vi "AlliGator.vi"() -> ()   [LabVIEW 2021, in "AlliGator GUI.lvlib"]
doc: "AlliGator main window.\nSpawned by AlliGator Launcher.vi.\nSpawns AlliGator Action Loop.vi, which handles UI requests from AlliGator.vi"
uses:
  AlliGator GUI.lvlib
  AlliGator Main Window Tabs.ctl
  Phasor/Phasor (g, s).ctl
  AlliGator Displayed Image.ctl
  AlliGator State Indicator.ctl
  Phasor/Phasor (m, phi).ctl
  Phasor/Phasor Ratio Type.ctl
  Fits/IRF(X)PSED/Decay Fit Parameters & Derived Quantities List.ctl
  Phasor/Phasor Calibration Type.ctl
  Histograms/Linear Histogram Options.ctl
  Histograms/Histogram Bin Option.ctl
  Histograms/Histogram Bin Position.ctl
  AlliGator Q Element.ctl
  AlliGator Q Event.ctl
  AlliGator Dataset Ctrl Refnums.ctl
  AlliGator Other Ctrl Refnums.ctl
  AlliGator Registered Events Ctrl Refnums.ctl
  AlliGator Ctrl Refnums.ctl
  AlliGator Phasor Plot Ctrl Refnums.ctl
  AlliGator Phasor Graph Ctrl Refnums.ctl
  AlliGator Image Histogram Control Refnums.ctl
  AlliGator Decay Fit Map Control Refnums.ctl
  AlliGator Refnums List.ctl
  AlliGator Settings List.ctl
  AlliGator Variables List.ctl
  Palette/Image Palette Information.ctl
  Image/Image Display Palette Type.ctl
  Image/Image Display Event.ctl
  Image/Image Control Refnum.ctl
  <vilib>/Utility/miscctls.llb/LVPoint32TypeDef.ctl
  AlliGator Decay Parameter Map Update Event Data.ctl
  Graphs/XY Graph/XY Graph Event.ctl
  AlliGator Filtered Event Data.ctl
  Utilities/Read-Write.ctl
  Graphs/XY Graph/New Plot Information.ctl
  Graphs/Plot Scales.ctl
  Graphs/LabVIEW Plot Interpolation.ctl
  Graphs/Plot Point Style.ctl
  Graphs/XY Graph/XY Graph Mouse Click Event Data.ctl
  Graphs/XY Graph/XY Graph Refnum.ctl
  AlliGator ROI Manager Actions.ctl
  Image/Image Display User Event Data.ctl
  AlliGator Phasor Plot Mouse Up Event Data.ctl
  Image/Image ROI Descriptor.ctl
  Image/Image Contour Definition.ctl
  Image/Image Contour ID.ctl
  Image/Image ROI Type.ctl
  AlliGator Action Loop.vi
  Variant/Variant to Data/Variant to Boolean.vi
  Phasor/Phasor Abort Parallel Computation.vi
  Fits/Abort Fit Global.vi
  Image/Abort ROI Creation Global.vi
  AlliGator Abort.vi
  Variant/Variant to Data/Variant to [String].vi
  <vilib>/Utility/inputDevices.llb/keyboardAcquire.vi
  <vilib>/Utility/inputDevices.llb/mouseAcquire.vi
  AlliGator Globals.vi
  <vilib>/Utility/inputDevices.llb/closeKeyboard.vi
  <vilib>/Utility/inputDevices.llb/closeMouse.vi
  AlliGator Action Engine.lvlib
  Variant/Variant to Data/Variant to Data.lvlib
  Error/Error.lvlib
  AlliGator Globals, Variables & Constants.lvlib
  Image/Image.lvlib
  Palette/Palette.lvlib
  Notebook/Notebook.lvlib
  Rich Text Box/Rich Text Box.lvlib
  Graphs/XY Graph/XY Graph Add-Ons.lvlib
  AlliGator Settings.lvlib
  Phasor/Phasor.lvlib
  Fits/Fits.lvlib
  AlliGator Phasor Calibration.lvlib
  AlliGator Phasor Plot.lvlib
  AlliGator Source Image.lvlib
  AlliGator Phasor Graph.lvlib
  AlliGator ROIs.lvlib
  GUI/GUI.lvlib
  AlliGator Decay Fit Parameter Map.lvlib
  AlliGator Python Plugins.lvlib
  Utilities/Utilities.lvlib
  AlliGator Graphs.lvlib
  Sound/Sound.lvlib
  Graphs/Graphs.lvlib
  AlliGator Decay Processing.lvlib
  Histograms/Histogram Window.lvlib
panel:
  in  "Current ROI Analysis":bool
  in  "Scale Bar":bool
  in  "Refresh Image":bool
  in  "Clear Image Overlay":bool
  in  "Overlay Mode":u16(ring)
  in  "Use ROI as Search Area":bool
  in  "Highlight Image ROI":bool
  in  "Phasor Overlay Color":u32(colorbox)=16777216
  in  "Gate Image Slide":u16(slide)=9 min=1 max=135 scale=1.0..132.0
  in  "Dataset File/Folder Path":path caption="File/Folder Path"
  out "Source Image":T1(plugin-control)
  in  "Source Image ROI Selection":i32(c297)
  in  "Source Image ROI Color":u32(colorbox)=6618880 caption="ROI Color"
  in  "Time Point Slide":u16(slide)=65535 min=1 step=1 scale=1.0..2.0
  in  "Image Color Scale":dbl(ramp)
  in  "Channel Name":u16(ring) items=["Gate"]
  out "Current Time Stamp":dbl caption="Time Stamp" format="%#_5g"
  out "CPU":dbl[unit] format="%^#_4e"
  in  "Save Source Image":bool caption="Save Image"
  out "Current Data":string="Stained cancer cells" caption="Current Folder"
  in  "Displayed Image":T2=enum."Sum of All Gates"
  in  "Tab Control":T3=enum."Lifetime & Other Parameters"
  in  "Dataset File/Folder Path 2":path caption="File/Folder Path"
  in  "Histogram Lower Percentile":dbl=1.0 caption="Lower Percentile" min=0.0 max=100.0 format="%#.3f"
  in  "Histogram Upper Percentile":dbl=1.0 caption="100 - Upper Percentile" min=0.0 max=100.0 format="%#.3f"
  in  "Image Histogram Options":T4={"Bin Size"=1.0, "Bin Number"=256, "Bin Option"=enum."Bin Number", "Min Value"=-inf, "Max Value"=inf, "Filter NaN & Infinite Values"=TRUE, "Frequency Plot"=FALSE, "Align Bins"=TRUE, "Bin Location"=enum."Left", "Project Outside Values"=FALSE, "Max Histogram Size"=1000000} {"Max Histogram Size" format="%.0e"}
  in  "Auto-Adjust Contrast":bool=TRUE
  out "Lower Percentile":dbl=nan format="%#.3f"
  out "Upper Percentile":dbl=nan caption="100 - Upper Percentile" format="%#.3f"
  in  "Image Histogram Active":bool=TRUE
  in  "Use Image Histogram for Contrast":bool=TRUE
  out "Image Histogram":cluster{"X Array":dbl[], "Y Array":dbl[]}[](graph)
  in  "Dataset File/Folder Path 3":path caption="File/Folder Path"
  out "Decay Integrated Intensity":dbl=46949635.0 caption="Bkgd-subtracted Intensity" format="%#_5g"
  out "Decay Background":dbl caption="Background" format="%#_5g"
  out "Decay Lifetime":dbl[unit] caption="Lifetime" format="%#_5g"
  out "Decay Graph TipStrip":string
  out "Decay Graph":cluster{"X Array":dbl[], "Y Array":dbl[]}[](graph)
  in  "Decay Graph Active":bool=TRUE
  in  "Dataset File/Folder Path 4":path caption="File/Folder Path"
  out "Decay Statistics Graph TipStrip":string
  out "Decay Statistics Graph":cluster{"X Array":dbl[], "Y Array":dbl[]}[](graph)
  in  "Decay Statistics Bin":i32=1 min=1
  in  "Dataset File/Folder Path 5":path caption="File/Folder Path"
  in  "Intensity Correction File":path
  in  "Use Intensity Correction File":bool
  out "Intensity Time Trace TipStrip":string
  in  "Use File Timestamp":bool=TRUE
  out "Intensity Time Trace":cluster{"X Array":dbl[], "Y Array":dbl[]}[](graph)
  in  "Time Step":dbl[unit]=1.0 format="%#_5g"
  in  "Dataset File/Folder Path 6":path caption="File/Folder Path"
  in  "Phasor ROI Decay":bool
  in  "Phasor Plot ROI Color":u32(colorbox)=6618880
  out "Phasor Plot Average Lifetime":dbl[unit]=nan caption="<tau>_a" format="%#_4e"
  out "Phasor Plot Phasor Ratio":dbl=nan caption="Amplitude Ratio (a1)" format="%#_4e"
  out "Phasor Plot Modulus Lifetime":dbl[unit]=nan caption="Modulus Lifetime" format="%#_4e"
  out "Phasor Plot Phase Lifetime":dbl[unit]=-9.431404035075279e-09 caption="Phase Lifetime" format="%#_4e"
  out "Phasor at cursor (m, phi)":T7={"m"=1.5330078000581284, "phi"=1.7786862539971595} caption="Phasor at Cursor (m, phi)" {"phi" format="%#_4e"; "m" format="%#_4e"}
  in  "Clear Phasor Overlay":bool
  in  "Phasor Plot ROI Selection":i32(c297)
  in  "Phasor Plot Active":bool
  in  "Phasor Plot Color Scale":dbl(ramp)
  out "Phasor at cursor (g, s)":T8={"g"=-0.31640625, "s"=1.5} caption="Phasor at Cursor" {"s" format="%#.3e"; "g" format="%#_4e"}
  in  "Phasor Plot Display Range":cluster{u32, u32}(slide)={0, 100} scale=0.0..6117.0
  in  "Highlight Phasor in Source Image":bool caption="Highlight Phasor ROI"
  in  "Image Overlay Color":u32(colorbox)=16777216
  out "Phasor Plot Image":T1(plugin-control)
  in  "Refresh Phasor Plot":bool caption="Refresh Phsor Plot"
  in  "Save Phasor Plot":bool
  out "Reference 2 Button":bool caption="Reference"
  out "Reference 1 Button":bool caption="Reference"
  in  "Phasor Plot Frequency":dbl[unit]=80000000.0 caption="Phasor Frequency"
  in  "Dataset File/Folder Path 7":path caption="File/Folder Path"
  out "Average Lifetime SDV":dbl[unit]=nan caption="+/-" format="%#.3g"
  out "Phasor Ratio SDV":dbl=nan caption="+/-" format="%#.3g"
  out "Modulus Lifetime SDV":dbl[unit]=nan caption="+/-" format="%#.3g"
  out "Phase Lifetime SDV":dbl[unit]=nan caption="+/-" format="%#.3g"
  in  "Calibration Type":T9
  out "Phasor Graph Average Lifetime":dbl[unit]=nan caption="<tau>_a" format="%#.3g"
  in  "Phasor Graph Active":bool
  in  "Refresh SEPL":bool
  out "Phasor Graph Phasor Ratio":dbl=nan caption="Amplitude Ratio (a1)" format="%#.3g"
  out "Phasor Graph Modulus Lifetime":dbl[unit]=nan caption="Modulus Lifetime" format="%#.3g"
  in  "Phasor Reference 2 Control":dbl(c297)
  in  "Save Phasor Graph Image":bool
  in  "Current Phasor (m, phi)":T7={"m"=nan, "phi"=nan} {"phi" format="%#_4g"; "m" format="%#_4g"}
  in  "Phasor Reference 1 Control":dbl(c297)
  out "Phasor Graph TipStrip":string
  in  "Single Step Phasor":bool
  in  "Phasor Frame Slide":i32(slide) caption="Phasor Frame Slider" min=0 step=1 scale=1.0..1.1
  out "Phase Lifetime 2":dbl[unit]=nan format="%#.3g"
  out "Phase Lifetime 1":dbl[unit]=nan format="%#.3g"
  in  "Show Line":bool
  out "Phasor Graph Phase Lifetime":dbl[unit]=nan caption="Phase Lifetime" format="%#.3g"
  in  "Current Phasor (g, s)":T8={"g"=nan, "s"=nan} caption="Current Phasor" {"s" format="%#_4g"; "g" format="%#_4g"}
  out "Phasor Graph":cluster{"X Array":dbl[], "Y Array":dbl[]}[](graph)
  in  "Phasor Graph Frequency":dbl[unit]=80000000.0 caption="Phasor Frequency"
  in  "Calibration Lifetime":dbl[unit] min=0.0
  in  "Dataset File/Folder Path 8":path caption="File/Folder Path"
  in  "Phasor Ratio Type":T10
  out "Phasor Ratio Graph TipStrip":string
  out "Phasor Ratio Graph":cluster{"X Array":dbl[], "Y Array":dbl[]}[](graph)
  in  "Dataset File/Folder Path 9":path caption="File/Folder Path"
  out "Lifetime & Other Parameters Graph TipStrip":string caption="Lifetime Graph TipStrip"
  out "Lifetime & Other Parameters Graph":cluster{"X Array":dbl[], "Y Array":dbl[]}[](graph)
  in  "Dataset File/Folder Path 10":path caption="File/Folder Path"
  in  "Decay Fit Parameter Map ROI Color":u32(colorbox)=6618880
  in  "Overlay Decay Fit Parameter Map":bool caption="Overlay Parameter Map"
  out "Decay Fit Max Parameter":dbl=1.0 caption="Max Parameter"
  out "Decay Fit Min Parameter":dbl caption="Min Parameter"
  in  "Refresh Decay Fit Parameter Map":bool
  in  "Decay Fit Parameter":T11
  out "Decay Fit Parameter Map Image":T1(plugin-control)
  in  "Decay Fit Parameter Map Color Scale":dbl(ramp)
  in  "Decay Fit Parameter Map Display Range":cluster{dbl, dbl}(slide)={0.0, 1.0} scale=0.0..1.0
  in  "Map Set":u16(ring)
  in  "Map Parameter":u16(ring)
  in  "Dataset File/Folder Path 11":path caption="File/Folder Path"
  in  "Parameter Map ROI Color":u32(colorbox)=6618880 caption="Decay Fit Parameter Map ROI Color"
  in  "Overlay Parameter Map":bool
  out "Map Max Parameter":dbl=1.0 caption="Max Parameter"
  out "Map Min Parameter":dbl caption="Min Parameter"
  in  "Refresh Parameter Map":bool
  out "Parameter Map Image":T1(plugin-control)
  in  "Parameter Map Color Scale":dbl(ramp)
  in  "Parameter Map Display Range":cluster{dbl, dbl}(slide)={0.0, 1.0} scale=0.0..1.0
  out "Event LED":bool
  out "Message":string
  out "Progress Bar":dbl(slide) scale=0.0..100.0
  in  "Abort ROI Creation":bool
  in  "Abort Fit":bool
  in  "Abort":bool
  out "Animated Busy Icon":bool=TRUE
  out "State Indicators":T12
  # "Drop the content of this VI on AlliGator's diagram\nIn AlliGator, replace the subVI template by a new version"
  # "Drop the content of this VI on AlliGator's diagram\nIn AlliGator, replace the subVI template by a new version"
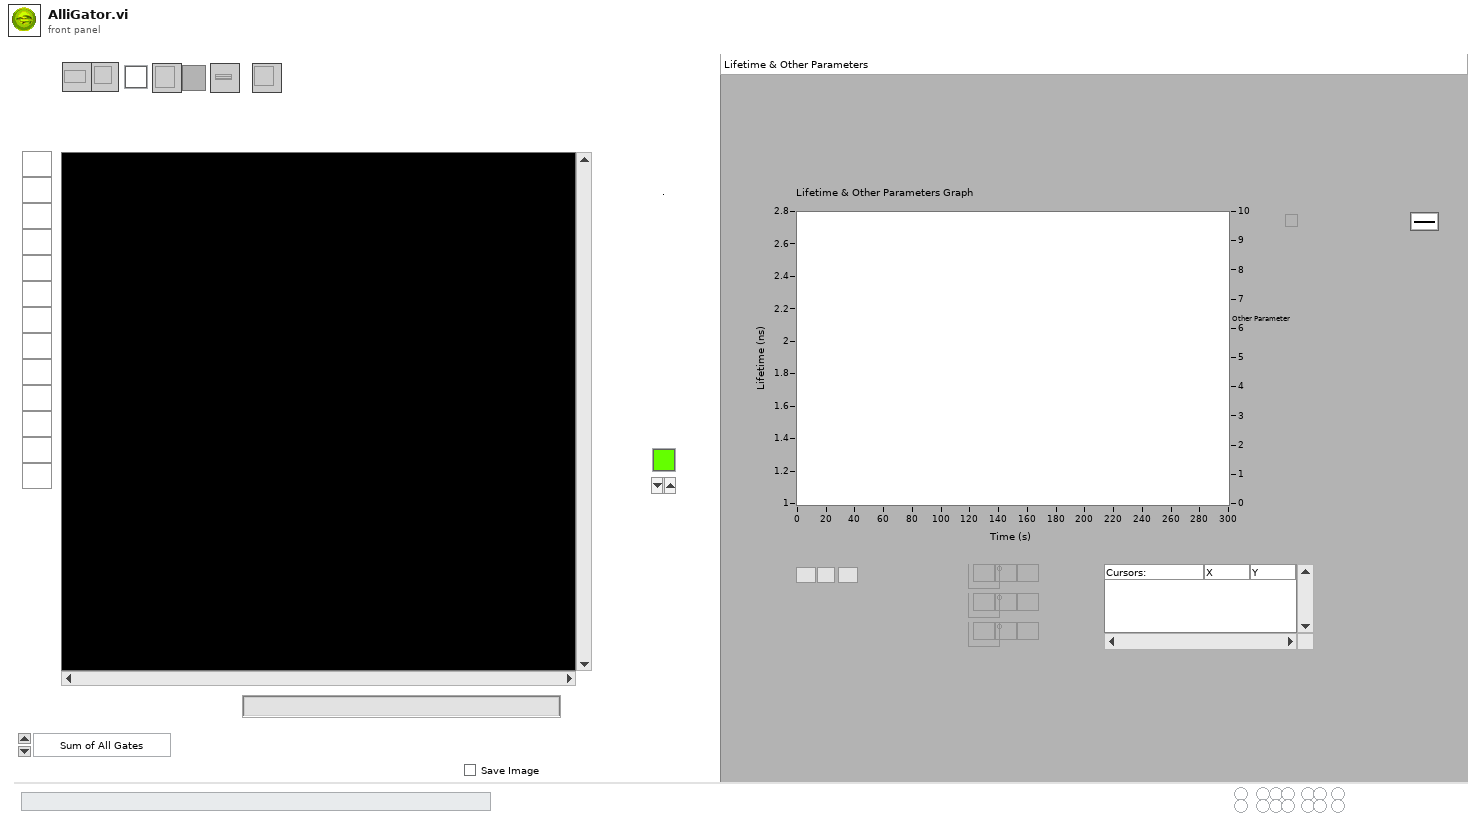
[diagram p1: front panel]
types:
  T1 = typedef "IMAQ Image.ctl" = refnum<image>
  T2 = typedef "AlliGator Source Image.lvlib/AlliGator Displayed Image.ctl" = enum16{"Single Gate", "Sum of All Gates", "Max of All Gates", "Min of All Gates", "-", "White Ligth Image", "Mask Image"}
  T3 = typedef "AlliGator GUI.lvlib/AlliGator Main Window Tabs.ctl" = enum32{"Image Histogram", "Fluorescence Decay", "Fluorescence Decay Statistics", "Intensity Time Trace", "Phasor Plot", "Phasor Graph", "Phasor Ratio", "Lifetime & Other Parameters", "Decay Fit Parameter Map", "Parameter Map"}
  T4 = typedef "Histogram Window.lvlib/Linear Histogram Options.ctl" = cluster{"Bin Size":dbl, "Bin Number":i32, "Bin Option":T5, "Min Value":dbl, "Max Value":dbl, "Filter NaN & Infinite Values":bool, "Frequency Plot":bool, "Align Bins":bool, "Bin Location":T6, "Project Outside Values":bool, "Max Histogram Size":i32}
  T5 = typedef "Histogram Window.lvlib/Histogram Bin Option.ctl" = enum32{"Bin Number", "Bin Size"}
  T6 = typedef "Histogram Window.lvlib/Histogram Bin Position.ctl" = enum16{"Left", "Center", "Right"}
  T7 = typedef "Phasor.lvlib/Phasor (m, phi).ctl" = cluster{"m":dbl, "phi":dbl}
  T8 = typedef "Phasor.lvlib/Phasor (g, s).ctl" = cluster{"g":dbl, "s":dbl}
  T9 = typedef "Phasor.lvlib/Phasor Calibration Type.ctl" = enum16{"None", "Single Phasor", "Phasor Series", "Phasor Map"}
  T10 = typedef "Phasor.lvlib/Phasor Ratio Type.ctl" = enum32{"Intensity-weighted", "Amplitude-weighted"}
  T11 = typedef "Fits.lvlib/Decay Fit Parameters & Derived Quantities List.ctl" = enum16{"Offset", "Baseline", "A_1", "tau_1", "A_2", "tau_2", "<tau>_a", "f1_a", "f2_a", "<tau>_i", "f1_i", "f2_i", "-", "R^2", "Chi^2"}
  T12 = typedef "AlliGator GUI.lvlib/AlliGator State Indicator.ctl" = cluster{"Phasor Calibration Defined":bool, "Phasor Calibration Series Defined":bool, "Phasor Calibration Map Defined":bool, "Phasor Ratio Reference 1 Defined":bool, "Phasor Ratio Reference 2 Defined":bool, "Phasor Ratio Lifetime Reference 1 Defined ":bool, "Phasor Ratio Lifetime Reference 2 Defined":bool, "Phasor Calibration Used":bool, "Phasor Calibration Series Used":bool, "Phasor Calibration Map Used":bool, "Dataset Update Needed":bool, "Phasor Plot Update Needed":bool, "Reference/IRF Defined":bool, "Individual IRFs Defined":bool}
  T13 = enum32{"Invalid", "Standard", "Closed", "Hidden", "Minimized", "Maximized"}
  T14 = enum32{"Image Histogram", "Fluorescence Decay", "Fluorescence Decay Statistics", "Intensity Time Trace", "Phasor Plot", "Phasor Graph", "Phasor Ratio", "Lifetime & Other Parameters", "Decay Fit Parameters Map", "Parameter Map"}
  T15 = typedef "AlliGator Decay Fit Parameter Map.lvlib/AlliGator Decay Fit Map Control Refnums.ctl" = cluster{"Decay Fit Parameter Map Color Scale":refnum<vi>, "Decay Fit Parameter":refnum<vi>, "Max Parameter":refnum<vi>, "Min Parameter":refnum<vi>, "Decay Fit Parameter Map Display":refnum<vi>, "Decay Fit Parameter Map Display Range":refnum<vi>}
  T16 = typedef "AlliGator GUI.lvlib/AlliGator Image Histogram Control Refnums.ctl" = cluster{"Image Histogram":refnum<vi>, "Image Histogram Options":refnum<vi>, "Image Histogram Active":refnum<vi>, "Image Histogram Upper Percentile":refnum<vi>, "Image Histogram Lower Percentile":refnum<vi>, "Auto-Adjust Contrast":refnum<vi>}
  T17 = typedef "AlliGator GUI.lvlib/AlliGator Phasor Graph Ctrl Refnums.ctl" = cluster{"Phasor Ratio":refnum<vi>, "Modulus Lifetime":refnum<vi>, "Phasor at cursor (m, phi)":refnum<vi>, "Phase Lifetime":refnum<vi>, "Phasor at cursor (g, s)":refnum<vi>, "Phasor Graph Average Lifetime":refnum<vi>, "Phasor Graph Active":refnum<vi>, "Save Phasor Graph":refnum<vi>, "Phasor Frame Slide":refnum<vi>, "Single Step Phasor":refnum<vi>, "Calibration Type":refnum<vi>, "Show Line":refnum<vi>, "Phase Lifetime 1":refnum<vi>, "Phase Lifetime 2":refnum<vi>, "Phasor Graph Frequency":refnum<vi>, "Phasor Reference 1 Control":refnum<vi>, "Phasor Reference 2 Control":refnum<vi>, "Calibration Lifetime":refnum<vi>, "Phase Lifetime SDV":refnum<vi>, "Average Lifetime SDV":refnum<vi>, "Phasor Ratio SDV":refnum<vi>, "Modulus Lifetime SDV":refnum<vi>}
  T18 = typedef "AlliGator GUI.lvlib/AlliGator Phasor Plot Ctrl Refnums.ctl" = cluster{"Phasor Ratio":refnum<vi>, "Modulus Lifetime":refnum<vi>, "Phasor at cursor (m, phi)":refnum<vi>, "Phase Lifetime":refnum<vi>, "Phasor at cursor (g, s)":refnum<vi>, "Phasor Plor Average Lifetime":refnum<vi>, "Phasor Plot Active":refnum<vi>, "Save Phasor Plot":refnum<vi>, "Image Overlay Color":refnum<vi>, "Phasor Plot Color Scale":refnum<vi>, "Reference 1 Button":refnum<vi>, "Reference 2 Button":refnum<vi>}
  T19 = typedef "AlliGator Globals, Variables & Constants.lvlib/AlliGator Refnums List.ctl" = enum16{"---------- AlliGator Controls ----------", "AlliGator Tab Control Refnum", "---------- AlliGator Indicators ----------", "Source Image Display Refnum", "Phasor Plot Display Refnum", "Decay Fit Parameter Map Refnum", "---------- AlliGator VIs ----------", "AlliGator Settings Refnum", "AlliGator Launcher Refnum"}
  T20 = typedef "AlliGator GUI.lvlib/AlliGator Ctrl Refnums.ctl" = cluster{"Other AlliGator Ctrl Refnums":T21, "Phasor Plot Ctrl Refnums":T18, "Phasor Graph Ctrl Refnums":T17, "Dataset Control References":T22, "Registered Events Ctrl Refnums":T23, "Image Histogram Ctrl Refnums":T16, "Decay Fit Map Ctrl Refums":T15}
  T21 = typedef "AlliGator GUI.lvlib/AlliGator Other Ctrl Refnums.ctl" = cluster{"State Indicators":refnum<vi>, " Progress Bar":refnum<vi>, "Decay Graph Active":refnum<vi>, "Decay Statistics Bin":refnum<vi>, "Time Step":refnum<vi>, "Use File Timestamp":refnum<vi>, "Tab Control":refnum<vi>, "CPU":refnum<vi>, "Abort Fit":refnum<vi>, "Dataset File/Folder Path":refnum<vi>, "Abort ROI Creation":refnum<vi>, "Event LED":refnum<vi>, "Dataset File/Folder Path 2":refnum<vi>, "Dataset File/Folder Path 3":refnum<vi>, "Dataset File/Folder Path 4":refnum<vi>, "Dataset File/Folder Path 5":refnum<vi>, "Dataset File/Folder Path 6":refnum<vi>, "Dataset File/Folder Path 7":refnum<vi>, "Dataset File/Folder Path 8":refnum<vi>, "Dataset File/Folder Path 9":refnum<vi>, "Dataset File/Folder Path 10":refnum<vi>, "Dataset File/Folder Path 11":refnum<vi>}
  T22 = typedef "AlliGator GUI.lvlib/AlliGator Dataset Ctrl Refnums.ctl" = cluster{"Current Data":refnum<vi>, "Gate Image Slide":refnum<vi>, "Time Point Slide":refnum<vi>, "Current Time Stamp":refnum<vi>, "Save Image":refnum<vi>, "Displayed Image":refnum<vi>, "Overlay Mode":refnum<vi>, "Phasor Overlay Color":refnum<vi>, "Image Color Scale":refnum<vi>, "Use ROI as Search Area":refnum<vi>, "Source Image ROI Color":refnum<vi>}
  T23 = typedef "AlliGator GUI.lvlib/AlliGator Registered Events Ctrl Refnums.ctl" = cluster{"Time Point Slider":refnum<vi>, "Phasor Plot Display Range":refnum<vi>, "Decay Graph":refnum<vi>, "Decay Statistics Graph":refnum<vi>, "Intensity Time Trace":refnum<vi>, "Phasor Graph":refnum<vi>, "Phasor Ratio Graph":refnum<vi>, "Lifetime Graph":refnum<vi>, "Phasor Plot Display":refnum<vi>, "Source Image Display":refnum<vi>, "Decay Fit Parameter Map Display Range":refnum<vi>, "Decay Fit Parameter Map Display":refnum<vi>}
  T24 = typedef "AlliGator Action Engine.lvlib/AlliGator Q Event.ctl" = enum16{"---- Files ----", "Files:Set Batch Export Files To Save", "Files:Set Dataset Loading & Pre-processing Options", "Files:Check #Frames in Dataset", "Files:Increment Frame Index", "Files:Open Mask Image", "Files:Open White Light Image", "Files:Open Single Dataset", "Files:New Folder of Folders Selected", "Files:Load File (all Types)_Scriptable", "Files:Move Flattened Series to Folders Series", "Files:Select Folder", "Files:Load FLI Dataset", "Files:Load Swiss SPAD 1 Dataset", "Files:Load Swiss SPAD 2 Dataset", "Files:Load .sdt FLI Dataset", "Files:Load .ptu FLI Dataset", "Files:Load .bin FLI Dataset", "Files:Load Single Gate Image Folder", "Files:Load I/m/phi Dataset (deprecated)", "Files:Load Single Image", "Files:Subtract Background File", "Files:Export FLI Dataset", "Files:Load HDF5 FLI Dataset", "Files:Set Destination File Path", "Files:Save Mask Image", "Files:Batch Conversion", "Files:New Folder Selected", "Files:Close FLI Dataset", "Files:Close FLI Dataset Series", "Files:Close White Light Image", "Files:Close Mask Image", "---- FLI Dataset ----", "FLI Dataset:Channel Arithmetic", "FLI Dataset:Export Average Lifetime Map as ASCII", "FLI Dataset:Export User-Defined Quantity Map as ASCII", "FLI Dataset:Python Function FLI Dataset Event", "FLI Dataset:ROI Analysis", "FLI Dataset:Tilted Logistic Square Gated IRF Characteristics Map", "FLI Dataset:Logistic Square Gated IRF Characteristics Map", "FLI Dataset:Square Gated IRF Characteristics Map", "FLI Dataset:Multi-ROI Single-Pixel Phasor Analysis", "FLI Dataset:Multi-ROI Single-Pixel NLSF Analysis", "FLI Dataset:All ROIs IRF Extraction", "FLI Dataset:All ROIs Decay Fit Non-Interactive (Fast + Individual IRF)", "FLI Dataset:All ROIs Phasor Analysis", "FLI Dataset:All ROIs Decay Fit", "FLI Dataset:Fluorescence Decay Statistics", "FLI Dataset:Update Decay Statistics Graph", "FLI Dataset:Get Decay from ROI", "FLI Dataset:All ROIs Average Lifetimes", "---- FLI Dataset Series ----", "FLI Dataset Series:Sum All Datasets in Series", "FLI Dataset Series:Add Dataset to Accumulated Dataset", "FLI Dataset Series:Display Accumulated Dataset", "FLI Dataset Series:Clear Dataset Series Sum", "FLI Dataset Series:Time-Series Analysis (NLSF)", "FLI Dataset Series:Time-Series Analysis (Phasor)", "---- Image ----", "Image:Update Image Profile Plots", "Image:Image Histogram Cursor Move", "Image:Image Histogram", "Image:Image Contrast", "Image:Set Image Histogram Cursor Move Flag", "Image:Clear Image Overlay", "Image:Use ROI as Search Area", "Image:Set ROI Diameter", "Image:Save Image Data as TIFF", "Image:Save Displayed Image with Overlay", "Image:Save Image Overlay Only", "Image:Save Image as Hot Pixel Mask", "Image:Change Source Image Color Palette", "Image:Copy Image to Clipboard", "Image:Source Image ROI Selection", "Image:Delete All ROIs", "Image:Delete All Unselected ROIs", "Image:Delete ROI", "Image:Merge All ROIs", "Image:Store ROI", "Image:Source Image ROI Storage", "Image:Export ROI Description to Notebook", "Image:Save ROI", "Image:Load ROI", "Image:Paste ROI Definition", "Image:Clear ROI", "Image:Identify ROIs in Mask Image", "Image:Create Complementary ROI", "Image:Create Contour ROI", "Image:Create ROI(s) from Pixels with Peak above Min_Scriptable", "Image:Create ROI(s) from Pixels with Intensity above Min_Scriptable", "Image:Compute ROI Statistics", "Image:Delete ROI(s) based on ROI Characteristics", "Image:Create ROI Grid", "Image:ROI to Individual Pixel ROIs", "Image:Python Function Source Image Event", "Image:Show Phasor Calibration Map ROI Centers", "Image:Convert ROI to Mask Image", "Image:Mouse Move", "Image:Mouse Up", "Image:Set Source Image Mouse Move Flag", "Image:Add Scale Bar Overlay", "Image:Delete Existing ROIs Option", "Image:Overlay ROI Median", "---- Decay ----", "Decay:Clear IRF/Reference Plot", "Decay:Clear Local IRFs", "Decay:Add Decay to Graph", "Decay:Smoothen Plot", "Decay:Smoothen Plot Tail", "Decay:Average Selected Plots", "Decay:Extract IRF", "Decay:Optimal IRF Extraction", "Decay:Threshold IRF", "Decay:Fit to Model IRF", "Decay:Fit IRF to Square Gate", "Decay:Fit IRF to Logistic Square Gate", "Decay:Fit IRF to Tilted Logistic Square Gate", "Decay:Create Bounding Cursors Set", "Decay:Export Bounding Cursors Definition to Notebook", "Decay:Denoise Plot", "Decay:Compute Cumulative Function", "Decay:Use as Reference Decay", "Decay:Show Reference Decay/IRF", "Decay:Extrapolate Decay", "Decay:Create Head & Tail Bounding Cursors", "Decay:Store Cursor-defined Head & Tail Fractions", "Decay:Rebin Plot", "Decay:1-Normalize Decay", "Decay:[0-1]-Normalize Plot", "Decay:Straighten Decay", "Decay:Shift Decay", "Decay:Fold Decay", "Decay:Fit Decay", "Decay:Global Fit of Selected Decays", "Decay:Post Global Fit Script", "Decay:Add Global Fit Parameters to Graph", "Decay:Add Decay Parameter(s) to Plot (Graph)", "Decay:Export Decay to Phasor Graph", "Decay:Plot Decay Shifts", "Decay:Compute Average Lifetime", "Decay:Plot Convolution", "Decay:Graph Tip Strip Update", "---- Decay Statistics ----", "Decay Statistics:Tip Strip Update", "---- Intensity Time Trace ----", "Intensity Time Trace:Use File Timestamp", "Intensity Time Trace:Load Intensity Corrections File", "Intensity Time Trace:Clear Intensity Corrections File", "Intensity Time Trace:Tip Strip Update", "---- Phasor Plot ----", "Phasor Plot:Build Phasor Plot", "Phasor Plot:Change Phasor Plot Color Palette", "Phasor Plot:Adjust Phasor Plot Display Range", "Phasor Plot:Highlight Image ROI in Phasor Plot", "Phasor Plot:Save Phasor Plot Image with Overlay", "Phasor Plot:Export Complex Phasor Map", "Phasor Plot:Export Phasor Ratio Map", "Phasor Plot:Export Average Lifetime Map", "Phasor Plot:Compute Phase Lifetime Histogram", "Phasor Plot:Compute Phasor Ratio Histogram", "Phasor Plot:Compute Phase Lifetime vs Intensity Scatter Plot", "Phasor Plot:Weber 2-Component Decomposition", "Phasor Plot:Update Phasor Color Map Vertices", "Phasor Plot:Clear Phasor Overlay", "Phasor Plot:Use Segment Extremities as References", "Phasor Plot:Use UC/Segment Intersections as References", "Phasor Plot:Use UC/Principal Axis Intersections as References", "Phasor Plot:Use UC/Linear Fit Intersections as References", "Phasor Plot:Update Phasor Plot Reference", "Phasor Plot:Show Local Phasor Info in Phasor Plot", "Phasor Plot:Update Phasor Plot State", "Phasor Plot:Phasor Plot ROI Storage", "Phasor Plot:Phasor Plot ROI Selection", "Phasor Plot:Python Function Phasor Plot Event", "Phasor Plot:Overlay Phasor ROI, Ratio or Map in Source Image", "Phasor Plot:Compute Decay of Selected Phasors", "Phasor Plot:Phasor at Image Pixel", "Phasor Plot:Mouse Move", "Phasor Plot:Mouse Up", "Phasor Plot:Display Range Mouse Move", "Phasor Plot:Set Mouse Move Flag", "---- Phasor Graph ----", "Phasor Graph:Calibrated Phasor Map Series", "Phasor Graph:Whole Image Phasor Scatter Plot (Todo)", "Phasor Graph:Get Phasor Value", "Phasor Graph:Create New Phasor Plot Dialog", "Phasor Graph:Update Last Phasor Value", "Phasor Graph:Update Phasor (m, phi)", "Phasor Graph:Remove Single Phasor from Plot", "Phasor Graph:Add Single Phasor to Plot", "Phasor Graph:Remove Phasor Plot", "Phasor Graph:Remove Selected Phasor Plots", "Phasor Graph:Clear Phasor Data", "Phasor Graph:Clear Phasor Graph", "Phasor Graph:Cursor Move", "Phasor Graph:Draw Cursor Connecting Line", "Phasor Graph:Clear Cursor Connecting Line", "Phasor Graph:Find UC Intersection", "Phasor Graph:Use UC/Cursor-Defined Line Intersections", "Phasor Graph:Use Selected Plots Fitted Line/UC Intersections", "Phasor Graph:Use Selected Plots Principal Axis/UC Intersections", "Phasor Graph:Show Single Phasor", "Phasor Graph:Save Single Phasor Plot", "Phasor Graph:Save All Phasor Plots", "Phasor Graph:Load Phasor Plot(s)", "Phasor Graph:Phasor Multiplication", "Phasor Graph:Compute Average Phasor", "Phasor Graph:Compute Multiple Average Phasors (Selected Plots)", "Phasor Graph:Export Single Phasor Plot Phase Lifetimes", "Phasor Graph:Phase Lifetime Trajectory", "Phasor Graph:Phase Lifetime vs Intensity Scatter Plot (deprecated)", "Phasor Graph:Parameter 2 vs Parameter 1 Scatter Plot", "Phasor Graph:Use Cursor n Location", "Phasor Graph:Set Reference n to Current Phase Lifetime Value", "Phasor Graph:Set Reference n to Lifetime Value", "Phasor Graph:Set Cursor n Location", "Phasor Graph:Save Phasor Graph Image", "Phasor Graph:Update SEPL Plot", "Phasor Graph:Export Single Phasor Plot Data", "Phasor Graph:Export Selected Phasor Plots Data", "Phasor Graph:Python Function Phasor Graph Event", "Phasor Graph:Tip Strip Update", "---- Calibration ----", "Calibration:Set Calibration Type", "Calibration:Load/Save Phasor Calibration", "Calibration:Load/Save Phasor Calibration Series", "Calibration:Load/Save Phasor Calibration Map", "Calibration:Use as Calibration", "Calibration:Compute Optimal Calibration from Phasor References", "Calibration:Clear Phasor Calibration", "Calibration:Single Phasor Calibration Information", "Calibration:Use as Calibration Series", "Calibration:Use as Calibration Map", "Calibration:Clear Calibration Series", "Calibration:Phasor Calibration Series Information", "Calibration:Clear Calibration Map", "Calibration:Phasor Calibration Map Information", "Calibration:Apply Phasor Calibration", "Calibration:Update Single Plot Calibration", "Calibration:Update Multiple Plots Calibration", "Calibration:Clear Single Plot Calibration", "Calibration:Clear All Plots Calibrations", "Calibration:Clear Plot(s) Calibration(s)?", "Calibration:Phasor Calibration Maps (# Gates Series)", "---- Phasor Ratio ----", "Phasor Ratio:Clear Reference n", "Phasor Ratio:Toggle Selected Plot(s)  Lock to Reference 1", "Phasor Ratio:Use as Reference n", "Phasor Ratio:Send Reference n to Notebook", "Phasor Ratio:Toggle Selected Plot(s)  Lock to Reference 2", "Phasor Ratio:Compute Phasor Ratio at Mouse Location", "Phasor Ratio:Compute Phasor Plot's Average Phasor Ratio", "Phasor Ratio:Compute Time-Series Phasor Ratios", "Phasor Ratio:Fit Line to Phasor Ratio Plot", "Phasor Ratio:Save References", "Phasor Ratio:Load References", "Phasor Ratio:Update Phasor Reference 1", "Phasor Ratio:Update Phasor Reference 2", "Phasor Ratio:Move Cursor n to Reference n", "Phasor Ratio:Use as Phasor Reference 1 Lifetime", "Phasor Ratio:Use as Phasor Reference 2 Lifetime", "Phasor Ratio:Export Phasor Ratio Map as ASCII", "Phasor Ratio:Tip Strip Update", "---- Lifetime & Other Parameters Graph ----", "Lifetime:Tip Strip Update", "---- Decay Fit Parameter Map ----", "Decay Fit Parameter Map:Export ROI NLSF Data as ASCII", "Decay Fit Parameter Map:Set Decay Fit  Parameter Map Selection", "Decay Fit Parameter Map:Build Decay Fit Parameter Map", "Decay Fit Parameter Map:Change Decay Fit Parameter Map Color Palette", "Decay Fit Parameter Map:Export Decay Fit Parameter Map Data as ASCII", "Decay Fit Parameter Map:Export All Decay Fit Parameter Maps Data as ASCII", "Decay Fit Parameter Map:Send Map Data to Lifetime Graph", "Decay Fit Parameter Map:Save Decay Fit Parameter Map Image", "Decay Fit Parameter Map:Save-Load IRFs & Fit Data", "Decay Fit Parameter Map:Update Local Decay Plots", "Decay Fit Parameter Map:Python Function Decay Fit Parameters Map Event", "Decay Fit Parameter Map:Overlay Decay Fit Parameter Map in Source Image", "Decay Fit Parameter Map:Plot Map Data vs Intensity", "Decay Fit Parameter Map:Mouse Up", "Decay Fit Parameter Map:Display Range Mouse Move", "---- Generic Graph ----", "Generic Graph:Generic XY Graph Event", "Generic Graph:Python Function XY Graph Event", "Generic Graph:New Plot", "Generic Graph:Save Plot", "Generic Graph:XY Plot Histogram", "Generic Graph:Set XY Graph Plot Name", "Generic Graph:Set Last Cursor Style", "Generic Graph:Tip Strip Update", "---- GUI ----", "GUI:Start Script", "GUI:Type of Displayed Image Changed", "GUI:Gate Image Slide Changed", "GUI:Show Busy Icon", "GUI:Show Busy Icon & Abort Button", "GUI:Hide Busy Icon", "GUI:Hide Busy Icon & Abort Button", "GUI:Abort", "GUI:End Script", "GUI:Start Timing", "GUI:End Timing", "GUI:Set State Indicator", "GUI:Send Parameters JSON Strings to Clipboard", "GUI:Set Gate Step", "GUI:Idle", "GUI:Initialization", "GUI:Quit", "GUI:Increment Dataset Index", "GUI:Set Dataset Index to -1", "GUI:Time Series Slider Moved", "GUI:Time Series Slider Changed", "GUI:Toggle Playback or Loop", "GUI:Playback Script", "GUI:Set Phasor Frequency", "GUI:Open Window", "GUI:Start Test Script", "GUI:End Test Script", "DEBUG"}
  T25 = typedef "AlliGator Action Engine.lvlib/AlliGator Q Element.ctl" = cluster{"AlliGator Q Event":T24, "Data":variant}
  T26 = typedef "AlliGator GUI.lvlib/AlliGator Event Registration v2.ctl" = cluster{"Phasor Plot Display Event":refnum<event-registration>, "Source Image Display Event":refnum<event-registration>, "Phasor Display Range Event":refnum<event-registration>, "Time Point Slider Event":refnum<event-registration>, "Other Events":refnum<event-registration>, "Decay Graph Tipstrip Event":refnum<event-registration>, "Decay Statistics Graph Tipstrip Event":refnum<event-registration>, "Intensity Time Trace Tipstrip Event":refnum<event-registration>, "Phasor Graph Tipstrip Event":refnum<event-registration>, "Phasor Ratio Graph Tipstrip Event":refnum<event-registration>, "Lifetime Graph Tipstrip Event":refnum<event-registration>, "Decay Fit Parameter Map Display Range Event":refnum<event-registration>, "Decay Fit Parameter Map Display Event":refnum<event-registration>}
  T27 = typedef "AlliGator Progress Bar Q Element.ctl" = cluster{"Action":string, "Value":dbl}
  T28 = typedef "AlliGator Settings.lvlib/AlliGator Settings List.ctl" = enum16{"GUI:Visible Settings Tab", "GUI:Last Run Version", "Source Image:Use Image Histogram for Contrast", "Source Image:Low Count Pixels Rejection Options", "Source Image:High Count Pixels Rejection Options", "Source Image:Use Image Brightness", "Source Image:Blend Overlay with Image Background", "Source Image:Use Fixed ROI Diameter", "Source Image:ROI Diameter", "Source Image:ROI Center Color", "Source Image:Peak Threshold", "Source Image:Intensity Threshold", "Source Image:Image Binning Options", "Source Image:Image Smoothing Options", "Source Image:Image Histogram Active", "Source Image:Invert Binary Mask", "Source Image:Hot Pixel Removal", "Source Image:Overlay Analyzed ROI Center", "Source Image:Auto-Adjust Contrast", "Source Image:Histogram Lower Percentile", "Source Image:Histogram Upper Percentile", "Source Image:Save Source Image", "Source Image:Scale Bar Options", "Source Image:Image Resolution (Pixel Size)", "Source Image:Flatfield Correction", "Source Image:Show Dead Left Columns Correction", "Source Image:Dead Left Columns Correction", "Source Image:Image Pre-Processing Operations Order", "Source Image:Overlay ROI Median", "Source Image:Median Overlay Color", "Data Information:Gate Width", "Data Information:Nanotime Gate Separation", "Data Information:Macrotime Gate Separation", "Data Information:Gate Step", "Data Information:# Gates", "Data Information:Gate Image Exposure", "Data Information:Gate Image Integration", "Data Information:Gates to Skip", "Data Information:Gates to Keep", "Data Information:Define Gates to", "Data Information:Channel Name", "Data Information:Available Channel Names", "Data Information:Channel Arithmetic", "Data Information:Background File Subtraction", "Data Information:Background File", "Data Information:Background Scaling Factor", "Data Information:Background Pile-up Correction", "Data Information:Background Pixel Well Capacity", "Data Information:Laser Period", "Data Information:SYNC Period", "Data Information:Pile-up Correction", "Data Information:Pixel Well Capacity", "Data Information:Dataset Scaling Factor", "Fluorescence Decay_Decay Pre-Processing:Reverse Gates", "Fluorescence Decay_Decay Pre-Processing:Verbose Decay Pre-Processing", "Fluorescence Decay_Decay Pre-Processing:Use Decay Pre-Processing", "Fluorescence Decay_Decay Pre-Processing:Background Subtraction", "Fluorescence Decay_Decay Pre-Processing:Background Definition Range", "Fluorescence Decay_Decay Pre-Processing:Baseline Subtraction Method", "Fluorescence Decay_Decay Pre-Processing:Decay Pre-Processing Operations Order", "Fluorescence Decay_Decay Pre-Processing:Smoothing Parameter", "Fluorescence Decay_Decay Pre-Processing:Shift Decay", "Fluorescence Decay_Decay Pre-Processing:Decay Shift Parameters", "Fluorescence Decay_Decay Pre-Processing:Fold Decay", "Fluorescence Decay_Decay Pre-Processing:# Folds", "Fluorescence Decay_Decay Pre-Processing:1-Normalize Decay", "Fluorescence Decay_Decay Pre-Processing:[0-1]-Normalize Decay", "Fluorescence Decay_Decay Pre-Processing:Smoothen Decay", "Fluorescence Decay_Decay Pre-Processing:Extrapolate Decay", "Fluorescence Decay_Decay Pre-Processing:Use Periodicity", "Fluorescence Decay_Decay Pre-Processing:Use Cursors", "Fluorescence Decay_Decay Pre-Processing:Tail Fraction", "Fluorescence Decay_Decay Pre-Processing:Head Fraction", "Fluorescence Decay_Decay Pre-Processing:Additional Points", "Fluorescence Decay_Decay Pre-Processing:Straighten Decay", "Fluorescence Decay_Decay Pre-Processing:Constant Background", "Fluorescence Decay_Decay Pre-Processing:Pixel-Normalize Decay", "Fluorescence Decay_Advanced Analysis:Extract IRF instead of Decay", "Fluorescence Decay_Advanced Analysis:IRF Extraction Options", "Fluorescence Decay_Advanced Analysis:IRF Optimization Options", "Fluorescence Decay_Advanced Analysis:Square Pulse Options", "Fluorescence Decay_Advanced Analysis:IRF Order", "Fluorescence Decay_Advanced Analysis:IRF Time Constants", "Fluorescence Decay_Advanced Analysis:Wavelet Analysis Options", "Fluorescence Decay_Advanced Analysis:Average Lifetime Options", "Fluorescence Decay_Fit Options:Fit Options", "Fluorescence Decay_Fit Options:Use Legacy Fitting Approach", "Fluorescence Decay_Fit Options:Use Data Information Laser Period", "Fluorescence Decay_Fit Parameters:Displayed Fit Parameters", "Fluorescence Decay_Fit Parameters:Fit Parameter Constraints", "Fluorescence Decay_Fit Parameters:Export Tabulated Results", "Fluorescence Decay_Fit Parameters:MLE Baseline Offset Type", "Fluorescence Decay_Fit Parameters:MLE Baseline Offset", "Fluorescence Decay_Fit Parameters:Guess Parameter Names", "Fluorescence Decay_Fit Parameters:Guess Parameter Values", "Fluorescence Decay_Fit Parameters:Guess Parameters Options", "Fluorescence Decay_Styles:Show Last Decay Only", "Fluorescence Decay_Styles:Decay Graph Color Array", "Fluorescence Decay:Decay Graph Active", "Fluorescence Decay Statistics:Min Peak Value", "Fluorescence Decay Statistics:Reject Low Decay Peak Pixels", "Fluorescence Decay Statistics:Reject High Decay Peak Pixels", "Fluorescence Decay Statistics:Max Peak Value", "Time Traces:Use File Timestamp", "Time Traces:Time Step", "Time Traces:Use Intensity Correction File", "Time Traces:Intensity Correction File", "Phasor Plot:Phasor Plot Smoothing Options", "Phasor Plot:Phasor Plot Size", "Phasor Plot:Phasor Plot Graphics Options", "Phasor Plot:Cumulative Phasor Plot", "Phasor Plot:Use Phasor Brightness", "Phasor Plot:Blend Overlay with Phasor Background", "Phasor Plot:Save Phasor Plot", "Phasor Plot:Show References", "Phasor Plot:Phasor Ratio Decay Range", "Phasor Plot:Exponential Fading", "Phasor Plot:Phasor Ratio Reference Colors", "Phasor Plot:Reference Radius", "Phasor Plot:Show Color Map Vertices", "Phasor Plot:Phasor Plot Active", "Phasor Plot:Phasor Ratio Color Map Type", "Phasor Plot:Phasor Ratio Color Map", "Phasor Plot:Phasor Ratio Display Range", "Phasor Plot:Selected Image ROI(s)", "Phasor Plot:All Image ROIs", "Phasor Plot:Selected Phasor Plot ROI(s)", "Phasor Plot:All Phasor Plot ROIs", "Phasor Plot:Phasor Ratio Color-Coded Quantity", "Phasor Plot:Store Phasor Harmonics", "Phasor Plot:Draw Reference Segment", "Phasor Plot:User-Defined Quantity", "Phasor Graph:Phasor Frequency", "Phasor Graph:Phasor Ratio Type", "Phasor Graph:Pixel-level Phasor Computation", "Phasor Graph:Save Phasor Graph", "Phasor Graph:Phasor Graph Active", "Phasor Graph:Phasor SDV Options", "Phasor Calibration:Use Backup Calibration if needed", "Phasor Graph:Define Shortest Lifetime as", "Phasor Calibration:Backup Calibration Type", "Phasor Calibration:Calibration Type", "Phasor Calibration:Calibration Lifetime", "Phasor Calibration:Calibration Map Algorithm", "Single-Exponential Phasor Locus (SEPL):Gate Parameters", "Single-Exponential Phasor Locus (SEPL):User-defined Gate", "Single-Exponential Phasor Locus (SEPL):User-defined IRF", "Single-Exponential Phasor Locus (SEPL):Phasor Parameters", "Single-Exponential Phasor Locus (SEPL):Decay & IRF Parameters", "Single-Exponential Phasor Locus (SEPL):Display Parameters", "Lifetime Analysis:Decay Analysis Parameters", "Lifetime Analysis:Lifetime Map Active", "Plugins:Python Settings", "Miscellaneous:Verbose Mode", "Miscellaneous:Beep after Script", "Miscellaneous:Saved Image File Format", "Miscellaneous:Exported Gate Image Settings", "Miscellaneous:Include Loading in Timing", "Miscellaneous:Verbose Settings Mode", "Miscellaneous:Histogram Options", "Miscellaneous:Beep on Error", "Miscellaneous:# Logical Processors Used", "Miscellaneous:ROI Description Max Characters", "Miscellaneous:Verbose Error Mode", "Miscellaneous:Transparent Mask Color"}
  T29 = typedef "Palette.lvlib/Image Palette Information.ctl" = cluster{"Palette Name [# Colors,int?,inv?]":string, "Palette Type":T30, "Palette Colors":u32[], "Interpolate?":bool}
  T30 = typedef "Image.lvlib/Image Display Palette Type.ctl" = u32
  T31 = typedef "AlliGator Globals, Variables & Constants.lvlib/AlliGator Variables List.ctl" = enum16{"---- GUI ----", "GUI:Initialization Status", "GUI:State Indicators Refnum", "GUI:Original AlliGator Menu Items", "GUI:Current Action Loop State", "GUI:Script in progress", "GUI:Playback", "GUI:Loop Playback", "GUI:Search ROI Used", "GUI:Search ROI", "Decay Graph Max Legend Size", "Intensity Graph Max Legend Size", "Decay Statistics Graph Max Legend Size", "Phasor Graph Max Legend Size", "Phasor Ratio Graph Max Legend Size", "Lifetime Graph Max Legend Size", "---- Files ----", "Files:Export Dataset Frames as Individual Files", "Files:Show Batch Export Help Balloons", "Files:Frames in Dataset", "Files:ptu File Frame Start Indices", "Files:Current Frame in Dataset", "Files:Current Frame Timestamp", "Files:Dataset Loaded", "Files:Dataset Metadata", "Files:Dataset Channel", "Files:Dataset Data Description", "Files:Background Dataset Metadata", "Files:Background Dataset Channel", "Files:Background Dataset Data Description", "Files:Background File Subtraction", "Files:Background File Path", "Files:Background File Pile-up Correction", "Files:Background File Pixel Well Capacity", "Files:Background File Scaling Factor", "Files:Current Dataset Load Settings", "Files:Dataset Path", "Files:ICCD-specific Information", "Files:Macrotime Gate Separation", "------ Python Plugins ------", "Python Plugins:Information", "Python Plugins:Python Session", "Python Plugins:Valid Python Session?", "---- Source Image ----", "Source Image:ROIs", "Source Image:Current ROI", "Source Image:ROI Event Refnum", "X_Source Image Display Range", "X_Source Image Palette Information", "X_Type of Displayed Image", "X_Time Gate Slider", "Source Image:Palette List", "Source Image:Scale", "Source Image:ROI Overlay Color", "Source Image:Overlay to Erase", "Source Image:Is Displayed Image Accumulated", "Source Image:White Light Image Modified", "Source Image:Mask Image Modified", "---- Image Profile Window ----", "Image Profile:Window Event Refnum", "Image Profile:IntensityType", "Image Profile:Intensity Average Type", "Image Profile:Intensity-weighted SDV", "Image Profile:Box Profile Type", "Image Profile:Window Open", "Image Profile:Plotted Fit Parameter", "------ Phasor Graph -------", "Phasor Graph:Show Line", "---- Phasor Plot ---", "Phasor Plot:Parameters Changed", "Phasor Plot:FLI Dataset Modified since last Calculation", "Phasor Harmonics Data", "Selected Phasor Harmonics", "Phasor Harmonic Manager Event Refnum", "Phasor Plot:ROIs", "Phasor Plot:Current ROI", "Phasor Plot:ROI Event Refnum", "Phasor Plot:Image Reference Points", "Phasor Plot:Computed", "Phasor Plot:Palette Information", "Phasor Plot:Palette List", "Phasor Plot:Phasor Ratio Palette Information", "Phasor Plot:Phasor Ratio Palette List", "Phasor Plot:Image Scale", "Phasor Plot:Image Overlay to Erase", "Phasor Plot:Image Elements to Update", "Phasor Plot:Current Calculation Parameters", "Phasor Plot:Current Calibration Options", "Phasor Plot:Reset Cumulated Phasor Plot", "Phasor Plot:Reference 1", "Phasor Plot:Lifetime Reference 1", "Phasor Plot:Reference 1 Frequency", "Phasor Plot:Reference 2", "Phasor Plot:Lifetime Reference 2", "Phasor Plot:Reference 2 Frequency", "---- Decay Analysis ----", "Number of Selected Decays to Fit", "LS Fit Results", "LAR Fit Results", "BS Fit Results", "Last Decay Max - Min", "Best Fit Parameters", "Best Fit Parameter Names", "Actual Size X", "Actual Size Y", "Binning X", "Binning Y", "Actual # Gates", "Dataset Number", "Gates to...", "Gates Skipped", "Gates to keep", "Gate Step", "Gate Separation", "Reversed Gates", "Pile-up Correction", "Pixel Well Capacity", "Background Subtracted", "Background Subtraction Method", "Background Definition Range", "Background File (deprecated)", "Number of Dataset Accumulated", "Array of Accumulated Dataset Paths", "Do Averaged Datasets", "Destination File Path", "Process Plot Target", "Use 1/D as Phasor Frequency", "---- Decay Fit Parameter Map -----", "Decay Fit Parameter Map:Palette Information", "Decay Fit Parameter Map:Palette List", "------- Local Decay Window ---------", "Local Decay Graph Window:Event Refnum", "Local Decay Graph Window:Use normalized IRF for convolution", "----- Miscellaneous ----", "Misc:Skippable Dialog Windows Status"}
  T32 = enum16{"0", "1", "2", "3", "4", "5", "6", "7", "8", "9", "A", "B", "C", "D", "E", "F", "G", "H", "I", "J", "K", "L", "M", "N", "O", "P", "Q", "R", "S", "T", "U", "V", "W", "X", "Y", "Z", "F1", "F2", "F3", "F4", "F5", "F6", "F7", "F8", "F9", "F10", "F11", "F12", "F13", "F14", "F15", "ADD", "BACK", "BACKSLASH", "CAPITAL", "COMMA", "DECIMAL", "DELETE", "DIVIDE", "DOWN", "END", "EQUALS", "ESCAPE", "GRAVE (`)", "HOME", "INSERT", "LBRACKET", "LCONTROL", "LEFT", "L ALT", "LSHIFT", "LWIN", "MINUS", "MULTIPLY", "NEXT", "NUMLOCK", "NUMPAD_0", "NUMPAD_1", "NUMPAD_2", "NUMPAD_3", "NUMPAD_4", "NUMPAD_5", "NUMPAD_6", "NUMPAD_7", "NUMPAD_8", "NUMPAD_9", "PAUSE", "PERIOD", "PRIOR (PG UP)", "RBRACKET", "RCONTROL", "RETURN", "RIGHT", "R ALT", "RSHIFT", "RWIN", "SCROLL", "SEMICOLON", "SLASH", "SPACE", "SUBTRACT", "TAB", "UP", "ENTER (num pad)", "' (quote)"}
  T33 = typedef "Image.lvlib/Image Display Event.ctl" = cluster{"Item Tag":string, "Image Control Refnum":T34, "Coords":T35, "Item Path":string}
  T34 = typedef "Image.lvlib/Image Control Refnum.ctl" = refnum<vi>
  T35 = typedef "LVPoint32TypeDef.ctl" = cluster{"Horizontal":i32, "Vertical":i32}
  T36 = typedef "AlliGator Decay Fit Parameter Map.lvlib/AlliGator Decay Parameter Map Update Event Data.ctl" = cluster{"Parameter":T11, "Parameter changed":bool}
  T37 = typedef "XY Graph Add-Ons.lvlib/XY Graph Event.ctl" = cluster{"Item Tag":string, "XY Graph Refnum":refnum<vi>, "Coords":T35, "Item Path":string}
  T38 = typedef "Utilities.lvlib/Read-Write.ctl" = enum16{"Read", "Write"}
  T39 = typedef "AlliGator Action Engine.lvlib/AlliGator Filtered Event Data.ctl" = cluster{"AlliGator Q Event":T24, "Time":u32, "Timeout":u32}
  T40 = typedef "XY Graph Add-Ons.lvlib/XY Graph Mouse Click Event Data.ctl" = cluster{"Multiplot XY Graph":T41, "Mouse Coordinates":T35}
  T41 = typedef "XY Graph Add-Ons.lvlib/XY Graph Refnum.ctl" = refnum<vi>
  T42 = typedef "AlliGator ROIs.lvlib/AlliGator ROI Manager Actions.ctl" = enum16{"Undefined", "Delete Current ROI", "Delete All Unselected ROIs", "Delete Multiple ROIs", "Delete All ROIs", "Swap ROIs", "Insert ROI", "Update Current ROI Descriptor", "Rename Current ROI", "Store New ROI", "Store Multiple ROIs", "Select Next ROI", "Select Previous ROI", "Find Selected ROI", "Show All ROIs", "Update ROI Manager Window", "Merge All ROIs", "Unmerge ROI", "Set Selected ROI by ID"}
  T43 = typedef "Image.lvlib/Image Display User Event Data.ctl" = cluster{"Image Control Refnum":T34, "Coords":T35, "button info":cluster{"button 1":bool, "button 2":bool, "button 3":bool, "button 4":bool}, "keys pressed":enum16{"0", "1", "2", "3", "4", "5", "6", "7", "8", "9", "A", "B", "C", "D", "E", "F", "G", "H", "I", "J", "K", "L", "M", "N", "O", "P", "Q", "R", "S", "T", "U", "V", "W", "X", "Y", "Z", "F1", "F2", "F3", "F4", "F5", "F6", "F7", "F8", "F9", "F10", "F11", "F12", "F13", "F14", "F15", "ADD", "BACK", "BACKSLASH", "CAPITAL", "COMMA", "DECIMAL", "DELETE", "DIVIDE", "DOWN", "END", "EQUALS", "ESCAPE", "GRAVE (`)", "HOME", "INSERT", "LBRACKET", "LCONTROL", "LEFT", "L ALT", "LSHIFT", "LWIN", "MINUS", "MULTIPLY", "NEXT", "NUMLOCK", "NUMPAD_0", "NUMPAD_1", "NUMPAD_2", "NUMPAD_3", "NUMPAD_4", "NUMPAD_5", "NUMPAD_6", "NUMPAD_7", "NUMPAD_8", "NUMPAD_9", "PAUSE", "PERIOD", "PRIOR (PG UP)", "RBRACKET", "RCONTROL", "RETURN", "RIGHT", "R ALT", "RSHIFT", "RWIN", "SCROLL", "SEMICOLON", "SLASH", "SPACE", "SUBTRACT", "TAB", "UP", "ENTER (num pad)", "' (quote)"}[]}
  T44 = typedef "AlliGator Phasor Plot.lvlib/AlliGator Phasor Plot Mouse Up Event Data.ctl" = cluster{"Current ROI Tool":u32, "ROI Descriptor":T45, "Shift":bool, "Alt":bool}
  T45 = typedef "Image.lvlib/Image ROI Descriptor.ctl" = cluster{"Global Rectangle":i32[], "Contours":T46[]}
  T46 = typedef "Image.lvlib/Image Contour Definition.ctl" = cluster{"Contour Type":T47, "ROI Type":T48, "Points":i32[]}
  T47 = typedef "Image.lvlib/Image Contour ID.ctl" = enum32{"External", "Internal"}
  T48 = typedef "Image.lvlib/Image ROI Type.ctl" = enum16{"No Selection", "Point", "Line", "Rectangle", "Oval", "Polygon", "Freehand Region", "Annulus", "Unused2", "Unused3", "Broken Line", "Freehand Line", "Rotated Rectangle"}
  T49 = enum16{"0", "1", "2", "3", "4", "5", "6", "7", "8", "9", "A", "B", "C", "D", "E", "F", "G", "H", "I", "J", "K", "L", "M", "N", "O", "P", "Q", "R", "S", "T", "U", "V", "W", "X", "Y", "Z", "F1", "F2", "F3", "F4", "F5", "F6", "F7", "F8", "F9", "F10", "F11", "F12", "F13", "F14", "F15", "ADD", "BACK", "BACKSLASH", "CAPITAL", "COMMA", "DECIMAL", "DELETE", "DIVIDE", "DOWN", "END", "EQUALS", "ESCAPE", "GRAVE (`)", "HOME", "INSERT", "LBRACKET", "LCONTROL", "LEFT", "L ALT", "LSHIFT", "LWIN", "MINUS", "MULTIPLY", "NEXT", "NUMLOCK", "NUMPAD_0", "NUMPAD_1", "NUMPAD_2", "NUMPAD_3", "NUMPAD_4", "NUMPAD_5", "NUMPAD_6", "NUMPAD_7", "NUMPAD_8", "NUMPAD_9", "PAUSE", "PERIOD", "PRIOR (PG UP)", "RBRACKET", "RCONTROL", "RETURN", "RIGHT", "R ALT", "RSHIFT", "RWIN", "SCROLL", "SEMICOLON", "SLASH", "SPACE", "SUBTRACT", "TAB", "UP", "ENTER (num pad)", "' (quote)"}[]
  T50 = typedef "XY Graph Add-Ons.lvlib/New Plot Information.ctl" = cluster{"Multiplot XY Graph":refnum<vi>, "Plot Name":string, "Plot Scales":T51, "Plot Interpolation":T52, "Point Style":T53, "Plot Color":u32, "Plot Metadata":variant}
  T51 = typedef "XY Graph Add-Ons.lvlib/Plot Scales.ctl" = cluster{"X Scale":u32, "Y Scale":u32}
  T52 = typedef "Graphs.lvlib/LabVIEW Plot Interpolation.ctl" = u8
  T53 = typedef "Graphs.lvlib/Plot Point Style.ctl" = enum16{"not defined", "None", "Empty Circle", "Filled Circle", "Thick Circle", "Dotted Circle", "Empty Square", "Filled Square", "Thick Square", "Dotted Square", "Small Filled Square", "Dot", "Cross", "Tiny Cross", "Large X", "Small x", "Diamond", "Small Empty Square"}
  T54 = typedef "AlliGator Settings.lvlib/AlliGator Settings Window Messages.ctl" = enum16{"Idle", "Subscribe", "Unsubscribe", "Refresh Parameter", "Refresh All Parameters", "Quit"}
  T55 = typedef "AlliGator Phasor Plot Color Map.lvlib/AlliGator Phasor Color Map User Event List.ctl" = enum16{"Init", "Vertex Update", "Color Change"}
  T56 = cluster{"button 1":bool, "button 2":bool, "button 3":bool, "button 4":bool}
  T57 = cluster{"Global Rectangle":i32[], "Contours":cluster{"Contour Type":u32, "ROI Type":u32, "Points":i32[]}[]}
  T58 = typedef "Rich Text Box.lvlib/Text Formatting.ctl" = cluster{"Font":string, "Text Color":T59, "Text Background Color":T59, "Text Style":enum16{"Regular", "Bold", "Italic", "Underline", "Strikeout"}, "Font Size (Points)":dbl, "Text Alignment":i32}
  T59 = typedef "Rich Text Box.lvlib/Text Colors.ctl" = enum16{"Unchanged", "Black", "Blue", "Brown", "Gray", "Green", "Orange", "Pink", "Red", "White"}
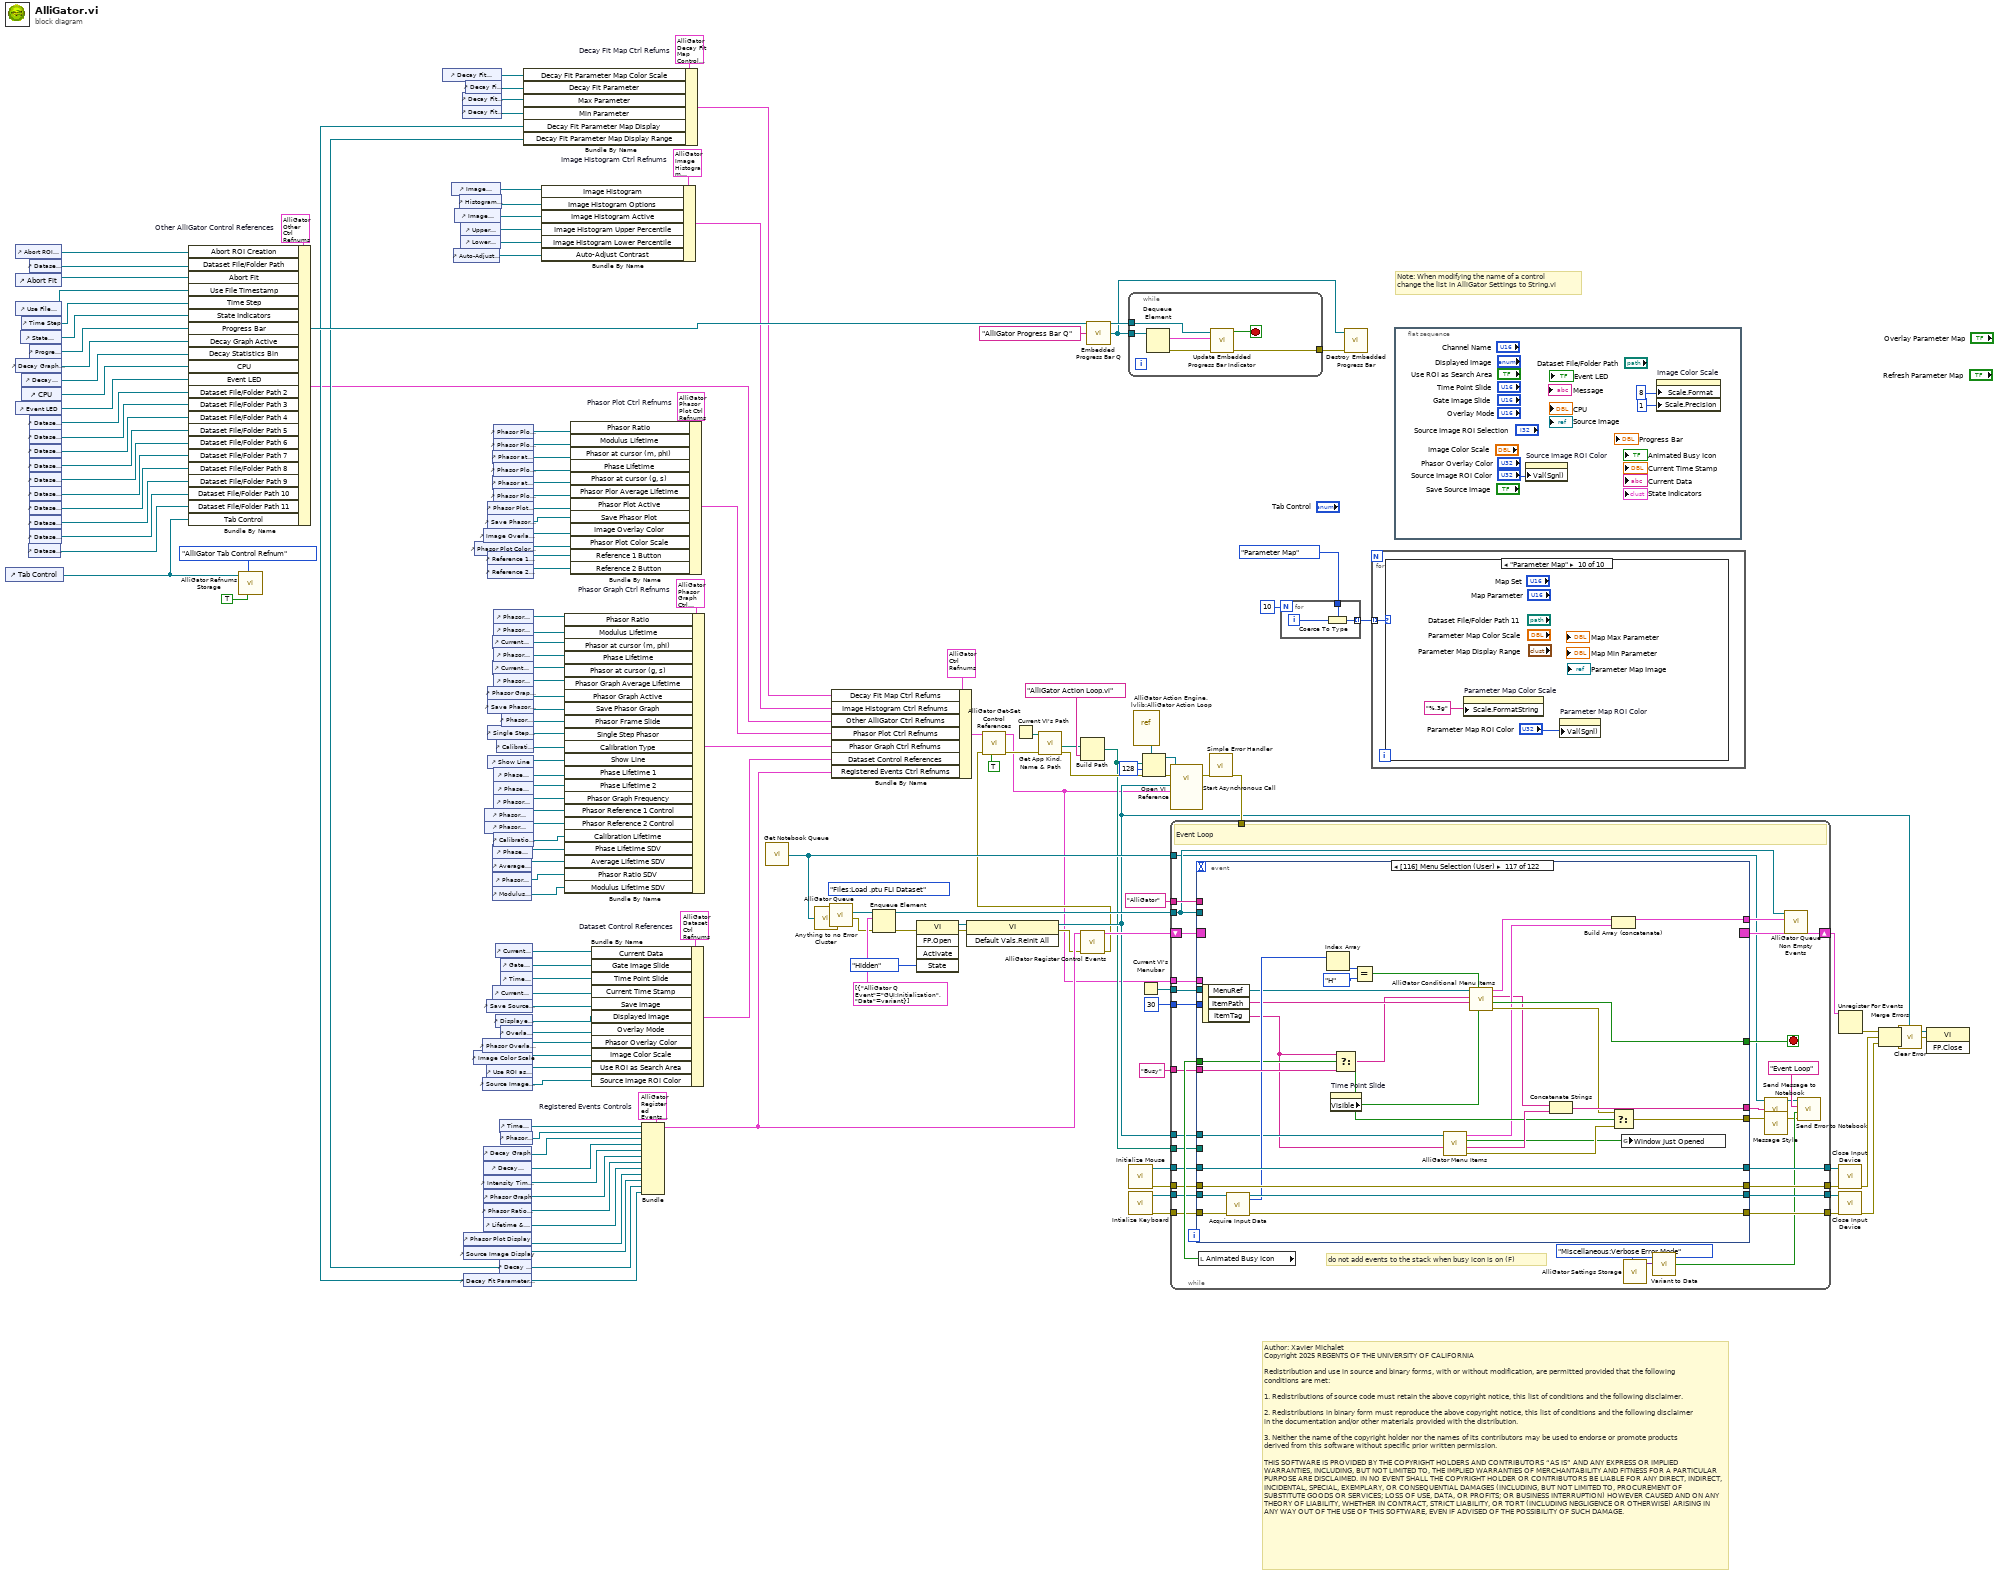
[diagram p0: block diagram]
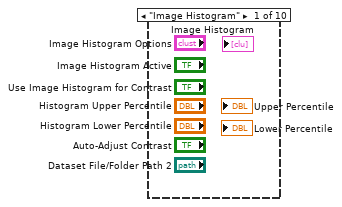
[diagram p2: hidden frame]
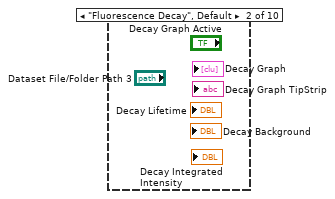
[diagram p3: hidden frame]
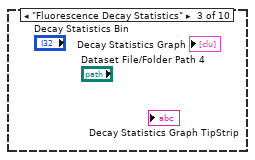
[diagram p4: hidden frame]
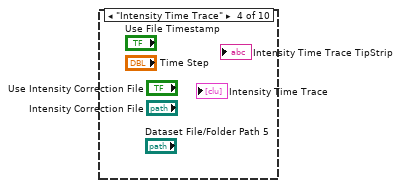
[diagram p5: hidden frame]
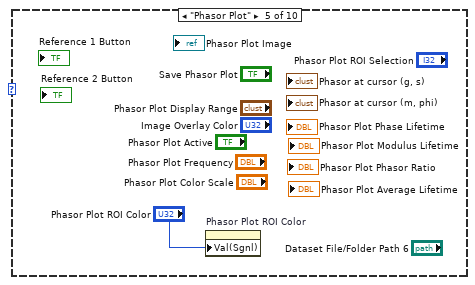
[diagram p6: hidden frame]
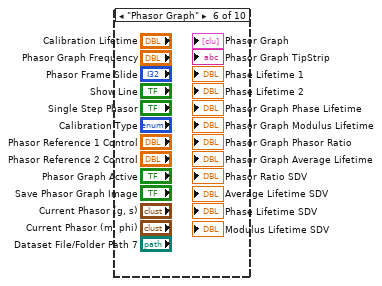
[diagram p7: hidden frame]
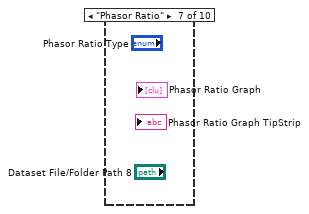
[diagram p8: hidden frame]
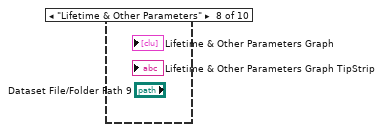
[diagram p9: hidden frame]
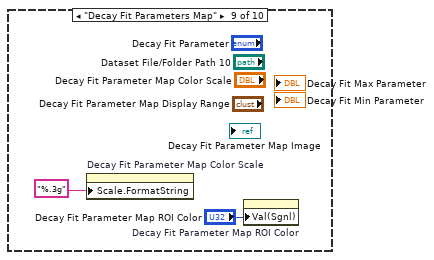
[diagram p10: hidden frame]
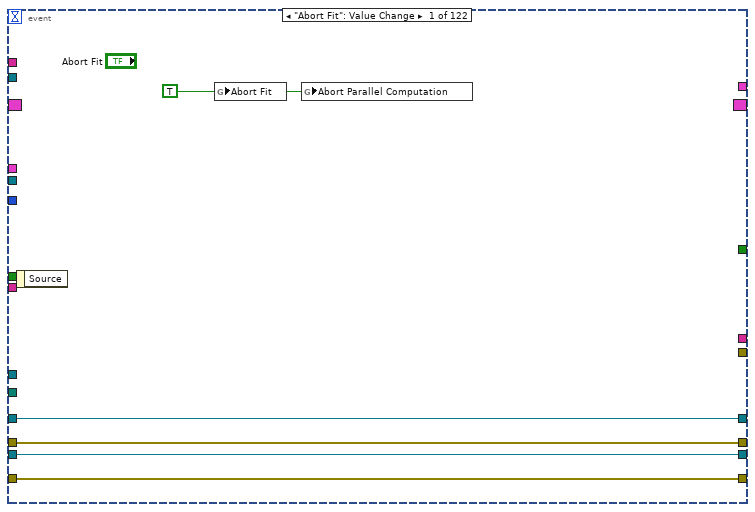
[diagram p11: hidden frame]
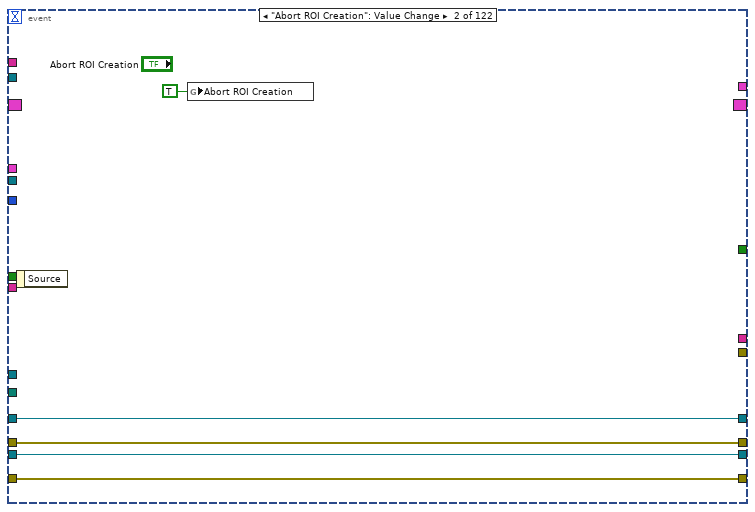
[diagram p12: hidden frame]
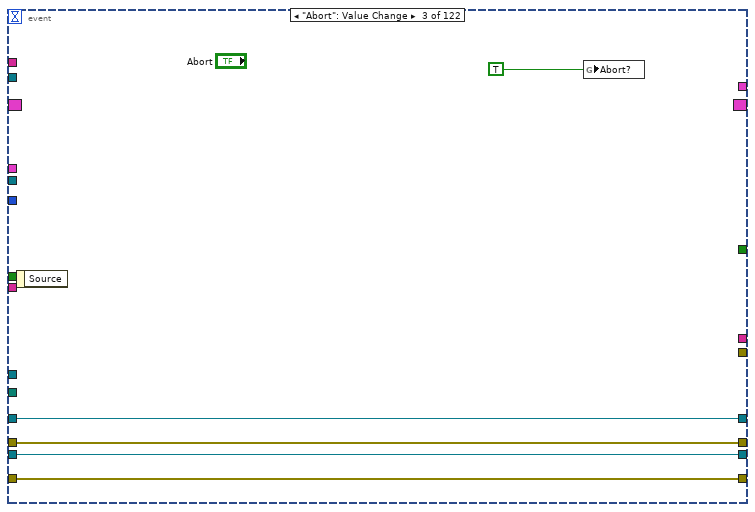
[diagram p13: hidden frame]
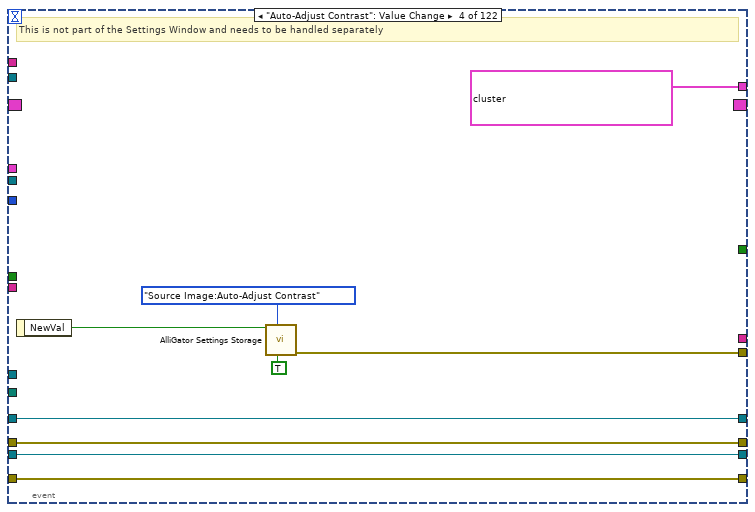
[diagram p14: hidden frame]
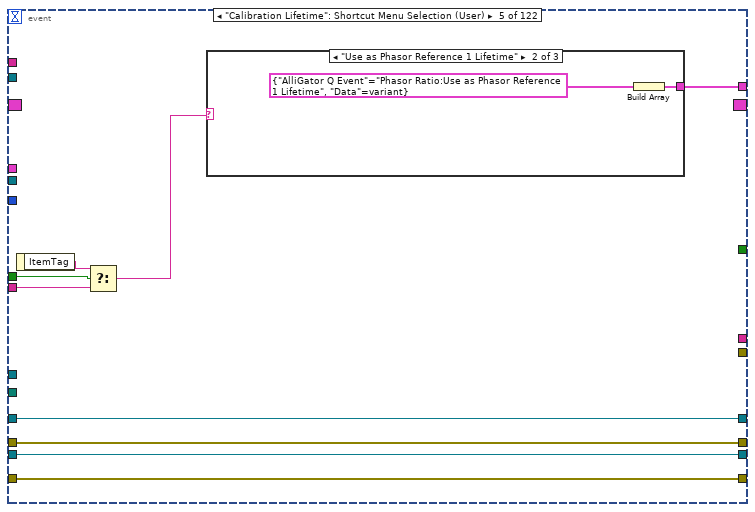
[diagram p15: hidden frame]
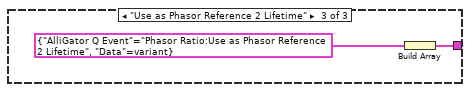
[diagram p17: hidden frame]
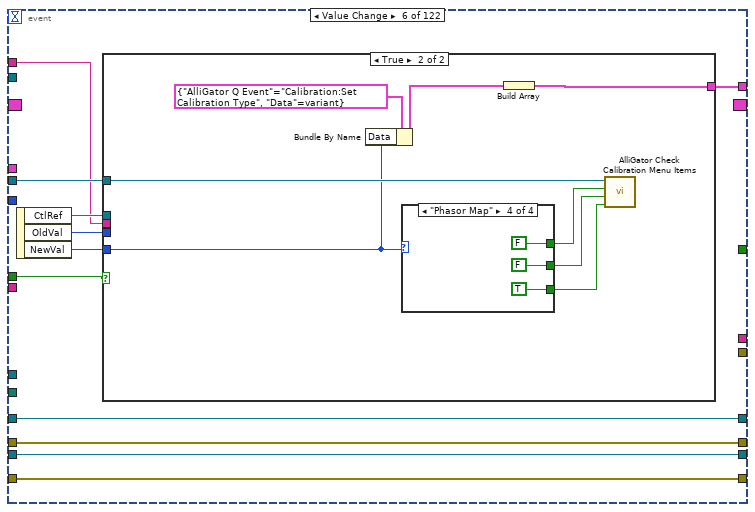
[diagram p18: hidden frame]
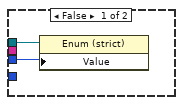
[diagram p19: hidden frame]
diagram:
  w70 = T15 {"Decay Fit Parameter Map Color Scale"=refnum, "Decay Fit Parameter"=refnum, "Max Parameter"=refnum, "Min Parameter"=refnum, "Decay Fit Parameter Map Display"=refnum, "Decay Fit Parameter Map Display Range"=refnum}  # Decay Fit Map Ctrl Refums
  w74 = T16 {"Image Histogram"=refnum, "Image Histogram Options"=refnum, "Image Histogram Active"=refnum, "Image Histogram Upper Percentile"=refnum, "Image Histogram Lower Percentile"=refnum, "Auto-Adjust Contrast"=refnum}  # Image Histogram Ctrl Refnums
  w93 = T17 {"Phasor Ratio"=refnum, "Modulus Lifetime"=refnum, "Phasor at cursor (m, phi)"=refnum, "Phase Lifetime"=refnum, "Phasor at cursor (g, s)"=refnum, "Phasor Graph Average Lifetime"=refnum, "Phasor Graph Active"=refnum, "Save Phasor Graph"=refnum, "Phasor Frame Slide"=refnum, "Single Step Phasor"=refnum, "Calibration Type"=refnum, "Show Line"=refnum, "Phase Lifetime 1"=refnum, "Phase Lifetime 2"=refnum, "Phasor Graph Frequency"=refnum, "Phasor Reference 1 Control"=refnum, "Phasor Reference 2 Control"=refnum, "Calibration Lifetime"=refnum, "Phase Lifetime SDV"=refnum, "Average Lifetime SDV"=refnum, "Phasor Ratio SDV"=refnum, "Modulus Lifetime SDV"=refnum}  # Phasor Graph Ctrl Refnums
  w94 = T18 {"Phasor Ratio"=refnum, "Modulus Lifetime"=refnum, "Phasor at cursor (m, phi)"=refnum, "Phase Lifetime"=refnum, "Phasor at cursor (g, s)"=refnum, "Phasor Plor Average Lifetime"=refnum, "Phasor Plot Active"=refnum, "Save Phasor Plot"=refnum, "Image Overlay Color"=refnum, "Phasor Plot Color Scale"=refnum, "Reference 1 Button"=refnum, "Reference 2 Button"=refnum}  # Phasor Plot Ctrl Refnums
  (unwired) AlliGator_Q_Event."Files:Load .ptu FLI Dataset" ("AlliGator Q Event")
  w139 = T23 {"Time Point Slider"=refnum, "Phasor Plot Display Range"=refnum, "Decay Graph"=refnum, "Decay Statistics Graph"=refnum, "Intensity Time Trace"=refnum, "Phasor Graph"=refnum, "Phasor Ratio Graph"=refnum, "Lifetime Graph"=refnum, "Phasor Plot Display"=refnum, "Source Image Display"=refnum, "Decay Fit Parameter Map Display Range"=refnum, "Decay Fit Parameter Map Display"=refnum}  # Registered Events Controls
  w120 = T21 {"State Indicators"=refnum, " Progress Bar"=refnum, "Decay Graph Active"=refnum, "Decay Statistics Bin"=refnum, "Time Step"=refnum, "Use File Timestamp"=refnum, "Tab Control"=refnum, "CPU"=refnum, "Abort Fit"=refnum, "Dataset File/Folder Path"=refnum, "Abort ROI Creation"=refnum, "Event LED"=refnum, "Dataset File/Folder Path 2"=refnum, "Dataset File/Folder Path 3"=refnum, "Dataset File/Folder Path 4"=refnum, "Dataset File/Folder Path 5"=refnum, "Dataset File/Folder Path 6"=refnum, "Dataset File/Folder Path 7"=refnum, "Dataset File/Folder Path 8"=refnum, "Dataset File/Folder Path 9"=refnum, "Dataset File/Folder Path 10"=refnum, "Dataset File/Folder Path 11"=refnum}  # Other AlliGator Control References
  w147 = T22 {"Current Data"=refnum, "Gate Image Slide"=refnum, "Time Point Slide"=refnum, "Current Time Stamp"=refnum, "Save Image"=refnum, "Displayed Image"=refnum, "Overlay Mode"=refnum, "Phasor Overlay Color"=refnum, "Image Color Scale"=refnum, "Use ROI as Search Area"=refnum, "Source Image ROI Color"=refnum}  # Dataset Control References
  # "Author: Xavier Michalet\nCopyright 2025 REGENTS OF THE UNIVERSITY OF CALIFORNIA\n\nRedistribution and use in source and binary forms, with or without modification, are permitted provided that the following conditions are met:\n\n1. Redistributions of source code must retain the above copyright notice, this list of conditions and the following disclaimer.\n\n2. Redistributions in binary form must reproduce the above copyright notice, this list of conditions and the following disclaimer in the documentation and/or other materials provided with the distribution.\n\n3. Neither the name of the copyright holder nor the names of its contributors may be used to endorse or promote products derived from this software without specific prior written permission.\n\nTHIS SOFTWARE IS PROVIDED BY THE COPYRIGHT HOLDERS AND CONTRIBUTORS “AS IS” AND ANY EXPRESS OR IMPLIED WARRANTIES, INCLUDING, BUT NOT LIMITED TO, THE IMPLIED WARRANTIES OF MERCHANTABILITY AND FITNESS FOR A PARTICULAR PURPOSE ARE DISCLAIMED. IN NO EVENT SHALL THE COPYRIGHT HOLDER OR CONTRIBUTORS BE LIABLE FOR ANY DIRECT, INDIRECT, INCIDENTAL, SPECIAL, EXEMPLARY, OR CONSEQUENTIAL DAMAGES (INCLUDING, BUT NOT LIMITED TO, PROCUREMENT OF SUBSTITUTE GOODS OR SERVICES; LOSS OF USE, DATA, OR PROFITS; OR BUSINESS INTERRUPTION) HOWEVER CAUSED AND ON ANY THEORY OF LIABILITY, WHETHER IN CONTRACT, STRICT LIABILITY, OR TORT (INCLUDING NEGLIGENCE OR OTHERWISE) ARISING IN ANY WAY OUT OF THE USE OF THIS SOFTWARE, EVEN IF ADVISED OF THE POSSIBILITY OF SUCH DAMAGE."
  # "Note: When modifying the name of a control\nchange the list in AlliGator Settings to String.vi"
  n1 = control-ref of="Tab Control"() -> (w1:refnum<vi>)
  n2 = control-ref of="Abort ROI Creation"() -> (w79:refnum<vi>)
  n3 = control-ref of="Abort Fit"() -> (w82:refnum<vi>)
  n4 = control-ref of="Use File Timestamp"() -> (w95:refnum<vi>)
  n5 = control-ref of="Decay Graph Active"() -> (w103:refnum<vi>)
  n6 = control-ref of="Event LED"() -> (w36:refnum<vi>)
  n7 = control-ref of="State Indicators"() -> (w122:refnum<vi>)
  n8 = control-ref of="Time Step"() -> (w96:refnum<vi>)
  n9 = control-ref of="Decay Statistics Bin"() -> (w98:refnum<vi>)
  n10 = control-ref of="CPU"() -> (w83:refnum<vi>)
  n11 = control-ref of="Dataset File/Folder Path 11"() -> (w2:refnum<vi>)
  n12 = control-ref of="Dataset File/Folder Path"() -> (w81:refnum<vi>)
  n13 = control-ref of="Progress Bar"() -> (w119:refnum<vi>)
  n14 = control-ref of="Dataset File/Folder Path 2"() -> (w14:refnum<vi>)
  n15 = control-ref of="Dataset File/Folder Path 3"() -> (w13:refnum<vi>)
  n16 = control-ref of="Dataset File/Folder Path 4"() -> (w12:refnum<vi>)
  n17 = control-ref of="Dataset File/Folder Path 5"() -> (w11:refnum<vi>)
  n18 = control-ref of="Dataset File/Folder Path 6"() -> (w10:refnum<vi>)
  n19 = control-ref of="Dataset File/Folder Path 7"() -> (w9:refnum<vi>)
  n20 = control-ref of="Dataset File/Folder Path 8"() -> (w8:refnum<vi>)
  n21 = control-ref of="Dataset File/Folder Path 9"() -> (w7:refnum<vi>)
  n22 = control-ref of="Dataset File/Folder Path 10"() -> (w6:refnum<vi>)
  n23 = Bundle By Name(cluster=w120, "Abort ROI Creation"=w79, "Dataset File/Folder Path"=w81, "Abort Fit"=w82, "Use File Timestamp"=w95, "Time Step"=w96, "State Indicators"=w122, "Progress Bar"=w119, "Decay Graph Active"=w103, "Decay Statistics Bin"=w98, "CPU"=w83, "Event LED"=w36, "Dataset File/Folder Path 2"=w14, "Dataset File/Folder Path 3"=w13, "Dataset File/Folder Path 4"=w12, "Dataset File/Folder Path 5"=w11, "Dataset File/Folder Path 6"=w10, "Dataset File/Folder Path 7"=w9, "Dataset File/Folder Path 8"=w8, "Dataset File/Folder Path 9"=w7, "Dataset File/Folder Path 10"=w6, "Dataset File/Folder Path 11"=w2, "Tab Control"=w1) -> (w5:T21)
  n24 = call "AlliGator Refnums Storage.vi"("Get(F)/Set"=TRUE, "AlliGator Refnum List"=AlliGator_Refnums_List."AlliGator Tab Control Refnum", "Data in"=w1) -> ()  [unwired: 7 in, 2 out]
  n25 = control-ref of="Decay Fit Parameter Map Color Scale"() -> (w69:refnum<vi>)
  n26 = control-ref of="Image Histogram"() -> (w78:refnum<vi>)
  n27 = control-ref of="Auto-Adjust Contrast"() -> (w31:refnum<vi>)
  n28 = control-ref of="Image Histogram Active"() -> (w77:refnum<vi>)
  n29 = control-ref of="Histogram Options"() -> (w26:refnum<vi>)
  n30 = control-ref of="Upper Percentile"() -> (w76:refnum<vi>)
  n31 = control-ref of="Lower Percentile"() -> (w75:refnum<vi>)
  n32 = control-ref of="Decay Fit Max Parameter"() -> (w64:refnum<vi>)
  n33 = control-ref of="Decay Fit Min Parameter"() -> (w65:refnum<vi>)
  n34 = control-ref of="Phasor Plot Display"() -> (w152:refnum<vi>)
  n35 = control-ref of="Source Image Display"() -> (w151:refnum<vi>)
  n36 = control-ref of="Decay Fit Parameter Map Display"() -> (w67:refnum<vi>)
  n37 = control-ref of="Decay Fit Parameter"() -> (w68:refnum<vi>)
  n38 = control-ref of="Image Color Scale"() -> (w85:refnum<vi>)
  n39 = control-ref of="Phasor Plot Color Scale"() -> (w86:refnum<vi>)
  n40 = control-ref of="Phasor Overlay Color"() -> (w99:refnum<vi>)
  n41 = control-ref of="Source Image ROI Color"() -> (w32:refnum<vi>)
  n42 = control-ref of="Image Overlay Color"() -> (w97:refnum<vi>)
  n43 = control-ref of="Decay Graph"() -> (w144:refnum<vi>)
  n44 = control-ref of="Decay Statistics Graph"() -> (w143:refnum<vi>)
  n45 = control-ref of="Intensity Time Trace"() -> (w142:refnum<vi>)
  n46 = control-ref of="Phasor Graph"() -> (w52:refnum<vi>)
  n47 = control-ref of="Phasor Ratio Graph"() -> (w141:refnum<vi>)
  n48 = control-ref of="Lifetime & Other Parameters Graph"() -> (w140:refnum<vi>)
  n49 = control-ref of="Phasor Reference 1 Control"() -> (w84:refnum<vi>)
  n50 = control-ref of="Phasor Reference 2 Control"() -> (w72:refnum<vi>)
  n51 = control-ref of="Save Source Image"() -> (w108:refnum<vi>)
  n52 = control-ref of="Use ROI as Search Area"() -> (w80:refnum<vi>)
  n53 = control-ref of="Phasor Plot Active"() -> (w111:refnum<vi>)
  n54 = control-ref of="Save Phasor Plot"() -> (w56:refnum<vi>)
  n55 = control-ref of="Reference 1 Button"() -> (w21:refnum<vi>)
  n56 = control-ref of="Reference 2 Button"() -> (w20:refnum<vi>)
  n57 = control-ref of="Phasor Graph Active"() -> (w110:refnum<vi>)
  n58 = control-ref of="Save Phasor Graph Image"() -> (w109:refnum<vi>)
  n59 = control-ref of="Single Step Phasor"() -> (w91:refnum<vi>)
  n60 = control-ref of="Show Line"() -> (w90:refnum<vi>)
  n61 = control-ref of="Phasor at cursor (m, phi)"() -> (w130:refnum<vi>)
  n62 = control-ref of="Phasor at cursor (g, s)"() -> (w128:refnum<vi>)
  n63 = control-ref of="Current Phasor (m, phi)"() -> (w125:refnum<vi>)
  n64 = control-ref of="Current Phasor (g, s)"() -> (w123:refnum<vi>)
  n65 = control-ref of="Average Lifetime SDV"() -> (w24:refnum<vi>)
  n66 = control-ref of="Phasor Ratio SDV"() -> (w23:refnum<vi>)
  n67 = control-ref of="Modulus Lifetime SDV"() -> (w22:refnum<vi>)
  n68 = control-ref of="Phase Lifetime SDV"() -> (w25:refnum<vi>)
  n69 = control-ref of="Current Time Stamp"() -> (w133:refnum<vi>)
  n70 = control-ref of="Phasor Plot Phasor Ratio"() -> (w132:refnum<vi>)
  n71 = control-ref of="Phasor Plot Modulus Lifetime"() -> (w131:refnum<vi>)
  n72 = control-ref of="Phasor Plot Phase Lifetime"() -> (w129:refnum<vi>)
  n73 = control-ref of="Phasor Plot Average Lifetime"() -> (w112:refnum<vi>)
  n74 = control-ref of="Phasor Graph Phasor Ratio"() -> (w127:refnum<vi>)
  n75 = control-ref of="Phasor Graph Modulus Lifetime"() -> (w126:refnum<vi>)
  n76 = control-ref of="Phasor Graph Phase Lifetime"() -> (w124:refnum<vi>)
  n77 = control-ref of="Phasor Graph Average Lifetime"() -> (w113:refnum<vi>)
  n78 = control-ref of="Phase Lifetime 1"() -> (w89:refnum<vi>)
  n79 = control-ref of="Phase Lifetime 2"() -> (w88:refnum<vi>)
  n80 = control-ref of="Phasor Graph Frequency"() -> (w87:refnum<vi>)
  n81 = control-ref of="Calibration Lifetime"() -> (w71:refnum<vi>)
  n82 = control-ref of="Current Data"() -> (w149:refnum<vi>)
  n83 = control-ref of="Displayed Image"() -> (w107:refnum<vi>)
  n84 = control-ref of="Calibration Type"() -> (w38:refnum<vi>)
  n85 = control-ref of="Time Point Slide"() -> (w146:refnum<vi>)
  n86 = control-ref of="Decay Fit Parameter Map Display Range"() -> (w63:refnum<vi>)
  n87 = control-ref of="Gate Image Slide"() -> (w148:refnum<vi>)
  n88 = control-ref of="Time Point Slide"() -> (w134:refnum<vi>)
  n89 = control-ref of="Overlay Mode"() -> (w100:refnum<vi>)
  n90 = control-ref of="Phasor Plot Display Range"() -> (w145:refnum<vi>)
  n91 = control-ref of="Phasor Frame Slide"() -> (w92:refnum<vi>)
  n92 = Bundle By Name(cluster=w70, "Decay Fit Parameter Map Color Scale"=w69, "Decay Fit Parameter"=w68, "Max Parameter"=w64, "Min Parameter"=w65, "Decay Fit Parameter Map Display"=w67, "Decay Fit Parameter Map Display Range"=w63) -> (w66:T15)
  n93 = Bundle By Name(cluster=w74, "Image Histogram"=w78, "Image Histogram Options"=w26, "Image Histogram Active"=w77, "Image Histogram Upper Percentile"=w76, "Image Histogram Lower Percentile"=w75, "Auto-Adjust Contrast"=w31) -> (w73:T16)
  n94 = Bundle By Name(cluster=w93, "Phasor Ratio"=w127, "Modulus Lifetime"=w126, "Phasor at cursor (m, phi)"=w125, "Phase Lifetime"=w124, "Phasor at cursor (g, s)"=w123, "Phasor Graph Average Lifetime"=w113, "Phasor Graph Active"=w110, "Save Phasor Graph"=w109, "Phasor Frame Slide"=w92, "Single Step Phasor"=w91, "Calibration Type"=w38, "Show Line"=w90, "Phase Lifetime 1"=w89, "Phase Lifetime 2"=w88, "Phasor Graph Frequency"=w87, "Phasor Reference 1 Control"=w84, "Phasor Reference 2 Control"=w72, "Calibration Lifetime"=w71, "Phase Lifetime SDV"=w25, "Average Lifetime SDV"=w24, "Phasor Ratio SDV"=w23, "Modulus Lifetime SDV"=w22) -> (w39:T17)
  n95 = Bundle By Name(cluster=w94, "Phasor Ratio"=w132, "Modulus Lifetime"=w131, "Phasor at cursor (m, phi)"=w130, "Phase Lifetime"=w129, "Phasor at cursor (g, s)"=w128, "Phasor Plor Average Lifetime"=w112, "Phasor Plot Active"=w111, "Save Phasor Plot"=w56, "Image Overlay Color"=w97, "Phasor Plot Color Scale"=w86, "Reference 1 Button"=w21, "Reference 2 Button"=w20) -> (w106:T18)
  n96 = Bundle By Name(cluster=w147, "Current Data"=w149, "Gate Image Slide"=w148, "Time Point Slide"=w134, "Current Time Stamp"=w133, "Save Image"=w108, "Displayed Image"=w107, "Overlay Mode"=w100, "Phasor Overlay Color"=w99, "Image Color Scale"=w85, "Use ROI as Search Area"=w80, "Source Image ROI Color"=w32) -> (w105:T22)
  n97 = Bundle(cluster=w139, "Time Point Slider"=w146, "Phasor Plot Display Range"=w145, "Decay Graph"=w144, "Decay Statistics Graph"=w143, "Intensity Time Trace"=w142, "Phasor Graph"=w52, "Phasor Ratio Graph"=w141, "Lifetime Graph"=w140, "Phasor Plot Display"=w152, "Source Image Display"=w151, "Decay Fit Parameter Map Display Range"=w63, "Decay Fit Parameter Map Display"=w67) -> (w35:T23)
  n98 = call "Get Notebook Queue.vi"() -> ("Notebook Queue"=w59:refnum<queue>)  [unwired: 9 in]
  n99 = call "Anything to no Error Cluster.vi"("Variant"=w59) -> ("Error Out"=w58:errorcluster)  [unwired: 8 in]
  n100 = call "AlliGator Queue.vi"("Error In"=w58) -> ("Error Out"=w150:errorcluster, "AlliGator Q"=w158:refnum<queue>)  [unwired: 7 in]
  n101 = Bundle By Name(cluster=T20 {"Other AlliGator Ctrl Refnums"={"State Indicators"=refnum, " Progress Bar"=refnum, "Decay Graph Active"=refnum, "Decay Statistics Bin"=refnum, "Time Step"=refnum, "Use File Timestamp"=refnum, "Tab Control"=refnum, "CPU"=refnum, "Abort Fit"=refnum, "Dataset File/Folder Path"=refnum, "Abort ROI Creation"=refnum, "Event LED"=refnum, "Dataset File/Folder Path 2"=refnum, "Dataset File/Folder Path 3"=refnum, "Dataset File/Folder Path 4"=refnum, "Dataset File/Folder Path 5"=refnum, "Dataset File/Folder Path 6"=refnum, "Dataset File/Folder Path 7"=refnum, "Dataset File/Folder Path 8"=refnum, "Dataset File/Folder Path 9"=refnum, "Dataset File/Folder Path 10"=refnum, "Dataset File/Folder Path 11"=refnum}, "Phasor Plot Ctrl Refnums"={"Phasor Ratio"=refnum, "Modulus Lifetime"=refnum, "Phasor at cursor (m, phi)"=refnum, "Phase Lifetime"=refnum, "Phasor at cursor (g, s)"=refnum, "Phasor Plor Average Lifetime"=refnum, "Phasor Plot Active"=refnum, "Save Phasor Plot"=refnum, "Image Overlay Color"=refnum, "Phasor Plot Color Scale"=refnum, "Reference 1 Button"=refnum, "Reference 2 Button"=refnum}, "Phasor Graph Ctrl Refnums"={"Phasor Ratio"=refnum, "Modulus Lifetime"=refnum, "Phasor at cursor (m, phi)"=refnum, "Phase Lifetime"=refnum, "Phasor at cursor (g, s)"=refnum, "Phasor Graph Average Lifetime"=refnum, "Phasor Graph Active"=refnum, "Save Phasor Graph"=refnum, "Phasor Frame Slide"=refnum, "Single Step Phasor"=refnum, "Calibration Type"=refnum, "Show Line"=refnum, "Phase Lifetime 1"=refnum, "Phase Lifetime 2"=refnum, "Phasor Graph Frequency"=refnum, "Phasor Reference 1 Control"=refnum, "Phasor Reference 2 Control"=refnum, "Calibration Lifetime"=refnum, "Phase Lifetime SDV"=refnum, "Average Lifetime SDV"=refnum, "Phasor Ratio SDV"=refnum, "Modulus Lifetime SDV"=refnum}, "Dataset Control References"={"Current Data"=refnum, "Gate Image Slide"=refnum, "Time Point Slide"=refnum, "Current Time Stamp"=refnum, "Save Image"=refnum, "Displayed Image"=refnum, "Overlay Mode"=refnum, "Phasor Overlay Color"=refnum, "Image Color Scale"=refnum, "Use ROI as Search Area"=refnum, "Source Image ROI Color"=refnum}, "Registered Events Ctrl Refnums"={"Time Point Slider"=refnum, "Phasor Plot Display Range"=refnum, "Decay Graph"=refnum, "Decay Statistics Graph"=refnum, "Intensity Time Trace"=refnum, "Phasor Graph"=refnum, "Phasor Ratio Graph"=refnum, "Lifetime Graph"=refnum, "Phasor Plot Display"=refnum, "Source Image Display"=refnum, "Decay Fit Parameter Map Display Range"=refnum, "Decay Fit Parameter Map Display"=refnum}, "Image Histogram Ctrl Refnums"={"Image Histogram"=refnum, "Image Histogram Options"=refnum, "Image Histogram Active"=refnum, "Image Histogram Upper Percentile"=refnum, "Image Histogram Lower Percentile"=refnum, "Auto-Adjust Contrast"=refnum}, "Decay Fit Map Ctrl Refums"={"Decay Fit Parameter Map Color Scale"=refnum, "Decay Fit Parameter"=refnum, "Max Parameter"=refnum, "Min Parameter"=refnum, "Decay Fit Parameter Map Display"=refnum, "Decay Fit Parameter Map Display Range"=refnum}} ("AlliGator Ctrl Refnums"), "Decay Fit Map Ctrl Refums"=w66, "Image Histogram Ctrl Refnums"=w73, "Other AlliGator Ctrl Refnums"=w5, "Phasor Plot Ctrl Refnums"=w106, "Phasor Graph Ctrl Refnums"=w39, "Dataset Control References"=w105, "Registered Events Ctrl Refnums"=w35) -> (w61:T20)
  n102 = Enqueue Element(queue=w158, element=T25[] [{"AlliGator Q Event"=enum."GUI:Initialization", "Data"=variant}] ("Named Q Element"), error in (no error)=w150) -> (queue out=w157:refnum<queue>, error out=w50:errorcluster)  [unwired: 1 in, 1 out]
  n103 = invoke class="VI" method="FP.Open"(error in=w50, "State"=T13."Hidden" ("Front Panel Window:State")) -> (reference out=w40:refnum<vi>, error out=w29:errorcluster)  [unwired: 3 in, 3 out]
  n104 = invoke class="VI" method="Default Vals.Reinit All"(reference=w40, error in=w29) -> (reference out=w30:refnum<vi>, error out=w28:errorcluster)  [unwired: 1 in, 1 out]
  n105 = Current VI's Path() -> (path=w47:path)
  n106 = call "AlliGator Register Control Events.vi"("Error In"=w28, "AlliGator Control References"=w35) -> ("Error Out"=w16:errorcluster, "AlliGator Event Registration"=w121:T26)  [unwired: 8 in]
  n107 = call "AlliGator Get-Set Control References.vi"("Get(F)/Set"=TRUE, "Error In"=w16, "AlliGator Ctrl Refnums in"=w61) -> ("Error Out"=w19:errorcluster, "AlliGator Ctrl Refnums out"=w4:T20)  [unwired: 7 in]
  n108 = call "Get App Kind, Name & Path.vi"("Error In"=w19, "Callling VI Path"=w47) -> ("Error Out"=w43:errorcluster, "Application Path"=w45:path)  [unwired: 6 in, 2 out]
  n109 = Build Path(base path=w45, name or relative path="AlliGator Action Loop.vi") -> (appended path=w15:path)
  n110 = call "Embedded Progress Bar Q.vi"("Progress Bar Queue Name"="AlliGator Progress Bar Q") -> ("Progress Bar Queue"=w33:refnum<queue>)  [unwired: 6 in]
  n111 = while {
    tunnel: w33 -> [w164]
    tunnel: w119 -> [w162]
    tunnel: [w159] -> w34
    stop <- w160 stop-if-true
    n112 = Dequeue Element(queue=w164) -> (element=w163:T27, error out=w161:errorcluster)  [unwired: 2 in, 2 out]
    n113 = call "Update Embedded Progress Bar Indicator.vi"("Error In"=w161, "Progress Bar Event"=w163, "Progress Bar Refnum"=w162) -> ("Error Out"=w159:errorcluster, "Quit?"=w160:bool)  [unwired: 7 in]
  }
  n114 = call <vilib>:"Initialize Mouse.vi"() -> ("error out"=w137:errorcluster, "device ID"=w138:refnum<k1>)  [unwired: 10 in]
  n115 = call <vilib>:"Intialize Keyboard.vi"() -> ("error out"=w116:errorcluster, "device ID"=w117:refnum<k1>)  [unwired: 10 in]
  n116 = vi-ref "AlliGator Action Engine.lvlib:AlliGator Action Loop.vi"() -> (w44:refnum<vi>)
  n117 = Current VI's Menubar() -> (w155:refnum<k9>)
  n118 = Open VI Reference(type specifier VI Refnum (for type only)=w44, vi path=w15, options=128, error in (no error)=w43) -> (vi reference=w3:refnum<vi>, error out=w62:errorcluster)  [unwired: 2 in]
  n119 = call-by-ref "Start Asynchronous Call"(reference=w3, error in=w62, "AlliGator Ctrl Refnums"=w4, "AlliGator Refnum"=w30) -> (error out=w37:errorcluster)  [unwired: 9 in, 2 out]
  n120 = while {
    tunnel: w157 -> [w169]
    tunnel: w155 -> [w195]
    shift-right: [w194] -> w154
    shift-left: w121 -> [w193]
    tunnel: "AlliGator" ("Sender") -> [w192]
    tunnel: w59 -> [w168]
    tunnel: w138 -> [w190]
    tunnel: w137 -> [w189]
    tunnel: [w188] -> w136
    tunnel: [w187] -> w135
    tunnel: w117 -> [w186]
    tunnel: w116 -> [w185]
    tunnel: [w184] -> w115
    tunnel: [w183] -> w114
    tunnel: w37 -> [_]
    tunnel: w30 -> [w178]
    tunnel: "Busy" ("t") -> [w170]
    tunnel: u32 30 ("Mouse Move Timeout") -> [w167]
    tunnel: w15 -> [w166]
    tunnel: w4 -> [w165]
    stop <- w171 stop-if-true
    # "do not add events to the stack when busy icon is on (F)"
    # "Event Loop"
    n121 = local read "Animated Busy Icon"() -> (w191:bool)
    n122 = event shown="[116] Menu Selection (User)" {
      selector: w193 -> [_ _ _ _ _ _ _ _ _ _ _ _ _ _ _ _ _ _ _ _ _ _ _ _ _ _ _ _ _ _ _ _ _ _ _ _ _ _ _ _ _ _ _ _ _ _ _ _ _ _ _ _ _ _ _ _ _ _ _ _ _ _ _ _ _ _ _ _ _ _ _ _ _ w1324 w1341 _ w1371 w1382 w1389 w1412 w1425 _ w1451 w1464 _ w1490 w1503 _ w1529 w1542 _ _ _ w1624 w1631 w1654 w1663 w1676 _ w1704 w1732 w1749 _ w1831 w1868 w1881 _ w1907 w1935 w1952 _ w2020 w2047 _ w2088 _ _ _ _ _ _ _]
      dyn-events: [_ _ _ _ _ _ _ _ _ _ _ _ _ _ _ _ _ _ _ _ _ _ _ _ _ _ _ _ _ _ _ _ _ _ _ _ _ _ _ _ _ _ _ _ _ _ _ _ _ _ _ _ _ _ _ _ _ _ _ _ _ _ _ _ _ _ _ _ _ _ _ _ _ w1325 w1342 _ w1372 w1383 w1389 w1410 w1424 _ w1449 w1463 _ w1488 w1502 _ w1527 w1541 _ _ _ w1625 w1631 w1655 w1661 w1675 _ w1703 w1733 w1750 _ w1830 w1866 w1880 _ w1908 w1936 w1953 _ w2019 w2048 _ w2089 _ _ _ _ _ _ _] -> w194
      timeout: _ -> [_ _ _ _ _ _ _ _ _ _ _ _ _ _ _ _ _ _ _ _ _ _ _ _ _ _ _ _ _ _ _ _ _ _ _ _ _ _ _ _ _ _ _ _ _ _ _ _ _ _ _ _ _ _ _ _ _ _ _ _ _ _ _ _ _ _ _ _ _ _ _ _ _ _ _ _ _ _ _ _ _ _ _ _ _ _ _ _ _ _ _ _ _ _ _ _ _ _ _ _ _ _ _ _ _ _ _ _ _ _ _ _ _ _ _ _ _ _ _ _ _ _]
      tunnel: [_ _ _ _ _ _ _ _ _ _ _ _ _ _ _ _ _ _ _ _ _ _ _ _ _ _ _ _ _ _ _ _ _ _ _ _ _ _ _ _ _ _ _ _ _ _ _ _ _ _ _ _ _ _ _ _ _ _ _ _ _ _ _ _ _ _ _ _ _ _ _ _ _ _ _ _ _ _ _ _ _ _ _ _ _ _ _ _ _ _ _ _ _ _ _ _ _ _ _ _ _ _ _ _ _ _ _ _ _ _ _ _ _ _ _ _ w2137 _ _ _ _ w2177] -> w171
      tunnel: w169 -> [_ _ _ _ _ _ _ _ _ _ _ _ _ _ _ _ _ _ _ _ _ _ _ _ _ _ _ _ _ _ _ _ _ _ _ _ _ _ _ _ _ _ _ _ _ _ _ _ _ _ _ _ w985 w1002 w1016 w1025 _ _ _ _ _ _ _ _ _ _ _ _ _ _ _ _ w1310 _ _ _ _ _ _ _ _ _ _ _ _ _ _ _ _ _ _ _ _ _ _ _ _ _ _ _ _ _ _ _ _ _ _ _ _ _ _ _ _ _ _ _ _ _ _ _ _ _]
      tunnel: w195 -> [_ _ _ _ _ w243 _ _ _ _ _ _ _ _ _ _ _ _ _ _ _ _ _ _ _ _ _ _ _ _ _ _ _ _ _ _ _ _ _ _ _ _ _ _ _ _ _ _ _ _ _ _ _ _ _ _ _ _ _ _ _ _ _ _ _ _ _ _ _ _ _ _ _ _ _ _ _ _ _ _ _ _ _ _ _ _ _ _ _ _ _ _ _ _ _ _ _ _ _ _ _ _ _ _ _ _ _ _ _ _ _ _ _ _ _ _ _ _ _ _ _ _]
      tunnel: w192 -> [_ _ _ _ _ w240 _ _ _ _ _ _ _ _ _ _ _ _ _ _ _ _ _ _ _ _ _ _ _ _ _ _ _ w600 _ _ _ _ w681 _ _ _ _ _ _ _ _ _ _ _ _ _ _ _ _ _ _ _ _ _ _ w1079 _ _ _ _ _ _ _ w1246 _ w1279 _ _ _ _ _ _ _ _ _ _ _ _ _ _ _ _ _ _ _ w1567 _ _ _ _ _ _ _ _ _ _ _ _ _ _ _ _ _ _ _ _ _ _ _ _ _ _ _ _ _ w2183]
      tunnel: w191 -> [_ _ _ _ w228 w239 _ _ w280 _ _ w299 w309 w316 w332 w339 _ _ w382 _ w435 _ w455 w479 w490 w505 w520 w527 w534 _ w550 _ _ w598 _ w647 w656 _ _ _ w761 w782 w796 _ _ _ w841 _ w882 _ _ w944 w983 w1000 w1015 w1024 _ _ w1051 w1059 w1067 w1077 w1099 _ w1128 _ _ w1188 w1226 _ w1259 w1276 w1308 w1323 w1340 w1356 _ _ w1392 _ _ _ _ _ _ _ _ _ _ _ _ _ w1610 _ w1634 _ _ _ _ w1695 w1725 w1748 w1763 w1833 _ _ _ w1901 w1928 w1951 w1970 w2013 w2046 w2065 w2087 w2109 w2134 w2148 w2155 _ _ w2184]
      tunnel: w170 -> [_ _ _ _ w225 _ _ _ _ _ _ _ w306 _ w330 _ _ _ _ _ _ _ _ _ _ _ _ _ _ _ _ _ _ _ _ _ _ _ _ _ _ _ _ _ _ _ _ _ _ _ _ w942 _ _ _ _ _ _ _ _ _ _ _ _ _ _ _ _ _ _ _ _ _ _ _ _ _ _ _ _ _ _ _ _ _ _ _ _ _ _ _ _ _ _ _ _ _ _ _ _ _ _ _ _ _ _ _ _ _ _ _ _ _ _ _ _ w2147 _ _ _ _ _]
      tunnel: w190 -> [w200 w204 w209 w216 w224 w237 w267 w273 w279 w286 w292 w298 w305 w315 w329 w338 w352 w365 w392 w428 w434 w448 w471 w476 w487 w502 w519 w526 w533 w541 w549 w561 w583 w597 w632 w646 w653 w668 w683 w744 w766 w781 w798 w816 w825 w832 w840 w855 w885 w923 w930 w941 w980 w997 w1014 w1023 w1037 w1044 w1050 w1058 w1066 w1075 w1096 w1120 w1125 w1150 w1163 w1191 w1224 w1243 w1256 w1274 w1305 w1321 w1338 w1352 w1368 w1379 w1391 w1409 w1419 w1437 w1448 w1458 w1476 w1487 w1497 w1515 w1526 w1536 w1554 w1566 w1609 w1619 w1633 w1651 w1660 w1670 w1688 w1700 w1730 w1746 w1770 w1828 w1865 w1875 w1893 w1905 w1933 w1949 w1973 w2018 w2044 w2064 w2085 w2108 w2146 w2153 w2160 w2167 w2176 w2182]
      tunnel: w189 -> [w199 w203 w208 w215 w223 w236 w266 w272 w278 w285 w291 w297 w304 w314 w328 w337 w351 w364 w391 w427 w433 w447 w470 w475 w486 w501 w518 w525 w532 w540 w548 w560 w582 w596 w631 w645 w652 w667 w682 w743 w765 w780 w797 w815 w824 w831 w839 w854 w884 w922 w929 w940 w979 w996 w1013 w1022 w1036 w1043 w1049 w1057 w1065 w1074 w1095 w1119 w1124 w1149 w1162 w1190 w1223 w1242 w1255 w1273 w1304 w1320 w1337 w1351 w1367 w1378 w1390 w1408 w1418 w1436 w1447 w1457 w1475 w1486 w1496 w1514 w1525 w1535 w1553 w1565 w1608 w1618 w1632 w1650 w1659 w1669 w1687 w1699 w1729 w1745 w1771 w1827 w1864 w1874 w1892 w1904 w1932 w1948 w1972 w2017 w2043 w2063 w2084 w2107 w2145 w2152 w2159 w2166 w2175 w2181]
      tunnel: [w200 w204 w209 w216 w224 w237 w267 w273 w279 w286 w292 w298 w305 w315 w329 w338 w352 w365 w392 w428 w434 w448 w471 w476 w487 w502 w519 w526 w533 w541 w549 w561 w583 w597 w632 w646 w653 w668 w683 w744 w766 w781 w798 w816 w825 w832 w840 w855 w885 w923 w930 w941 w980 w997 w1014 w1023 w1037 w1044 w1050 w1058 w1066 w1075 w1096 w1120 w1125 w1150 w1163 w1191 w1224 w1243 w1256 w1274 w1305 w1321 w1338 w1352 w1368 w1379 w1391 w1409 w1419 w1437 w1448 w1458 w1476 w1487 w1497 w1515 w1526 w1536 w1554 w1566 w1609 w1619 w1633 w1651 w1660 w1670 w1688 w1700 w1730 w1746 w1769 w1828 w1865 w1875 w1893 w1905 w1933 w1949 w1973 w2018 w2044 w2064 w2085 w2108 w2146 w2153 w2160 w2167 w2176 w2182] -> w188
      tunnel: [w199 w203 w208 w215 w223 w236 w266 w272 w278 w285 w291 w297 w304 w314 w328 w337 w351 w364 w391 w427 w433 w447 w470 w475 w486 w501 w518 w525 w532 w540 w548 w560 w582 w596 w631 w645 w652 w667 w682 w743 w765 w780 w797 w815 w824 w831 w839 w854 w884 w922 w929 w940 w979 w996 w1013 w1022 w1036 w1043 w1049 w1057 w1065 w1074 w1095 w1119 w1124 w1149 w1162 w1190 w1223 w1242 w1255 w1273 w1304 w1320 w1337 w1351 w1367 w1378 w1390 w1408 w1418 w1436 w1447 w1457 w1475 w1486 w1496 w1514 w1525 w1535 w1553 w1565 w1608 w1618 w1632 w1650 w1659 w1669 w1687 w1699 w1729 w1745 w1768 w1827 w1864 w1874 w1892 w1904 w1932 w1948 w1972 w2017 w2043 w2063 w2084 w2107 w2145 w2152 w2159 w2166 w2175 w2181] -> w187
      tunnel: [_ _ _ w212 _ _ w263 w269 _ w282 w288 _ _ _ _ _ _ w354 w380 _ _ w444 w453 _ _ _ _ _ _ w537 _ w557 _ w593 w626 _ _ w664 w675 w740 _ _ w785 w812 w820 _ _ w848 w874 _ _ _ _ _ _ _ w1033 w1040 _ _ _ w1071 _ _ _ _ w1153 w1179 w1220 w1249 w1252 w1270 _ w1317 w1334 _ w1362 w1373 _ w1407 w1417 w1435 w1444 w1456 w1474 w1485 w1495 w1513 w1524 w1534 w1552 w1564 _ w1615 _ w1645 w1658 w1668 w1686 w1698 w1726 w1742 _ w1825 w1863 w1873 w1891 w1900 w1929 w1945 _ w2010 w2040 _ w2081 w2104 w2131 _ _ _ _ _] -> w175
      tunnel: w186 -> [w197 w202 w207 w214 w222 w235 w265 w271 w277 w284 w290 w296 w303 w313 w327 w336 w349 w363 w386 w425 w431 w446 w465 w474 w485 w500 w517 w524 w531 w539 w546 w559 w585 w595 w630 w644 w651 w666 w679 w742 w764 w779 w790 w814 w823 w830 w838 w853 w879 w920 w927 w939 w978 w995 w1012 w1021 w1035 w1042 w1048 w1056 w1064 w1073 w1094 w1117 w1123 w1148 w1161 w1185 w1222 w1241 w1254 w1272 w1303 w1319 w1336 w1355 w1364 w1375 w1388 w1406 w1416 w1434 w1446 w1455 w1473 w1484 w1494 w1512 w1523 w1533 w1551 w1563 w1607 w1617 w1630 w1647 w1657 w1667 w1685 w1697 w1728 w1744 w1764 w1824 w1862 w1872 w1890 w1903 w1931 w1947 w1966 w2016 w2042 w2061 w2083 w2106 w2143 w2150 w2157 w2164 w2173 w2180]
      tunnel: w185 -> [w196 w201 w206 w213 w221 w234 w264 w270 w276 w283 w289 w295 w302 w312 w326 w335 w350 w362 w387 w426 w430 w445 w463 w473 w484 w499 w516 w523 w530 w538 w547 w558 w584 w594 w629 w643 w650 w665 w678 w741 w763 w778 w791 w813 w822 w829 w837 w852 w880 w921 w928 w938 w977 w994 w1011 w1020 w1034 w1041 w1047 w1055 w1063 w1072 w1093 w1118 w1122 w1147 w1160 w1183 w1221 w1240 w1253 w1271 w1302 w1318 w1335 w1354 w1363 w1374 w1387 w1405 w1415 w1433 w1445 w1454 w1472 w1483 w1493 w1511 w1522 w1532 w1550 w1562 w1606 w1616 w1629 w1646 w1656 w1666 w1684 w1696 w1727 w1743 w1766 w1823 w1861 w1871 w1889 w1902 w1930 w1946 w1969 w2015 w2041 w2060 w2082 w2105 w2142 w2151 w2158 w2165 w2174 w2179]
      tunnel: [w196 w201 w206 w213 w221 w234 w264 w270 w276 w283 w289 w295 w302 w312 w326 w335 w350 w362 w385 w426 w430 w445 w464 w473 w484 w499 w516 w523 w530 w538 w547 w558 w584 w594 w629 w643 w650 w665 w678 w741 w763 w778 w788 w813 w822 w829 w837 w852 w876 w921 w928 w938 w977 w994 w1011 w1020 w1034 w1041 w1047 w1055 w1063 w1072 w1093 w1118 w1122 w1147 w1160 w1184 w1221 w1240 w1253 w1271 w1302 w1318 w1335 w1354 w1363 w1374 w1387 w1405 w1415 w1433 w1445 w1454 w1472 w1483 w1493 w1511 w1522 w1532 w1550 w1562 w1606 w1616 w1629 w1646 w1656 w1666 w1684 w1696 w1727 w1743 w1767 w1823 w1861 w1871 w1889 w1902 w1930 w1946 w1968 w2015 w2041 w2060 w2082 w2105 w2141 w2151 w2158 w2165 w2174 w2179] -> w184
      tunnel: [w197 w202 w207 w214 w222 w235 w265 w271 w277 w284 w290 w296 w303 w313 w327 w336 w349 w363 w384 w425 w431 w446 w466 w474 w485 w500 w517 w524 w531 w539 w546 w559 w585 w595 w630 w644 w651 w666 w679 w742 w764 w779 w789 w814 w823 w830 w838 w853 w878 w920 w927 w939 w978 w995 w1012 w1021 w1035 w1042 w1048 w1056 w1064 w1073 w1094 w1117 w1123 w1148 w1161 w1186 w1222 w1241 w1254 w1272 w1303 w1319 w1336 w1355 w1364 w1375 w1388 w1406 w1416 w1434 w1446 w1455 w1473 w1484 w1494 w1512 w1523 w1533 w1551 w1563 w1607 w1617 w1630 w1647 w1657 w1667 w1685 w1697 w1728 w1744 w1765 w1824 w1862 w1872 w1890 w1903 w1931 w1947 w1967 w2016 w2042 w2061 w2083 w2106 w2140 w2150 w2157 w2164 w2173 w2180] -> w183
      tunnel: w178 -> [_ _ _ _ _ _ _ _ _ _ _ _ _ _ _ _ _ _ _ _ _ _ _ _ _ _ _ _ _ _ _ _ _ _ _ _ _ _ _ _ _ _ _ _ _ _ _ _ _ _ _ _ _ _ _ _ _ _ _ _ _ _ _ _ _ _ _ _ _ _ _ _ _ _ _ _ _ _ _ _ _ _ _ _ _ _ _ _ _ _ _ w1561 _ _ _ _ _ _ _ _ _ _ _ _ _ _ _ _ _ _ _ _ _ _ _ w2103 w2127 _ _ _ _ _]
      tunnel: [_ _ _ T25[] [{"AlliGator Q Event"=enum."Image:Image Histogram", "Data"=variant}, {"AlliGator Q Event"=enum."Image:Image Contrast", "Data"=variant}] ("AlliGator Actions") w220 w233 _ _ w275 _ _ w294 w301 w311 w323 w334 w346 _ w389 _ w429 _ w462 w472 w483 w498 w515 w522 w529 T25[] [{"AlliGator Q Event"=enum."Image:Image Histogram", "Data"=variant}] ("AlliGator Actions") w545 T25[] [{"AlliGator Q Event"=enum."Image:Image Histogram", "Data"=variant}, {"AlliGator Q Event"=enum."Image:Image Contrast", "Data"=variant}] ("AlliGator Actions") w577 w592 _ w642 w649 _ w676 _ w762 w777 w784 _ _ _ w836 _ w881 _ w924 w935 w976 w993 w1010 w1019 _ _ w1046 w1054 w1062 w1070 w1092 _ w1121 _ _ w1181 w1219 _ w1251 w1269 w1301 _ _ w1353 _ _ w1386 _ _ _ _ _ _ _ _ _ _ _ _ _ w1605 _ w1627 _ _ _ _ _ _ _ w1762 w1822 _ _ _ _ _ _ w1971 w2014 _ w2059 w2080 _ w2126 w2149 w2156 _ _ w2178] -> w177
      tunnel: [_ _ _ _ _ _ _ _ _ _ _ _ _ _ _ _ _ _ w381 _ _ _ w452 _ _ _ _ _ _ _ _ _ _ w591 _ _ _ _ w674 _ _ _ w786 _ _ _ _ _ w875 _ _ _ _ _ _ _ _ _ _ _ _ _ _ _ _ _ _ w1180 _ w1236 _ w1268 _ _ _ _ _ _ _ _ _ _ _ _ _ _ _ _ _ _ _ _ _ _ _ _ _ _ _ _ _ _ _ _ _ _ _ _ _ _ _ _ _ _ _ _ w2135 _ _ _ _ _] -> w172
      tunnel: w167 -> [_ _ _ _ _ _ _ _ _ _ _ _ _ _ _ _ _ _ _ _ _ _ _ _ _ _ _ _ _ _ _ _ w576 _ _ _ _ _ _ _ w759 _ _ _ _ _ _ _ _ _ _ _ _ _ _ _ _ _ _ _ _ _ _ _ _ _ _ _ _ _ _ _ _ _ _ _ _ _ w1384 _ _ w1427 _ _ w1465 _ _ w1504 _ _ w1543 _ _ _ w1626 _ _ _ w1677 _ _ _ w1760 _ _ _ w1882 _ _ _ w1963 _ _ w2057 _ _ _ _ _ _ _ _]
      tunnel: w166 -> [_ _ _ _ _ _ _ _ _ _ _ _ _ _ _ _ _ _ _ _ _ _ _ _ _ _ _ _ _ _ _ _ _ _ _ _ _ _ _ _ _ _ _ _ _ _ _ _ _ _ _ _ _ _ _ _ _ _ _ _ _ _ _ _ _ _ _ _ _ _ _ _ _ _ _ _ _ _ _ _ _ _ _ _ _ _ _ _ _ _ _ _ _ _ _ _ _ _ _ _ _ _ _ _ _ _ _ _ _ _ _ _ _ _ _ w2102 _ _ _ _ _ _]
      tunnel: w165 -> [_ _ _ _ _ _ _ _ _ _ _ _ _ _ _ _ _ _ _ _ _ _ _ _ _ _ _ _ _ _ _ _ _ _ _ _ _ _ _ _ _ _ _ _ _ _ _ _ _ _ _ _ _ _ _ _ _ _ _ _ _ _ _ _ _ _ _ _ _ _ _ _ _ _ _ _ _ _ _ _ _ _ _ _ _ _ _ _ _ _ _ _ _ _ _ _ _ _ _ _ _ _ _ _ _ _ _ _ _ _ _ _ _ _ _ _ _ _ _ w2163 w2168 _]
      event "Abort Fit": Value Change {
        w198 = TRUE ("Abort?")
        n123 = event-data() -> ()  [unwired: 1 in, 1 out]
        n124 = global write "Abort Fit Global.vi" "Abort Fit"(w198) -> ()
        n125 = global write "Phasor Abort Parallel Computation.vi" "Abort Parallel Computation"(w198) -> ()
      }
      event "Abort ROI Creation": Value Change {
        n126 = event-data() -> ()  [unwired: 1 in, 1 out]
        n127 = global write "Abort ROI Creation Global.vi" "Abort ROI Creation"(TRUE ("Abort?")) -> ()
      }
      event "Abort": Value Change {
        n128 = event-data() -> ()  [unwired: 1 in, 1 out]
        n129 = global write "AlliGator Abort.vi" "Abort?"(TRUE ("Abort?")) -> ()
      }
      event "Auto-Adjust Contrast": Value Change {
        # "This is not part of the Settings Window and needs to be handled separately"
        n130 = event-data() -> ("NewVal"=w219:bool)  [unwired: 1 in]
        n131 = call "AlliGator Settings Storage.vi"("Get(F)/Set"=TRUE, "AlliGator Settings List"=AlliGator_Settings_List."Source Image:Auto-Adjust Contrast", "Variant Data in"=w219) -> ("Error Out"=w212:errorcluster)  [unwired: 7 in, 1 out]
      }
      event "Calibration Lifetime": Shortcut Menu Selection (User) {
        n132 = event-data() -> ("ItemTag"=w226:string)  [unwired: 1 in]
        n133 = Select(t=w226, s=w228, f=w225) -> (s? t:f=w227:string)
        n134 = case shown="\"Use as Phasor Reference 1 Lifetime\"" w227 {
          tunnel: [_ w229 w231] -> w220
          frame Default {
          }
          frame "Use as Phasor Reference 1 Lifetime" {
            n135 = Build Array(T25 {"AlliGator Q Event"=enum."Phasor Ratio:Use as Phasor Reference 1 Lifetime", "Data"=variant} ("element")) -> (w229:T25[])
          }
          frame "Use as Phasor Reference 2 Lifetime" {
            n136 = Build Array(T25 {"AlliGator Q Event"=enum."Phasor Ratio:Use as Phasor Reference 2 Lifetime", "Data"=variant} ("element")) -> (w231:T25[])
          }
        }
      }
      event Value Change {
        n137 = event-data() -> ("CtlRef"=w242:refnum<vi>, "OldVal"=w241:T9, "NewVal"=w238:T9)  [unwired: 1 in]
        n138 = case shown="True" w239 {
          tunnel: w243 -> [_ w253]
          tunnel: w242 -> [w245 _]
          tunnel: w241 -> [w244 _]
          tunnel: w240 -> [_ _]
          tunnel: w238 -> [_ w250]
          tunnel: [_ w246] -> w233
          frame False {
            n139 = property class="Enum (strict)"(reference=w245, "Value"=w244) -> ()  [unwired: 1 in, 2 out]
          }
          frame True {
            n140 = Bundle By Name(cluster=T25 {"AlliGator Q Event"=enum."Calibration:Set Calibration Type", "Data"=variant} ("element"), "Data"=w250) -> (w251:T25)
            n141 = case shown="\"Phasor Map\"" w250 {
              tunnel: [_ TRUE ("Use Calibration Phasor") FALSE ("Use Calibration Phasor") FALSE ("Use Calibration Phasor")] -> w249
              tunnel: [_ FALSE ("Use Calibration Phasor Curve") TRUE ("Use Calibration Phasor Curve") FALSE ("Use Calibration Phasor Curve")] -> w248
              tunnel: [_ FALSE ("Use Calibration Phasor Map") FALSE ("Use Calibration Phasor Map") TRUE ("Use Calibration Phasor Map")] -> w247
              frame "None", Default {
              }
              frame "Single Phasor" {
              }
              frame "Phasor Series" {
              }
              frame "Phasor Map" {
              }
            }
            n142 = Build Array(w251) -> (w246:T25[])
            n143 = call "AlliGator Check Calibration Menu Items.vi"("Use Calibration Phasor Map"=w247, "Use Calibration Phasor Curve"=w248, "Use Calibration Phasor"=w249, "Menu in"=w253) -> ()  [unwired: 7 in, 1 out]
          }
        }
      }
      event "Clear Image Overlay": Shortcut Menu Activation? {
        n144 = event-data() -> ("MenuRef"=w268:refnum<k9>)  [unwired: 1 in]
        n145 = call "AlliGator Set Check Marks in Source Image Overlay to Erase Button Menu.vi"("Menu in"=w268) -> ("Error Out"=w263:errorcluster)  [unwired: 10 in]
        n146 = event-data() -> ()  [unwired: 2 in, 1 out]
      }
      event "Clear Image Overlay": Shortcut Menu Selection (User) {
        n147 = event-data() -> ("ItemTag"=w274:string)  [unwired: 1 in]
        n148 = call "AlliGator Update Checkmarks in Source Image Overlay to Erase Button Menu.vi"("Source Image Overlay to Erase"=w274) -> ("Error Out"=w269:errorcluster)  [unwired: 10 in]
      }
      event "Clear Image Overlay": Value Change {
        n149 = event-data() -> ()  [unwired: 1 in, 1 out]
        n150 = case shown="True" w280 {
          tunnel: [_ T25[] [{"AlliGator Q Event"=enum."Image:Clear Image Overlay", "Data"=variant}, {"AlliGator Q Event"=enum."Image:Image Contrast", "Data"=variant}] ("element")] -> w275
          frame False {
          }
          frame True {
          }
        }
      }
      event "Clear Phasor Overlay": Shortcut Menu Activation? {
        n151 = event-data() -> ("MenuRef"=w287:refnum<k9>)  [unwired: 1 in]
        n152 = call "AlliGator Set Checkmarks in Phasor Overlay to Erase Button Menu.vi"("Menu in"=w287) -> ("Error Out"=w282:errorcluster)  [unwired: 10 in]
        n153 = event-data() -> ()  [unwired: 2 in, 1 out]
      }
      event "Clear Phasor Overlay": Shortcut Menu Selection (User) {
        n154 = event-data() -> ("ItemTag"=w293:string)  [unwired: 1 in]
        n155 = call "AlliGator Update Checkmarks in Phasor Overlay to Erase Button Menu.vi"("Phasor Plot Overlay to Erase"=w293) -> ("Error Out"=w288:errorcluster)  [unwired: 10 in]
      }
      event "Clear Phasor Overlay": Value Change {
        n156 = event-data() -> ()  [unwired: 1 in, 1 out]
        n157 = case shown="True" w299 {
          tunnel: [_ T25[] [{"AlliGator Q Event"=enum."Phasor Plot:Clear Phasor Overlay", "Data"=variant}] ("element")] -> w294
          frame False {
          }
          frame True {
          }
        }
      }
      event Shortcut Menu Selection (User) {
        n158 = event-data() -> ("ItemTag"=w307:string)  [unwired: 1 in]
        n159 = local read "Current Phasor (g, s)"() -> (w310:T8)
        n160 = Select(t=w307, s=w309, f=w306) -> (s? t:f=w308:string)
        n161 = call "AlliGator Current Phasor (g, s) Custom Menu Actions.vi"("Menu Item Tag"=w308, "Current Phasor"=w310) -> ("AlliGator Actions"=w301:T25[])  [unwired: 9 in]
      }
      event Value Change {
        n162 = event-data() -> ("NewVal"=w317:T8)  [unwired: 1 in]
        n163 = case shown="True" w316 {
          tunnel: w317 -> [_ w320]
          tunnel: [_ w319] -> w311
          frame False {
          }
          frame True {
            n164 = Build Array(w320) -> (w318:T8[])
            n165 = Bundle By Name(cluster=T25 {"AlliGator Q Event"=enum."Phasor Graph:Update Last Phasor Value", "Data"=variant} ("element"), "Data"=w318) -> (w321:T25)
            n166 = Build Array(w321) -> (w319:T25[])
          }
        }
      }
      event Shortcut Menu Selection (User) {
        n167 = event-data() -> ("ItemTag"=w331:string)  [unwired: 1 in]
        n168 = local read "Current Phasor (m, phi)"() -> (w333:T7)
        n169 = Select(t=w331, s=w332, f=w330) -> (s? t:f=w324:string)
        n170 = call "Phasor Convert (m, phi) to (g,s).vi"("Phasor (m, phi)"=w333) -> ("Phasor (g, s)"=w325:T8)  [unwired: 8 in]
        n171 = call "AlliGator Current Phasor (g, s) Custom Menu Actions.vi"("Menu Item Tag"=w324, "Current Phasor"=w325) -> ("AlliGator Actions"=w323:T25[])  [unwired: 9 in]
      }
      event Value Change {
        n172 = event-data() -> ("NewVal"=w340:T7)  [unwired: 1 in]
        n173 = case shown="True" w339 {
          tunnel: w340 -> [_ w342]
          tunnel: [_ w341] -> w334
          frame False {
          }
          frame True {
            n174 = Bundle By Name(cluster=T25 {"AlliGator Q Event"=enum."Phasor Graph:Update Phasor (m, phi)", "Data"=variant} ("element"), "Data"=w342) -> (w343:T25)
            n175 = Build Array(w343) -> (w341:T25[])
          }
        }
      }
      event "Dataset File/Folder Path", "Dataset File/Folder Path 2", "Dataset File/Folder Path 3", "Dataset File/Folder Path 4", "Dataset File/Folder Path 5", "Dataset File/Folder Path 6", "Dataset File/Folder Path 7", "Dataset File/Folder Path 8", "Dataset File/Folder Path 9", "Dataset File/Folder Path 10", "Dataset File/Folder Path 11": Value Change {
        n176 = event-data() -> ("NewVal"=w347:path)  [unwired: 1 in]
        n177 = Bundle By Name(cluster=T25 {"AlliGator Q Event"=enum."Files:Load File (all Types)_Scriptable", "Data"=variant} ("element"), "Data"=w347) -> (w345:T25)
        n178 = Build Array(w345) -> (w346:T25[])
        n179 = flat-sequence {
          tunnel: w345 -> [_]
          frame #0 {
            w353 = path "" ("File/Folder Path")
            n180 = local write "Dataset File/Folder Path 2"(w353) -> ()
            n181 = local write "Dataset File/Folder Path 3"(w353) -> ()
            n182 = local write "Dataset File/Folder Path 4"(w353) -> ()
            n183 = local write "Dataset File/Folder Path 5"(w353) -> ()
            n184 = local write "Dataset File/Folder Path 6"(w353) -> ()
            n185 = local write "Dataset File/Folder Path 7"(w353) -> ()
            n186 = local write "Dataset File/Folder Path 8"(w353) -> ()
            n187 = local write "Dataset File/Folder Path 9"(w353) -> ()
            n188 = local write "Dataset File/Folder Path 10"(w353) -> ()
            n189 = local write "Dataset File/Folder Path 11"(w353) -> ()
            n190 = local write "Dataset File/Folder Path"(w353) -> ()
          }
        }
      }
      event "Decay Fit Parameter Map Image": Shortcut Menu Activation? {
        w366 = AlliGator_Variables_List."Decay Fit Parameter Map:Palette List" ("Alligator Variable")
        n191 = event-data() -> ("CtlRef"=w357:refnum<vi>, "MenuRef"=w379:refnum<k9>)  [unwired: 1 in]
        n192 = call "Alligator Variables Storage.vi"("Get(F)/Set"=FALSE, "AlliGator Variable"=AlliGator_Variables_List."Decay Fit Parameter Map:Palette Information" ("Alligator Variable")) -> ("Error Out"=w375:errorcluster, "Data out"=w376:variant)  [unwired: 7 in, 1 out]
        n193 = call "Alligator Variables Storage.vi"("Get(F)/Set"=FALSE, "AlliGator Variable"=w366) -> ("Error Out"=w359:errorcluster, "Data out"=w370:variant)  [unwired: 7 in, 1 out]
        n194 = Variant To Data(error in=w375, type=T29 {"Palette Name [# Colors,int?,inv?]"="", "Palette Type"=0, "Palette Colors"=[], "Interpolate?"=FALSE} ("Image Display Palette Information"), Variant=w376) -> (data=w374:T29, error out=w361:errorcluster)
        n195 = call-poly "Variant to Data.vi"("Variant"=w370) -> ("String Array"=w369:string[])  [unwired: 8 in]
        n196 = Unbundle By Name(w374) -> ("Palette Name [# Colors,int?,inv?]"=w372:string)
        n197 = Merge Errors(w361, w359) -> (w360:errorcluster)
        n198 = call "Check Selected Palette in Menu.vi"("Error In"=w360, "Palette List"=w369, "Checked Palette"=w372, "Menu in"=w379) -> ("Error Out"=w358:errorcluster, "Stored Palette List"=w367:string[], "menu reference out"=w356:refnum<k9>)  [unwired: 5 in]
        n199 = call "Alligator Variables Storage.vi"("Get(F)/Set"=TRUE, "AlliGator Variable"=w366, "Error In"=w358, "Data in"=w367) -> ("Error Out"=w355:errorcluster)  [unwired: 5 in, 2 out]
        n200 = call "AlliGator Add Python Functions to Object Menu.vi"("error in (no error)"=w355, "Menu in"=w356, "Object Refnum"=w357) -> ("error out"=w354:errorcluster)  [unwired: 6 in, 2 out]
        n201 = event-data() -> ()  [unwired: 2 in, 1 out]
      }
      event "Decay Fit Parameter Map Image": Shortcut Menu Selection (User) {
        n202 = event-data() -> ("CtlRef"=w394:refnum<vi>, "ItemTag"=w390:string, "ItemPath"=w393:string, "Coords"=w388:T35)  [unwired: 1 in]
        n203 = call-poly <vilib>:"Acquire Input Data.vi"("device ID"=w386, "error in (no error)"=w387) -> ("device ID"=w384:refnum<k1>, "keys pressed"=w383:T49, "error out"=w385:errorcluster)  [unwired: 15 in]
        n204 = case shown="True" w382 {
          tunnel: w394 -> [_ w405]
          tunnel: w393 -> [_ w404]
          tunnel: w390 -> [_ w403]
          tunnel: [_ w402] -> w389
          tunnel: w388 -> [_ w401]
          tunnel: w383 -> [_ w397]
          tunnel: [_ w396] -> w381
          tunnel: [_ w395] -> w380
          frame False {
          }
          frame True {
            n205 = Index Array(array=w397) -> (element=w400:T32)  [unwired: 1 in]
            n206 = Equal?(x=w400, y=T32."H" ("element")) -> (x = y?=w398:bool)
            n207 = case shown="False" w398 {
              tunnel: w405 -> [w411 w417]
              tunnel: w404 -> [w409 _]
              tunnel: w403 -> [w410 w416]
              tunnel: [w413 _] -> w402
              tunnel: w401 -> [w408 _]
              tunnel: [_ w415] -> w396
              tunnel: [w406 w414] -> w395
              frame False {
                n208 = Bundle By Name(cluster=T33 {"Item Tag"="", "Image Control Refnum"=refnum, "Coords"={"Horizontal"=0, "Vertical"=0}, "Item Path"=""} ("Image Event Data"), "Image Control Refnum"=w411, "Item Tag"=w410, "Item Path"=w409, "Coords"=w408) -> (w407:T33)
                n209 = call "AlliGator Decay Fit Parameter Map Context Menu Handler.vi"("Image Event Data"=w407) -> ("Error Out"=w406:errorcluster, "AlliGator Actions"=w413:T25[])  [unwired: 9 in]
              }
              frame True {
                n210 = property class="ImageControl"(reference=w417) -> ("Label.Text"=w418:string)  [unwired: 1 in, 2 out]
                n211 = call "AlliGator Send Python Function Doc String to Notebook.vi"("Item Tag"=w416, "Target"=w418) -> ("Error Out"=w414:errorcluster, "Message"=w415:string)  [unwired: 8 in]
              }
            }
          }
        }
      }
      event "Decay Fit Parameter Map ROI Color": Value Change {
        n212 = event-data() -> ("NewVal"=w419:u32)  [unwired: 1 in]
        n213 = call <vilib>:"Color to RGB.vi"("Color"=w419) -> ("R"=w422:u8, "G"=w423:u8, "B"=w424:u8)  [unwired: 1 out]
        n214 = Bundle By Name(cluster=cluster{"Red":u8, "Green":u8, "Blue":u8} {"Red"=0, "Green"=0, "Blue"=0} ("ROI Color"), "Red"=w422, "Green"=w423, "Blue"=w424) -> (w421:cluster{"Red":u8, "Green":u8, "Blue":u8})
        n215 = property on="Decay Fit Parameter Map Image" class="ImageControl"("ROI Color"=w421) -> ()  [unwired: 2 in, 2 out]
      }
      event Value Change {
        n216 = event-data() -> ("NewVal"=w432:T11)  [unwired: 1 in]
        n217 = case shown="True" w435 {
          tunnel: w432 -> [_ w441]
          tunnel: [_ w436] -> w429
          frame False {
          }
          frame True {
            w438 = TRUE  # Parameter changed
            n218 = Bundle(cluster=T36 {"Parameter"=enum."Offset", "Parameter changed"=FALSE} ("output cluster"), "Parameter"=w441, "Parameter changed"=w438) -> (w439:T36)
            n219 = Bundle By Name(cluster=T25 {"AlliGator Q Event"=enum."Decay Fit Parameter Map:Build Decay Fit Parameter Map", "Data"=variant} ("Time-Gated Phasor Q Element"), "Data"=w439) -> (w442:T25)
            n220 = Build Array(w442, T25 {"AlliGator Q Event"=enum."Image:Update Image Profile Plots", "Data"=variant} ("Time-Gated Phasor Q Element")) -> (w436:T25[])
          }
        }
      }
      event "Decay Graph Active": Value Change {
        n221 = event-data() -> ("NewVal"=w451:bool)  [unwired: 1 in]
        n222 = call "AlliGator Settings Storage.vi"("Get(F)/Set"=TRUE, "AlliGator Settings List"=AlliGator_Settings_List."Fluorescence Decay:Decay Graph Active", "Variant Data in"=w451) -> ("Error Out"=w444:errorcluster)  [unwired: 7 in, 1 out]
      }
      event "Decay Graph", "Decay Statistics Graph", "Intensity Time Trace", "Image Histogram": Shortcut Menu Selection (User) {
        # "Shortcut Menu (User)"
        n223 = event-data() -> ("CtlRef"=w457:refnum<vi>, "Coords"=w460:T35, "ItemTag"=w459:string, "ItemPath"=w458:string)  [unwired: 1 in]
        n224 = call-poly <vilib>:"Acquire Input Data.vi"("device ID"=w465, "error in (no error)"=w463) -> ("device ID"=w466:refnum<k1>, "keys pressed"=w467:T49, "error out"=w464:errorcluster)  [unwired: 15 in]
        n225 = Index Array(array=w467) -> (element=w469:T32)  [unwired: 1 in]
        n226 = Equal?(x=w469, y=T32."H" ("element")) -> (x = y?=w454:bool)
        n227 = Bundle By Name(cluster=T37 {"Item Tag"="", "XY Graph Refnum"=refnum, "Coords"={"Horizontal"=0, "Vertical"=0}, "Item Path"=""} ("XY Graph Event"), "XY Graph Refnum"=w457, "Coords"=w460, "Item Tag"=w459, "Item Path"=w458) -> (w456:T37)
        n228 = call "AlliGator Special Graph Menu Actions.vi"("Help?"=w454, "Animated Busy Icon"=w455, "XY Graph Event"=w456) -> ("Error Out"=w453:errorcluster, "Message"=w452:string, "AlliGator Actions"=w462:T25[])  [unwired: 6 in]
      }
      event "Decay Statistics Bin": Value Change {
        n229 = event-data() -> ("CtlRef"=w478:refnum<vi>, "OldVal"=w477:i32)  [unwired: 1 in]
        n230 = case shown="True" w479 {
          tunnel: w478 -> [w481 _]
          tunnel: w477 -> [w480 _]
          tunnel: [_ T25[] [{"AlliGator Q Event"=enum."FLI Dataset:Update Decay Statistics Graph", "Data"=variant}] ("element")] -> w472
          frame False {
            n231 = property class="DigNum (strict)"(reference=w481, "Value"=w480) -> ()  [unwired: 1 in, 2 out]
          }
          frame True {
          }
        }
      }
      event Value Change {
        n232 = event-data() -> ("CtlRef"=w488:refnum<vi>, "NewVal"=w489:T2)  [unwired: 1 in]
        n233 = case shown="True" w490 {
          tunnel: w489 -> [w492 w494]
          tunnel: w488 -> [w491 _]
          tunnel: [_ w493] -> w483
          frame False {
            n234 = property class="Enum (strict)"(reference=w491, "Value"=w492) -> ()  [unwired: 1 in, 2 out]
          }
          frame True {
            n235 = Bundle By Name(cluster=T25 {"AlliGator Q Event"=enum."GUI:Type of Displayed Image Changed", "Data"=variant} ("array"), "Data"=w494) -> (w495:T25)
            n236 = Build Array (concatenate)(w495, T25[] [{"AlliGator Q Event"=enum."Image:Image Histogram", "Data"=variant}, {"AlliGator Q Event"=enum."Image:Image Contrast", "Data"=variant}] ("element")) -> (w493:T25[])
          }
        }
      }
      event "Gate Image Slide": Value Change {
        n237 = event-data() -> ("CtlRef"=w504:refnum<vi>, "OldVal"=w503:u16, "NewVal"=w506:u16)  [unwired: 1 in]
        n238 = case shown="False" w505 {
          tunnel: w506 -> [_ w510]
          tunnel: w504 -> [w508 _]
          tunnel: w503 -> [w507 _]
          tunnel: [_ w509] -> w498
          frame False {
            n239 = property class="Slide (strict)"(reference=w508, "Value"=w507) -> ()  [unwired: 1 in, 2 out]
          }
          frame True {
            n240 = Bundle By Name(cluster=T25 {"AlliGator Q Event"=enum."GUI:Gate Image Slide Changed", "Data"=variant} ("element"), "Data"=w510) -> (w511:T25)
            n241 = Build Array(w511, T25 {"AlliGator Q Event"=enum."Image:Image Histogram", "Data"=variant} ("element"), T25 {"AlliGator Q Event"=enum."Image:Image Contrast", "Data"=variant} ("element")) -> (w509:T25[])
          }
        }
      }
      event "Highlight Image ROI": Value Change {
        n242 = event-data() -> ()  [unwired: 1 in, 1 out]
        n243 = case shown="True" w520 {
          tunnel: [_ T25[] [{"AlliGator Q Event"=enum."Phasor Plot:Highlight Image ROI in Phasor Plot", "Data"=variant}] ("element")] -> w515
          frame False {
          }
          frame True {
          }
        }
      }
      event "Highlight Phasor in Source Image": Value Change {
        n244 = event-data() -> ()  [unwired: 1 in, 1 out]
        n245 = case shown="True" w527 {
          tunnel: [_ T25[] [{"AlliGator Q Event"=enum."Phasor Plot:Overlay Phasor ROI, Ratio or Map in Source Image", "Data"=variant}] ("element")] -> w522
          frame False {
          }
          frame True {
          }
        }
      }
      event "Image Color Scale": Mouse Up {
        n246 = event-data() -> ()  [unwired: 1 in, 1 out]
        n247 = case shown="True" w534 {
          tunnel: [_ T25[] [{"AlliGator Q Event"=enum."Image:Image Contrast", "Data"=variant}] ("element")] -> w529
          frame False {
          }
          frame True {
          }
        }
      }
      event "Image Histogram Active": Value Change {
        n248 = event-data() -> ("NewVal"=w544:bool)  [unwired: 1 in]
        n249 = call "AlliGator Settings Storage.vi"("Get(F)/Set"=TRUE, "AlliGator Settings List"=AlliGator_Settings_List."Source Image:Image Histogram Active", "Variant Data in"=w544) -> ("Error Out"=w537:errorcluster)  [unwired: 7 in, 1 out]
      }
      event Value Change {
        n250 = event-data() -> ()  [unwired: 1 in, 1 out]
        n251 = case shown="True" w550 {
          tunnel: [_ w551] -> w545
          frame False {
          }
          frame True {
            n252 = Build Array(T25 {"AlliGator Q Event"=enum."Image:Image Histogram", "Data"=variant} ("element")) -> (w551:T25[])
          }
        }
      }
      event "Histogram Upper Percentile", "Histogram Lower Percentile": Value Change {
        # "This is not part of the Settings Window and needs to be handled separately"
        n253 = event-data() -> ("CtlRef"=w556:refnum<vi>, "NewVal"=w554:dbl)  [unwired: 1 in]
        n254 = property class="DigNum (strict)"(reference=w556) -> ("Label.Text"=w555:string)  [unwired: 1 in, 2 out]
        n255 = case shown="\"Histogram Upper Percentile\"" w555 {
          tunnel: [_ w563 w567] -> w557
          tunnel: w554 -> [_ w562 w566]
          frame "", Default {
          }
          frame "Histogram Lower Percentile" {
            n256 = local write "Lower Percentile"(w562) -> ()
            n257 = call "AlliGator Settings Storage.vi"("Get(F)/Set"=TRUE, "AlliGator Settings List"=AlliGator_Settings_List."Source Image:Histogram Lower Percentile", "Variant Data in"=w562) -> ("Error Out"=w563:errorcluster)  [unwired: 7 in, 1 out]
          }
          frame "Histogram Upper Percentile" {
            n258 = local write "Upper Percentile"(w566) -> ()
            n259 = call "AlliGator Settings Storage.vi"("Get(F)/Set"=TRUE, "AlliGator Settings List"=AlliGator_Settings_List."Source Image:Histogram Upper Percentile", "Variant Data in"=w566) -> ("Error Out"=w567:errorcluster)  [unwired: 7 in, 1 out]
          }
        }
      }
      event "Image Histogram": Cursor Move {
        w578 = T25 {"AlliGator Q Event"=enum."Image:Image Histogram Cursor Move", "Data"=variant} ("Time-Gated Phasor Q Element")
        n260 = event-data() -> ("Time"=w575:u32)  [unwired: 1 in]
        n261 = Unbundle By Name(w578) -> ("AlliGator Q Event"=w581:T24)
        n262 = property on="Auto-Adjust Contrast" class="Bool (strict)"() -> ("Value"=w570:bool)  [unwired: 2 in, 2 out]
        n263 = Bundle By Name(cluster=T39 {"AlliGator Q Event"=enum."---- Files ----", "Time"=0, "Timeout"=0} ("output cluster"), "AlliGator Q Event"=w581, "Time"=w575, "Timeout"=w576) -> (w579:T39)
        n264 = case shown="True" w570 {
          frame False {
          }
          frame True {
            n265 = property on="Auto-Adjust Contrast" class="Bool (strict)"("Val(Sgnl)"=FALSE ("Auto-Adjust Contrast")) -> ()  [unwired: 2 in, 2 out]
          }
        }
        n266 = call "AlliGator Filter Event.vi"("Filtered Event Data"=w579) -> ("Filter Event?"=w572:bool)  [unwired: 9 in, 1 out]
        n267 = call "AlliGator Image Contrast Status.vi"("Read/Write"=Read-Write."Read") -> ("Flag (out)"=w571:bool)  [unwired: 8 in]
        n268 = Or(x=w572, y=w571) -> (x .or. y?=w573:bool)
        n269 = case shown="False" w573 {
          tunnel: w578 -> [w590 _]
          tunnel: [w589 _] -> w577
          frame False {
            # "event not filtered out"
            n270 = call "AlliGator Image Contrast Status.vi"("Flag (in)"=TRUE, "Read/Write"=Read-Write."Write") -> ()  [unwired: 7 in, 1 out]
            n271 = Build Array(w590) -> (w589:T25[])
          }
          frame True {
          }
        }
      }
      event "Intensity Correction File": Value Change {
        n272 = event-data() -> ("NewVal"=w601:path, "CtlRef"=w599:refnum<vi>)  [unwired: 1 in]
        n273 = case shown="True" w598 {
          tunnel: w601 -> [_ w604]
          tunnel: w600 -> [_ w609]
          tunnel: w599 -> [_ w607]
          tunnel: [_ w605] -> w593
          tunnel: [_ w603] -> w592
          tunnel: [_ w602] -> w591
          frame False {
          }
          frame True {
            n274 = property class="Path"(reference=w607) -> (reference out=w610:refnum<vi>, error out=w608:errorcluster, "Label.Text"=w611:string)  [unwired: 1 in]
            n275 = Empty String/Path?(string/path=w604) -> (empty?=w612:bool)
            n276 = case shown="False" w612 {
              selector: w612 -> [_ w618]
              tunnel: w604 -> [w614 _]
              tunnel: [w613 _] -> w603
              frame False {
                n277 = Bundle By Name(cluster=T25 {"AlliGator Q Event"=enum."Intensity Time Trace:Load Intensity Corrections File", "Data"=variant} ("Time-Gated Phasor Q Element"), "Data"=w614) -> (w615:T25)
                n278 = Build Array(w615) -> (w613:T25[])
              }
              frame True {
                n279 = Not(x=w618) -> (.not. x?=w617:bool)
                n280 = property on="Use Intensity Correction File" class="Bool (strict)"("Val(Sgnl)"=w617) -> ()  [unwired: 2 in, 2 out]
              }
            }
            n281 = call "AlliGator Get Control Notebook String.vi"("error in (no error)"=w608, "Value"=w604, "Control Label"=w611) -> ("error out"=w606:errorcluster, "Notebook String"=w602:string)  [unwired: 7 in]
            n282 = call "AlliGator Update Settings & Control.vi"("Error In"=w606, "Value"=w604, "Sender"=w609, "CtlRef"=w610) -> ("Error Out"=w605:errorcluster)  [unwired: 7 in]
          }
        }
      }
      event "Lifetime & Other Parameters Graph", "Phasor Ratio Graph", "Decay Graph", "Phasor Graph", "Decay Statistics Graph", "Intensity Time Trace", "Image Histogram": Shortcut Menu Activation? {
        # "Shortcut Menu Activation"
        n283 = event-data() -> ("CtlRef"=w634:refnum<vi>, "MenuRef"=w633:refnum<k9>)  [unwired: 1 in]
        n284 = call "XY Graph Check-Uncheck Menu Items.vi"("Menu in"=w633, "XY Graph Refnum"=w634) -> ("Error Out (dup)"=w628:errorcluster, "Menu out"=w622:refnum<k9>, "XY Graph Refnum dup"=w620:T41)  [unwired: 6 in, 1 out]
        n285 = call "XY Graph Get Label.vi"("XYGraph"=w620) -> ("Graph Label"=w619:string)  [unwired: 8 in]
        n286 = case shown="\"Decay Graph\"" w619 {
          tunnel: w628 -> [w635 w641]
          tunnel: [w635 w640] -> w623
          tunnel: w622 -> [w636 w639]
          tunnel: [w636 w638] -> w621
          frame "", Default {
          }
          frame "Decay Graph" {
            n287 = call "AlliGator Decay Graph Get-Set Process Plot Target.vi"("Get (F)/Set"=FALSE, "Error In"=w641, "Menu"=w639) -> ("Error Out (dup)"=w640:errorcluster, "Menu"=w638:refnum<k9>)  [unwired: 6 in, 1 out]
          }
        }
        n288 = call "AlliGator Add Python Functions to Object Menu.vi"("error in (no error)"=w623, "Menu in"=w621, "Object Refnum"=w620) -> ("error out"=w627:errorcluster, "Menu out"=w625:refnum<k9>, "Object Refnum dup"=w624:refnum<vi>)  [unwired: 6 in]
        n289 = call "AlliGator Grayed out Menu Items.vi"("error in (no error)"=w627, "Menu in"=w625, "Object Refnum"=w624) -> ("error out"=w626:errorcluster)  [unwired: 7 in, 1 out]
        n290 = event-data() -> ()  [unwired: 2 in, 1 out]
      }
      event "Overlay Decay Fit Parameter Map": Value Change {
        n291 = event-data() -> ()  [unwired: 1 in, 1 out]
        n292 = case shown="True" w647 {
          tunnel: [_ T25[] [{"AlliGator Q Event"=enum."Decay Fit Parameter Map:Overlay Decay Fit Parameter Map in Source Image", "Data"=variant}] ("element")] -> w642
          frame False {
          }
          frame True {
          }
        }
      }
      event "Phasor Frame Slide": Value Change {
        n293 = event-data() -> ("CtlRef"=w655:refnum<vi>, "OldVal"=w654:i32, "NewVal"=w657:i32)  [unwired: 1 in]
        n294 = case shown="True" w656 {
          tunnel: w657 -> [_ w661]
          tunnel: w655 -> [w659 _]
          tunnel: w654 -> [w658 _]
          tunnel: [_ w660] -> w649
          frame False {
            n295 = property class="Slide (strict)"(reference=w659, "Value"=w658) -> ()  [unwired: 1 in, 2 out]
          }
          frame True {
            n296 = Bundle By Name(cluster=T25 {"AlliGator Q Event"=enum."Phasor Graph:Show Single Phasor", "Data"=variant} ("element"), "Data"=w661) -> (w662:T25)
            n297 = Build Array(w662) -> (w660:T25[])
          }
        }
      }
      event "Phasor Graph Active": Value Change {
        n298 = event-data() -> ("NewVal"=w671:bool)  [unwired: 1 in]
        n299 = call "AlliGator Settings Storage.vi"("Get(F)/Set"=TRUE, "AlliGator Settings List"=AlliGator_Settings_List."Phasor Graph:Phasor Graph Active", "Variant Data in"=w671) -> ("Error Out"=w664:errorcluster)  [unwired: 7 in, 1 out]
      }
      event "Phasor Graph Frequency", "Calibration Lifetime", "Save Phasor Plot", "Save Phasor Graph Image", "Phasor Plot Frequency", "Save Source Image", "Use Image Histogram for Contrast": Value Change {
        # "Each new control duplicated in the Settings Window needs to be added to this case\nunless it has its own event case\nThe labels of the controls need to be identical (in the Main AlliGator window and in the Settings window)"
        n300 = event-data() -> ("CtlRef"=w686:refnum<vi>)  [unwired: 1 in]
        n301 = property class="Ctl"(reference=w686) -> (reference out=w673:refnum<vi>, error out=w685:errorcluster, "Label.Text"=w672:string, "Value"=w680:variant)  [unwired: 1 in]
        n302 = case shown="\"Phasor Graph Frequency\"" w672 {
          tunnel: w685 -> [w687 w688 w690 w704 w725]
          tunnel: [w687 w688 w691 w708 w728] -> w684
          tunnel: [_ T25[] [{"AlliGator Q Event"=enum."Image:Image Histogram", "Data"=variant}, {"AlliGator Q Event"=enum."Image:Image Contrast", "Data"=variant}] ("AlliGator Actions") _ T25[] [{"AlliGator Q Event"=enum."Phasor Graph:Update SEPL Plot", "Data"=variant}] ("element") T25[] [{"AlliGator Q Event"=enum."Phasor Graph:Update SEPL Plot", "Data"=variant}] ("element")] -> w676
          tunnel: w681 -> [_ _ _ w711 w730]
          tunnel: w680 -> [_ _ _ w706 w726]
          frame "", Default {
            # "only updates the corresponding Settings window control"
          }
          frame "Use Image Histogram for Contrast" {
          }
          frame "Calibration Lifetime" {
            n303 = disable-structure shown="Disabled" {
              disable-tunnel: [w694 _] -> w691
              disable-tunnel: w690 -> [w693 _]
              frame Disabled {
                n304 = call "Alligator Variables Storage.vi"("AlliGator Variable"=AlliGator_Variables_List."Phasor Plot:Computed" ("Alligator Variable"), "Error In"=w693) -> ("Error Out"=w692:errorcluster, "Data out"=w696:variant)  [unwired: 7 in, 1 out]
                n305 = call-poly "Variant to Data.vi"("Variant"=w696) -> ("Value"=w695:bool)  [unwired: 8 in]
                n306 = case shown="True" w695 {
                  tunnel: w692 -> [w698 w701]
                  tunnel: [w698 w699] -> w694
                  frame False {
                  }
                  frame True {
                    n307 = call "AlliGator Set Phasor Plot Update LED.vi"("error in (no error)"=w701, "Off/On"=TRUE) -> ("error out"=w699:errorcluster)  [unwired: 9 in]
                  }
                }
              }
              frame Enabled {
              }
            }
          }
          frame "Phasor Plot Frequency" {
            # "Need to update TWO controls"
            n308 = Variant To Data(error in=w704, type=dbl[unit] 0.0 ("Calibration Phasor Frequency"), Variant=w706) -> (data=w702:dbl[unit], error out=w703:errorcluster)
            n309 = control-ref of="Phasor Graph Frequency"() -> (w710:refnum<vi>)
            n310 = call "Alligator Variables Storage.vi"("AlliGator Variable"=AlliGator_Variables_List."Phasor Plot:Computed" ("Alligator Variable"), "Error In"=w704) -> ("Error Out"=w709:errorcluster, "Data out"=w714:variant)  [unwired: 7 in, 1 out]
            n311 = local write "Phasor Graph Frequency"(w702) -> ()
            n312 = call "AlliGator Update Settings & Control.vi"("Error In"=w703, "Value"=w702, "Sender"=w711, "CtlRef"=w710) -> ("Error Out"=w707:errorcluster)  [unwired: 7 in]
            n313 = call-poly "Variant to Data.vi"("Variant"=w714) -> ("Value"=w713:bool)  [unwired: 8 in]
            n314 = case shown="True" w713 {
              tunnel: w709 -> [w717 w720]
              tunnel: [w717 w718] -> w716
              frame False {
              }
              frame True {
                n315 = call "AlliGator Set Phasor Plot Update LED.vi"("error in (no error)"=w720, "Off/On"=TRUE) -> ("error out"=w718:errorcluster)  [unwired: 9 in]
              }
            }
            n316 = Merge Errors(w716, w707) -> (w708:errorcluster)
          }
          frame "Phasor Graph Frequency" {
            # "Need to update TWO controls"
            n317 = control-ref of="Phasor Plot Frequency"() -> (w729:refnum<vi>)
            n318 = Variant To Data(error in=w725, type=dbl[unit] 0.0 ("Phasor Plot Frequency"), Variant=w726) -> (data=w721:dbl[unit], error out=w724:errorcluster)
            n319 = call "Alligator Variables Storage.vi"("AlliGator Variable"=AlliGator_Variables_List."Phasor Plot:Computed" ("Alligator Variable"), "Error In"=w725) -> ("Error Out"=w723:errorcluster, "Data out"=w733:variant)  [unwired: 7 in, 1 out]
            n320 = call-poly "Variant to Data.vi"("Variant"=w733) -> ("Value"=w732:bool)  [unwired: 8 in]
            n321 = local write "Phasor Plot Frequency"(w721) -> ()
            n322 = call "AlliGator Update Settings & Control.vi"("Error In"=w724, "Value"=w721, "Sender"=w730, "CtlRef"=w729) -> ("Error Out"=w727:errorcluster)  [unwired: 7 in]
            n323 = case shown="True" w732 {
              tunnel: w723 -> [w736 w739]
              tunnel: [w736 w737] -> w735
              frame False {
              }
              frame True {
                n324 = call "AlliGator Set Phasor Plot Update LED.vi"("error in (no error)"=w739, "Off/On"=TRUE) -> ("error out"=w737:errorcluster)  [unwired: 9 in]
              }
            }
            n325 = Merge Errors(w735, w727) -> (w728:errorcluster)
          }
        }
        n326 = call "AlliGator Update Settings & Control.vi"("Error In"=w684, "Value"=w680, "Sender"=w681, "CtlRef"=w673) -> ("Error Out"=w677:errorcluster)  [unwired: 7 in]
        n327 = call "AlliGator Get Control Notebook String.vi"("error in (no error)"=w677, "Value"=w680, "Control Label"=w672) -> ("error out"=w675:errorcluster, "Notebook String"=w674:string)  [unwired: 7 in]
      }
      event "Phasor Graph Frequency", "Phasor Plot Frequency": Shortcut Menu Selection (User) {
        n328 = event-data() -> ("CtlRef"=w746:refnum<vi>, "ItemTag"=w745:string)  [unwired: 1 in]
        n329 = case shown="\"f = 1/D\"" w745 {
          tunnel: w746 -> [_ w748 w751 w754 w758]
          tunnel: [_ w747 w749 w752 w755] -> w740
          frame "", Default {
          }
          frame "f = 1/T" {
            n330 = call "AlliGator Set Phasor Harmonic.vi"("Phasor Frequency Refnum"=w748) -> ("Error Out"=w747:errorcluster)  [unwired: 10 in]
          }
          frame "f = 1/D" {
            n331 = call "AlliGator Set Phasor Harmonic.vi"("Use n/D"=TRUE, "Phasor Frequency Refnum"=w751) -> ("Error Out"=w749:errorcluster)  [unwired: 9 in]
          }
          frame "f = n/T (n > 1)" {
            n332 = call "AlliGator Set Phasor Harmonic.vi"("Harmonic (1)"=0, "Phasor Frequency Refnum"=w754) -> ("Error Out"=w752:errorcluster)  [unwired: 9 in]
          }
          frame "f = n/D (n > 1)" {
            n333 = call "AlliGator Set Phasor Harmonic.vi"("Use n/D"=TRUE, "Harmonic (1)"=0, "Phasor Frequency Refnum"=w758) -> ("Error Out"=w755:errorcluster)  [unwired: 8 in]
          }
        }
      }
      event "Phasor Graph": Cursor Move {
        n334 = event-data() -> ("Time"=w760:u32)  [unwired: 1 in]
        n335 = case shown="True" w761 {
          tunnel: [_ w768] -> w762
          tunnel: w760 -> [_ w771]
          tunnel: w759 -> [_ w767]
          frame False {
          }
          frame True {
            w769 = T25 {"AlliGator Q Event"=enum."Phasor Graph:Cursor Move", "Data"=variant} ("Time-Gated Phasor Q Element")
            n336 = Unbundle By Name(w769) -> ("AlliGator Q Event"=w774:T24)
            n337 = Bundle By Name(cluster=T39 {"AlliGator Q Event"=enum."---- Files ----", "Time"=0, "Timeout"=0} ("output cluster"), "AlliGator Q Event"=w774, "Time"=w771, "Timeout"=w767) -> (w772:T39)
            n338 = call "AlliGator Filter Event.vi"("Filtered Event Data"=w772) -> ("Filter Event?"=w770:bool)  [unwired: 9 in, 1 out]
            n339 = case shown="False" w770 {
              tunnel: w769 -> [w776 _]
              tunnel: [w775 _] -> w768
              frame False {
                n340 = Build Array(w776) -> (w775:T25[])
              }
              frame True {
              }
            }
          }
        }
      }
      event "Phasor Graph": Scale Range Change; "Phasor Graph": Autoscale Range Change; "Phasor Graph": Cursor Release {
        n341 = event-data() -> ()  [unwired: 1 in, 1 out]
        n342 = case shown="True" w782 {
          tunnel: [_ T25[] [{"AlliGator Q Event"=enum."Phasor Graph:Draw Cursor Connecting Line", "Data"=variant}] ("element")] -> w777
          frame False {
          }
          frame True {
          }
        }
      }
      event "Phasor Graph": Shortcut Menu Selection (User) {
        n343 = event-data() -> ("CtlRef"=w795:refnum<vi>, "Coords"=w794:T35, "ItemTag"=w793:string, "ItemPath"=w792:string)  [unwired: 1 in]
        n344 = call-poly <vilib>:"Acquire Input Data.vi"("device ID"=w790, "error in (no error)"=w791) -> ("device ID"=w789:refnum<k1>, "keys pressed"=w787:T49, "error out"=w788:errorcluster)  [unwired: 15 in]
        n345 = case shown="True" w796 {
          tunnel: w795 -> [_ w811]
          tunnel: w794 -> [_ w810]
          tunnel: w793 -> [_ w809]
          tunnel: w792 -> [_ w808]
          tunnel: w787 -> [_ w804]
          tunnel: [_ w801] -> w786
          tunnel: [_ w800] -> w785
          tunnel: [_ w799] -> w784
          frame False {
          }
          frame True {
            n346 = Index Array(array=w804) -> (element=w803:T32)  [unwired: 1 in]
            n347 = Equal?(x=w803, y=T32."H" ("element")) -> (x = y?=w802:bool)
            n348 = Bundle By Name(cluster=T37 {"Item Tag"="", "XY Graph Refnum"=refnum, "Coords"={"Horizontal"=0, "Vertical"=0}, "Item Path"=""} ("XY Graph Event"), "XY Graph Refnum"=w811, "Coords"=w810, "Item Tag"=w809, "Item Path"=w808) -> (w807:T37)
            n349 = call "AlliGator Phasor Graph Context Menu Handler.vi"("Help?"=w802, "XY Graph Event"=w807) -> ("Error Out"=w800:errorcluster, "Message"=w801:string, "AlliGator Actions"=w799:T25[])  [unwired: 7 in]
          }
        }
      }
      event "Phasor Plot Active": Value Change {
        n350 = event-data() -> ("NewVal"=w819:bool)  [unwired: 1 in]
        n351 = call "AlliGator Settings Storage.vi"("Get(F)/Set"=TRUE, "AlliGator Settings List"=AlliGator_Settings_List."Phasor Plot:Phasor Plot Active", "Variant Data in"=w819) -> ("Error Out"=w812:errorcluster)  [unwired: 7 in, 1 out]
      }
      event "Phasor Plot Color Scale", "Decay Fit Parameter Map Color Scale", "Image Color Scale": Shortcut Menu Activation? {
        w826 = string[] ["Copy Color Scale to Clipboard"] ("item names")
        n352 = event-data() -> ("MenuRef"=w828:refnum<k9>)  [unwired: 1 in]
        n353 = Delete Menu Items(9:w828) -> (0:w821:errorcluster, 3:w827:refnum<k9>)  [unwired: 3 in]
        n354 = Insert Menu Items(6:w821, 7:w826, 8:w826, 9:w827) -> (0:w820:errorcluster)  [unwired: 2 in, 2 out]
        n355 = event-data() -> ()  [unwired: 2 in, 1 out]
      }
      event "Phasor Plot Color Scale", "Image Color Scale", "Decay Fit Parameter Map Color Scale": Shortcut Menu Selection (User) {
        n356 = event-data() -> ("CtlRef"=w833:refnum<vi>, "ItemTag"=w834:string)  [unwired: 1 in]
        n357 = case shown="\"Copy Color Scale to Clipboard\"" w834 {
          tunnel: w833 -> [_ w835]
          frame "", Default {
          }
          frame "Copy Color Scale to Clipboard" {
            n358 = call "Export Color Ramp to Clipboard.vi"("ColorRamp in"=w835) -> ()  [unwired: 11 in]
          }
        }
      }
      event "Phasor Plot Color Scale": Mouse Up {
        n359 = event-data() -> ()  [unwired: 1 in, 1 out]
        n360 = case shown="True" w841 {
          tunnel: [_ w842] -> w836
          frame False {
          }
          frame True {
            n361 = Bundle By Name(cluster=T25 {"AlliGator Q Event"=enum."Phasor Plot:Change Phasor Plot Color Palette", "Data"=variant} ("element"), "Data"="Refresh Image" ("String")) -> (w844:T25)
            n362 = Build Array(w844) -> (w842:T25[])
          }
        }
      }
      event "Phasor Plot Image": Shortcut Menu Activation? {
        w859 = AlliGator_Variables_List."Phasor Plot:Phasor Ratio Palette List" ("Alligator Variable")
        n363 = event-data() -> ("CtlRef"=w847:refnum<vi>, "MenuRef"=w873:refnum<k9>)  [unwired: 1 in]
        n364 = call "Alligator Variables Storage.vi"("Get(F)/Set"=FALSE, "AlliGator Variable"=AlliGator_Variables_List."Phasor Plot:Palette Information" ("Alligator Variable")) -> ("Error Out"=w869:errorcluster, "Data out"=w870:variant)  [unwired: 7 in, 1 out]
        n365 = call "Alligator Variables Storage.vi"("Get(F)/Set"=FALSE, "AlliGator Variable"=w859) -> ("Error Out"=w850:errorcluster, "Data out"=w863:variant)  [unwired: 7 in, 1 out]
        n366 = Variant To Data(error in=w869, type=T29 {"Palette Name [# Colors,int?,inv?]"="", "Palette Type"=0, "Palette Colors"=[], "Interpolate?"=FALSE} ("Image Display Palette Information"), Variant=w870) -> (data=w868:T29, error out=w867:errorcluster)
        n367 = call-poly "Variant to Data.vi"("Variant"=w863) -> ("String Array"=w862:string[])  [unwired: 8 in]
        n368 = Unbundle By Name(w868) -> ("Palette Name [# Colors,int?,inv?]"=w865:string)
        n369 = Merge Errors(w867, w850) -> (w851:errorcluster)
        n370 = call "Check Selected Palette in Menu.vi"("Error In"=w851, "Palette List"=w862, "Checked Palette"=w865, "Menu in"=w873) -> ("Error Out"=w858:errorcluster, "Stored Palette List"=w860:string[], "menu reference out"=w857:refnum<k9>)  [unwired: 5 in]
        n371 = call "Alligator Variables Storage.vi"("Get(F)/Set"=TRUE, "AlliGator Variable"=w859, "Error In"=w858, "Data in"=w860) -> ("Error Out"=w856:errorcluster)  [unwired: 5 in, 2 out]
        n372 = call "AlliGator Show-Hide Phasor Plot Menu Items.vi"("error in (no error)"=w856, "Menu in"=w857) -> ("error out"=w849:errorcluster, "Menu out"=w846:refnum<k9>)  [unwired: 8 in]
        n373 = call "AlliGator Add Python Functions to Object Menu.vi"("error in (no error)"=w849, "Menu in"=w846, "Object Refnum"=w847) -> ("error out"=w848:errorcluster)  [unwired: 6 in, 2 out]
        n374 = event-data() -> ()  [unwired: 2 in, 1 out]
      }
      event "Phasor Plot Image": Shortcut Menu Selection (User) {
        n375 = event-data() -> ("CtlRef"=w886:refnum<vi>, "ItemTag"=w883:string, "ItemPath"=w887:string, "Coords"=w888:T35)  [unwired: 1 in]
        n376 = call-poly <vilib>:"Acquire Input Data.vi"("device ID"=w879, "error in (no error)"=w880) -> ("device ID"=w878:refnum<k1>, "keys pressed"=w877:T49, "error out"=w876:errorcluster)  [unwired: 15 in]
        n377 = case shown="True" w882 {
          tunnel: w888 -> [_ w899]
          tunnel: w887 -> [_ w898]
          tunnel: w886 -> [_ w897]
          tunnel: w883 -> [_ w896]
          tunnel: [_ w895] -> w881
          tunnel: w877 -> [_ w891]
          tunnel: [_ w890] -> w875
          tunnel: [_ w889] -> w874
          frame False {
          }
          frame True {
            n378 = Index Array(array=w891) -> (element=w894:T32)  [unwired: 1 in]
            n379 = Equal?(x=w894, y=T32."H" ("element")) -> (x = y?=w892:bool)
            n380 = case shown="False" w892 {
              tunnel: w899 -> [w908 _]
              tunnel: w898 -> [w907 _]
              tunnel: w897 -> [w906 w912]
              tunnel: w896 -> [w905 w911]
              tunnel: [w904 _] -> w895
              tunnel: [w901 w910] -> w890
              tunnel: [w900 w909] -> w889
              frame False {
                n381 = Bundle By Name(cluster=T33 {"Item Tag"="", "Image Control Refnum"=refnum, "Coords"={"Horizontal"=0, "Vertical"=0}, "Item Path"=""} ("Image Event Data"), "Image Control Refnum"=w906, "Item Tag"=w905, "Item Path"=w907, "Coords"=w908) -> (w902:T33)
                n382 = call "AlliGator Phasor Plot Context Menu Handler.vi"("Image Event"=w902) -> ("Error Out"=w900:errorcluster, "Message"=w901:string, "AlliGator Actions"=w904:T25[])  [unwired: 8 in]
              }
              frame True {
                n383 = property class="ImageControl"(reference=w912) -> ("Label.Text"=w913:string)  [unwired: 1 in, 2 out]
                n384 = call "AlliGator Send Python Function Doc String to Notebook.vi"("Item Tag"=w911, "Target"=w913) -> ("Error Out"=w909:errorcluster, "Message"=w910:string)  [unwired: 8 in]
              }
            }
          }
        }
      }
      event "Phasor Plot ROI Color": Value Change {
        n385 = event-data() -> ("NewVal"=w914:u32)  [unwired: 1 in]
        n386 = call <vilib>:"Color to RGB.vi"("Color"=w914) -> ("R"=w917:u8, "G"=w918:u8, "B"=w919:u8)  [unwired: 1 out]
        n387 = Bundle By Name(cluster=cluster{"Red":u8, "Green":u8, "Blue":u8} {"Red"=0, "Green"=0, "Blue"=0} ("ROI Color"), "Red"=w917, "Green"=w918, "Blue"=w919) -> (w916:cluster{"Red":u8, "Green":u8, "Blue":u8})
        n388 = property on="Phasor Plot Image" class="ImageControl"("ROI Color"=w916) -> ()  [unwired: 2 in, 2 out]
      }
      event "Phasor Ratio Graph", "Decay Graph", "Phasor Graph", "Lifetime & Other Parameters Graph", "Decay Statistics Graph": event #0x4e {
        # "Change style of new cursor to a more visible one"
        n389 = event-data() -> ("ItemTag"=w926:string, "CtlRef"=w925:refnum<vi>)  [unwired: 1 in]
        n390 = case shown="\"CURS_FREE\", \"CURS_MULTI\", \"CURS_SINGLE\"" w926 {
          tunnel: w925 -> [_ w931]
          tunnel: [_ w933] -> w924
          frame "", Default {
          }
          frame "CURS_FREE", "CURS_MULTI", "CURS_SINGLE" {
            n391 = Bundle By Name(cluster=T25 {"AlliGator Q Event"=enum."Generic Graph:Set Last Cursor Style", "Data"=variant} ("AlliGator Actions"), "Data"=w931) -> (w932:T25)
            n392 = Build Array(w932) -> (w933:T25[])
          }
        }
      }
      event "Phasor Ratio Graph", "Lifetime & Other Parameters Graph": Shortcut Menu Selection (User) {
        n393 = event-data() -> ("ItemPath"=w936:string, "CtlRef"=w946:refnum<vi>, "Coords"=w945:T35, "ItemTag"=w937:string)  [unwired: 1 in]
        n394 = Select(t=w937, s=w944, f=w942) -> (s? t:f=w943:string)
        n395 = case shown="\"Linear Fit\"" w943 {
          selector: w943 -> [_ w949 _ _ _ _]
          tunnel: w946 -> [_ w951 _ _ w970 _]
          tunnel: w945 -> [_ w950 _ _ w969 _]
          tunnel: w936 -> [_ w948 _ _ _ _]
          tunnel: [_ w947 _ w957 w968 w974] -> w935
          frame "", "Busy" {
          }
          frame Default {
            n396 = Bundle By Name(cluster=T37 {"Item Tag"="", "XY Graph Refnum"=refnum, "Coords"={"Horizontal"=0, "Vertical"=0}, "Item Path"=""} ("XY Graph Event"), "Item Path"=w948, "XY Graph Refnum"=w951, "Coords"=w950, "Item Tag"=w949) -> (w954:T37)
            n397 = Bundle By Name(cluster=T25 {"AlliGator Q Event"=enum."Generic Graph:Generic XY Graph Event", "Data"=variant} ("element"), "Data"=w954) -> (w952:T25)
            n398 = Build Array(w952) -> (w947:T25[])
          }
          frame "-----------------" {
          }
          frame "New Plot" {
            w956 = T50 {"Multiplot XY Graph"=refnum, "Plot Name"="", "Plot Scales"={"X Scale"=0, "Y Scale"=0}, "Plot Interpolation"=7, "Point Style"=enum."not defined", "Plot Color"=15781887, "Plot Metadata"=variant} ("New Plot Information")
            w961 = T25 {"AlliGator Q Event"=enum."Generic Graph:New Plot", "Data"=variant} ("Time-Gated Phasor Q Element")
            n399 = control-ref of="Lifetime & Other Parameters Graph"() -> (w958:refnum<vi>)
            n400 = control-ref of="Phasor Ratio Graph"() -> (w959:refnum<vi>)
            n401 = Bundle By Name(cluster=w956, "Multiplot XY Graph"=w959, "Plot Name"="Phasor Ratio") -> (w965:T50)
            n402 = Bundle By Name(cluster=w956, "Multiplot XY Graph"=w958, "Plot Name"="Lifetime") -> (w962:T50)
            n403 = Bundle By Name(cluster=w961, "Data"=w965) -> (w966:T25)
            n404 = Bundle By Name(cluster=w961, "Data"=w962) -> (w960:T25)
            n405 = Build Array(w966, w960) -> (w957:T25[])
          }
          frame "Linear Fit" {
            n406 = Bundle(cluster=T40 {"Multiplot XY Graph"=refnum, "Mouse Coordinates"={"Horizontal"=0, "Vertical"=0}} ("Mouse Click Event Data"), "Multiplot XY Graph"=w970, "Mouse Coordinates"=w969) -> (w972:T40)
            n407 = Bundle By Name(cluster=T25 {"AlliGator Q Event"=enum."Phasor Ratio:Fit Line to Phasor Ratio Plot", "Data"=variant} ("Time-Gated Phasor Q Element"), "Data"=w972) -> (w973:T25)
            n408 = Build Array(w973) -> (w968:T25[])
          }
          frame "Plot Decay Shifts" {
            n409 = Build Array(T25 {"AlliGator Q Event"=enum."Decay:Plot Decay Shifts", "Data"=variant} ("element")) -> (w974:T25[])
          }
        }
      }
      event "Phasor Reference 1 Control": Value Change {
        n410 = event-data() -> ("CtlRef"=w982:refnum<vi>, "OldVal"=w981:dbl, "NewVal"=w984:dbl)  [unwired: 1 in]
        n411 = case shown="True" w983 {
          tunnel: w985 -> [_ _]
          tunnel: w984 -> [_ w990]
          tunnel: w982 -> [w987 _]
          tunnel: w981 -> [w986 _]
          tunnel: [_ w988] -> w976
          frame False {
            n412 = property class="Scroll (strict)"(reference=w987, "Value"=w986) -> ()  [unwired: 1 in, 2 out]
          }
          frame True {
            n413 = Bundle By Name(cluster=T25 {"AlliGator Q Event"=enum."Phasor Ratio:Update Phasor Reference 1", "Data"=variant} ("Time-Gated Phasor Q Element"), "Data"=w990) -> (w991:T25)
            n414 = Build Array(w991, T25 {"AlliGator Q Event"=enum."Phasor Graph:Draw Cursor Connecting Line", "Data"=variant} ("Time-Gated Phasor Q Element")) -> (w988:T25[])
          }
        }
      }
      event "Phasor Reference 2 Control": Value Change {
        n415 = event-data() -> ("CtlRef"=w999:refnum<vi>, "OldVal"=w998:dbl, "NewVal"=w1001:dbl)  [unwired: 1 in]
        n416 = case shown="True" w1000 {
          tunnel: w1002 -> [_ _]
          tunnel: w1001 -> [_ w1007]
          tunnel: w999 -> [w1004 _]
          tunnel: w998 -> [w1003 _]
          tunnel: [_ w1005] -> w993
          frame False {
            n417 = property class="Scroll (strict)"(reference=w1004, "Value"=w1003) -> ()  [unwired: 1 in, 2 out]
          }
          frame True {
            n418 = Bundle By Name(cluster=T25 {"AlliGator Q Event"=enum."Phasor Ratio:Update Phasor Reference 2", "Data"=variant} ("Time-Gated Phasor Q Element"), "Data"=w1007) -> (w1008:T25)
            n419 = Build Array(w1008, T25 {"AlliGator Q Event"=enum."Phasor Graph:Draw Cursor Connecting Line", "Data"=variant} ("Time-Gated Phasor Q Element")) -> (w1005:T25[])
          }
        }
      }
      event "Refresh Image": Value Change {
        n420 = event-data() -> ()  [unwired: 1 in, 1 out]
        n421 = case shown="True" w1015 {
          tunnel: w1016 -> [_ _]
          tunnel: [_ w1017] -> w1010
          frame False {
          }
          frame True {
            n422 = Build Array(T25 {"AlliGator Q Event"=enum."Files:New Folder Selected", "Data"=variant} ("Time-Gated Phasor Q Element")) -> (w1017:T25[])
          }
        }
      }
      event "Refresh Decay Fit Parameter Map": Value Change {
        n423 = event-data() -> ()  [unwired: 1 in, 1 out]
        n424 = case shown="True" w1024 {
          tunnel: w1025 -> [_ _]
          tunnel: [_ w1026] -> w1019
          frame False {
          }
          frame True {
            w1029 = TRUE  # Parameter changed
            n425 = local read "Decay Fit Parameter"() -> (w1028:T11)
            n426 = Bundle(cluster=T36 {"Parameter"=enum."Offset", "Parameter changed"=FALSE} ("output cluster"), "Parameter"=w1028, "Parameter changed"=w1029) -> (w1027:T36)
            n427 = Bundle By Name(cluster=T25 {"AlliGator Q Event"=enum."Decay Fit Parameter Map:Build Decay Fit Parameter Map", "Data"=variant} ("Time-Gated Phasor Q Element"), "Data"=w1027) -> (w1031:T25)
            n428 = Build Array(w1031) -> (w1026:T25[])
          }
        }
      }
      event "Refresh Phasor Plot": Shortcut Menu Activation? {
        n429 = event-data() -> ("MenuRef"=w1038:refnum<k9>)  [unwired: 1 in]
        n430 = call "AlliGator Set Checks in Phasor Update Button.vi"("Menu in"=w1038) -> ("Error Out"=w1033:errorcluster)  [unwired: 10 in]
        n431 = event-data() -> ()  [unwired: 2 in, 1 out]
      }
      event "Refresh Phasor Plot": Shortcut Menu Selection (User) {
        n432 = event-data() -> ("ItemTag"=w1045:string, "CtlRef"=w1039:refnum<vi>)  [unwired: 1 in]
        n433 = call "AlliGator Update Phasor Image Elements to Update.vi"("CtlRef"=w1039, "Phasor Plot Element to Update"=w1045) -> ("Error Out"=w1040:errorcluster)  [unwired: 8 in, 1 out]
      }
      event "Refresh Phasor Plot": Value Change {
        n434 = event-data() -> ()  [unwired: 1 in, 1 out]
        n435 = case shown="True" w1051 {
          tunnel: [_ w1052] -> w1046
          frame False {
          }
          frame True {
            n436 = Build Array(T25 {"AlliGator Q Event"=enum."Phasor Plot:Build Phasor Plot", "Data"=variant} ("Time-Gated Phasor Q Element")) -> (w1052:T25[])
          }
        }
      }
      event "Refresh SEPL": Value Change {
        n437 = event-data() -> ()  [unwired: 1 in, 1 out]
        n438 = case shown="True" w1059 {
          tunnel: [_ w1060] -> w1054
          frame False {
          }
          frame True {
            n439 = Build Array(T25 {"AlliGator Q Event"=enum."Phasor Graph:Update SEPL Plot", "Data"=variant} ("element")) -> (w1060:T25[])
          }
        }
      }
      event "Scale Bar": Value Change {
        n440 = event-data() -> ()  [unwired: 1 in, 1 out]
        n441 = case shown="True" w1067 {
          tunnel: [_ w1068] -> w1062
          frame False {
          }
          frame True {
            n442 = Build Array(T25 {"AlliGator Q Event"=enum."Image:Add Scale Bar Overlay", "Data"=variant} ("element")) -> (w1068:T25[])
          }
        }
      }
      event "Show Line": Value Change {
        n443 = event-data() -> ("CtlRef"=w1080:refnum<vi>, "NewVal"=w1078:bool, "OldVal"=w1076:bool)  [unwired: 1 in]
        n444 = case shown="True" w1077 {
          tunnel: w1080 -> [w1083 _]
          tunnel: w1079 -> [_ _]
          tunnel: w1078 -> [_ w1086]
          tunnel: w1076 -> [w1082 _]
          tunnel: [w1081 w1085] -> w1071
          tunnel: [_ w1087] -> w1070
          frame False {
            n445 = property class="Bool (strict)"(reference=w1083, "Value"=w1082) -> (error out=w1081:errorcluster)  [unwired: 1 in, 1 out]
          }
          frame True {
            n446 = call "Alligator Variables Storage.vi"("AlliGator Variable"=AlliGator_Variables_List."Phasor Graph:Show Line", "Data in"=w1086) -> ("Error Out"=w1085:errorcluster)  [unwired: 7 in, 2 out]
            n447 = Build Array(T25 {"AlliGator Q Event"=enum."Phasor Graph:Draw Cursor Connecting Line", "Data"=variant} ("Time-Gated Phasor Q Element"), T25 {"AlliGator Q Event"=enum."Phasor Graph:Find UC Intersection", "Data"=variant} ("Time-Gated Phasor Q Element")) -> (w1089:T25[])
            n448 = Select(t=w1089, s=w1086, f=T25[] [{"AlliGator Q Event"=enum."Phasor Graph:Clear Cursor Connecting Line", "Data"=variant}] ("element")) -> (s? t:f=w1087:T25[])
          }
        }
      }
      event "Single Step Phasor": Value Change {
        n449 = event-data() -> ("CtlRef"=w1098:refnum<vi>, "NewVal"=w1100:bool, "OldVal"=w1097:bool)  [unwired: 1 in]
        n450 = case shown="True" w1099 {
          tunnel: w1100 -> [_ w1108]
          tunnel: w1098 -> [w1102 _]
          tunnel: w1097 -> [w1101 _]
          tunnel: [_ w1103] -> w1092
          frame False {
            n451 = property class="Bool (strict)"(reference=w1102, "Value"=w1101) -> ()  [unwired: 1 in, 2 out]
          }
          frame True {
            n452 = property on="Phasor Frame Slide" class="Slide (strict)"("Visible"=w1108) -> ("Value"=w1107:i32)  [unwired: 2 in, 2 out]
            n453 = Select(t=w1107, s=w1108, f=0) -> (s? t:f=w1105:i32)
            n454 = Decrement(x=w1105) -> (x-1=w1104:i32)
            n455 = Bundle By Name(cluster=T25 {"AlliGator Q Event"=enum."Phasor Graph:Show Single Phasor", "Data"=variant} ("element"), "Data"=w1104) -> (w1109:T25)
            n456 = Build Array(w1109) -> (w1103:T25[])
          }
        }
      }
      event "Source Image ROI Color": Value Change {
        n457 = event-data() -> ("NewVal"=w1111:u32)  [unwired: 1 in]
        n458 = call <vilib>:"Color to RGB.vi"("Color"=w1111) -> ("R"=w1114:u8, "G"=w1115:u8, "B"=w1116:u8)  [unwired: 1 out]
        n459 = Bundle By Name(cluster=cluster{"Red":u8, "Green":u8, "Blue":u8} {"Red"=0, "Green"=0, "Blue"=0} ("ROI Color"), "Red"=w1114, "Green"=w1115, "Blue"=w1116) -> (w1113:cluster{"Red":u8, "Green":u8, "Blue":u8})
        n460 = property on="Source Image" class="ImageControl"("ROI Color"=w1113) -> ()  [unwired: 2 in, 2 out]
      }
      event "Source Image ROI Selection": Value Change {
        n461 = event-data() -> ("CtlRef"=w1127:refnum<vi>, "OldVal"=w1126:i32, "NewVal"=w1130:i32)  [unwired: 1 in]
        n462 = Subtract(x=w1126, y=w1130) -> (x-y=w1129:i32)
        n463 = case shown="True" w1128 {
          tunnel: w1129 -> [_ w1134]
          tunnel: w1127 -> [w1132 _]
          tunnel: w1126 -> [w1131 _]
          tunnel: [_ w1133] -> w1121
          frame False {
            n464 = property class="Scroll (strict)"(reference=w1132, "Value"=w1131) -> ()  [unwired: 1 in, 2 out]
          }
          frame True {
            n465 = case shown="..-1" w1134 {
              tunnel: [_ w1135 w1141] -> w1133
              frame 0, Default {
              }
              frame 1.. {
                n466 = Bundle("Action"=AlliGator_ROI_Manager_Actions."Select Previous ROI", -1) -> (w1137:cluster{"Action":T42, i32})  [unwired: 1 in]
                n467 = Bundle By Name(cluster=T25 {"AlliGator Q Event"=enum."Image:Source Image ROI Selection", "Data"=variant} ("Time-Gated Phasor Q Element"), "Data"=w1137) -> (w1139:T25)
                n468 = Build Array(w1139) -> (w1135:T25[])
              }
              frame ..-1 {
                n469 = Bundle("Action"=AlliGator_ROI_Manager_Actions."Select Next ROI", -1) -> (w1143:cluster{"Action":T42, i32})  [unwired: 1 in]
                n470 = Bundle By Name(cluster=T25 {"AlliGator Q Event"=enum."Image:Source Image ROI Selection", "Data"=variant} ("Time-Gated Phasor Q Element"), "Data"=w1143) -> (w1145:T25)
                n471 = Build Array(w1145) -> (w1141:T25[])
              }
            }
          }
        }
      }
      event "Source Image", "Phasor Plot Image", "Decay Fit Parameter Map Image": Mouse Wheel {
        n472 = event-data() -> ("CtlRef"=w1152:refnum<vi>, "Delta"=w1151:i32)  [unwired: 1 in]
        n473 = call "Image Display Mouse Wheel Zoom.vi"("Mouse Wheel Delta"=w1151, "Image Control Refnum"=w1152) -> ()  [unwired: 9 in, 1 out]
      }
      event "Source Image": Shortcut Menu Activation? {
        w1164 = AlliGator_Variables_List."Source Image:Palette List" ("Alligator Variable")
        n474 = event-data() -> ("CtlRef"=w1155:refnum<vi>, "MenuRef"=w1178:refnum<k9>)  [unwired: 1 in]
        n475 = call "Alligator Variables Storage.vi"("Get(F)/Set"=FALSE, "AlliGator Variable"=AlliGator_Variables_List."X_Source Image Palette Information" ("Alligator Variable")) -> ("Error Out"=w1174:errorcluster, "Data out"=w1175:variant)  [unwired: 7 in, 1 out]
        n476 = call "Alligator Variables Storage.vi"("Get(F)/Set"=FALSE, "AlliGator Variable"=w1164) -> ("Error Out"=w1157:errorcluster, "Data out"=w1168:variant)  [unwired: 7 in, 1 out]
        n477 = Variant To Data(error in=w1174, type=T29 {"Palette Name [# Colors,int?,inv?]"="", "Palette Type"=0, "Palette Colors"=[], "Interpolate?"=FALSE} ("Image Display Palette Information"), Variant=w1175) -> (data=w1173:T29, error out=w1172:errorcluster)
        n478 = call-poly "Variant to Data.vi"("Variant"=w1168) -> ("String Array"=w1167:string[])  [unwired: 8 in]
        n479 = Unbundle By Name(w1173) -> ("Palette Name [# Colors,int?,inv?]"=w1170:string)
        n480 = Merge Errors(w1172, w1157) -> (w1158:errorcluster)
        n481 = call "Check Selected Palette in Menu.vi"("Error In"=w1158, "Palette List"=w1167, "Checked Palette"=w1170, "Menu in"=w1178) -> ("Error Out"=w1159:errorcluster, "Stored Palette List"=w1165:string[], "menu reference out"=w1154:refnum<k9>)  [unwired: 5 in]
        n482 = call "Alligator Variables Storage.vi"("Get(F)/Set"=TRUE, "AlliGator Variable"=w1164, "Error In"=w1159, "Data in"=w1165) -> ("Error Out"=w1156:errorcluster)  [unwired: 5 in, 2 out]
        n483 = call "AlliGator Add Python Functions to Object Menu.vi"("error in (no error)"=w1156, "Menu in"=w1154, "Object Refnum"=w1155) -> ("error out"=w1153:errorcluster)  [unwired: 6 in, 2 out]
        n484 = event-data() -> ()  [unwired: 2 in, 1 out]
      }
      event "Source Image": Shortcut Menu Selection (User) {
        n485 = event-data() -> ("CtlRef"=w1193:refnum<vi>, "ItemTag"=w1189:string, "ItemPath"=w1192:string, "Coords"=w1187:T35)  [unwired: 1 in]
        n486 = call-poly <vilib>:"Acquire Input Data.vi"("device ID"=w1185, "error in (no error)"=w1183) -> ("device ID"=w1186:refnum<k1>, "keys pressed"=w1182:T49, "error out"=w1184:errorcluster)  [unwired: 15 in]
        n487 = case shown="True" w1188 {
          tunnel: w1193 -> [_ w1198]
          tunnel: w1192 -> [_ w1204]
          tunnel: w1189 -> [_ w1202]
          tunnel: w1187 -> [_ w1203]
          tunnel: w1182 -> [_ w1201]
          tunnel: [_ w1196] -> w1181
          tunnel: [_ w1195] -> w1180
          tunnel: [_ w1194] -> w1179
          frame False {
          }
          frame True {
            n488 = Index Array(array=w1201) -> (element=w1200:T32)  [unwired: 1 in]
            n489 = Equal?(x=w1200, y=T32."H" ("element")) -> (x = y?=w1197:bool)
            n490 = case shown="False" w1197 {
              tunnel: w1204 -> [w1212 _]
              tunnel: w1203 -> [w1211 _]
              tunnel: w1202 -> [w1209 w1215]
              tunnel: w1198 -> [w1208 w1217]
              tunnel: [w1206 _] -> w1196
              tunnel: [_ w1214] -> w1195
              tunnel: [w1205 w1213] -> w1194
              frame False {
                n491 = Bundle By Name(cluster=T33 {"Item Tag"="", "Image Control Refnum"=refnum, "Coords"={"Horizontal"=0, "Vertical"=0}, "Item Path"=""} ("Image Event"), "Image Control Refnum"=w1208, "Item Tag"=w1209, "Item Path"=w1212, "Coords"=w1211) -> (w1207:T33)
                n492 = call "AlliGator Source Image Context Menu Handler.vi"("Image Event Data"=w1207) -> ("Error Out"=w1205:errorcluster, "AlliGator Actions"=w1206:T25[])  [unwired: 9 in]
              }
              frame True {
                n493 = property class="ImageControl"(reference=w1217) -> ("Label.Text"=w1216:string)  [unwired: 1 in, 2 out]
                n494 = call "AlliGator Send Python Function Doc String to Notebook.vi"("Item Tag"=w1215, "Target"=w1216) -> ("Error Out"=w1213:errorcluster, "Message"=w1214:string)  [unwired: 8 in]
              }
            }
          }
        }
      }
      event "Time Point Slide": Value Change {
        # "Time Point Slider: Mouse Up, Mouse Leave"
        n495 = event-data() -> ("CtlRef"=w1225:refnum<vi>, "OldVal"=w1218:u16)  [unwired: 1 in]
        n496 = case shown="True" w1226 {
          tunnel: w1225 -> [w1229 w1233]
          tunnel: [w1227 w1230] -> w1220
          tunnel: [_ w1231] -> w1219
          tunnel: w1218 -> [w1228 _]
          frame False {
            n497 = property class="Slide (strict)"(reference=w1229, "Value"=w1228) -> (error out=w1227:errorcluster)  [unwired: 1 in, 1 out]
          }
          frame True {
            n498 = property class="Slide (strict)"(reference=w1233) -> (error out=w1230:errorcluster, "Value"=w1232:u16)  [unwired: 1 in, 1 out]
            n499 = Bundle By Name(cluster=T25 {"AlliGator Q Event"=enum."GUI:Time Series Slider Changed", "Data"=variant} ("Time-Gated Phasor Q Element"), "Data"=w1232) -> (w1234:T25)
            n500 = Build Array(w1234) -> (w1231:T25[])
          }
        }
      }
      event "Time Step": Value Change {
        n501 = event-data() -> ("CtlRef"=w1247:refnum<vi>)  [unwired: 1 in]
        n502 = property class="DigNum (strict)"(reference=w1247) -> (reference out=w1244:refnum<vi>, error out=w1239:errorcluster, "Label.Text"=w1250:string, "Value"=w1245:dbl[unit])  [unwired: 1 in]
        n503 = call "AlliGator Update Settings & Control.vi"("Error In"=w1239, "Value"=w1245, "Sender"=w1246, "CtlRef"=w1244) -> ("Error Out"=w1238:errorcluster)  [unwired: 7 in]
        n504 = node(w1245) -> (w1248:dbl)
        n505 = property on="Intensity Time Trace" class="XYGraph (strict)"(error in=w1238, "XScale.Multiplier"=w1248) -> (error out=w1237:errorcluster)  [unwired: 1 in, 1 out]
        n506 = call "AlliGator Get Control Notebook String.vi"("error in (no error)"=w1237, "Value"=w1245, "Control Label"=w1250) -> ("error out"=w1249:errorcluster, "Notebook String"=w1236:string)  [unwired: 7 in]
      }
      event "Use File Timestamp": Value Change {
        n507 = event-data() -> ("CtlRef"=w1258:refnum<vi>, "OldVal"=w1257:bool, "NewVal"=w1260:bool)  [unwired: 1 in]
        n508 = case shown="True" w1259 {
          tunnel: w1260 -> [_ w1265]
          tunnel: w1258 -> [w1263 _]
          tunnel: w1257 -> [w1262 _]
          tunnel: [w1261 _] -> w1252
          tunnel: [_ w1264] -> w1251
          frame False {
            n509 = property class="Bool (strict)"(reference=w1263, "Value"=w1262) -> (error out=w1261:errorcluster)  [unwired: 1 in, 1 out]
          }
          frame True {
            n510 = Bundle By Name(cluster=T25 {"AlliGator Q Event"=enum."Intensity Time Trace:Use File Timestamp", "Data"=variant} ("element"), "Data"=w1265) -> (w1266:T25)
            n511 = Build Array(w1266) -> (w1264:T25[])
          }
        }
      }
      event "Use Intensity Correction File": Value Change {
        n512 = event-data() -> ("NewVal"=w1277:bool, "CtlRef"=w1278:refnum<vi>, "OldVal"=w1275:bool)  [unwired: 1 in]
        n513 = case shown="True" w1276 {
          tunnel: w1279 -> [_ w1292]
          tunnel: w1278 -> [w1282 w1290]
          tunnel: w1277 -> [_ w1288]
          tunnel: w1275 -> [w1281 _]
          tunnel: [w1280 w1291] -> w1270
          tunnel: [_ w1284] -> w1269
          tunnel: [_ w1283] -> w1268
          frame False {
            n514 = property class="Bool (strict)"(reference=w1282, "Value"=w1281) -> (error out=w1280:errorcluster)  [unwired: 1 in, 1 out]
          }
          frame True {
            n515 = local read "Intensity Correction File"() -> (w1287:path)
            n516 = property class="Bool (strict)"(reference=w1290) -> (reference out=w1294:refnum<vi>, error out=w1286:errorcluster, "Label.Text"=w1295:string, "Value"=w1293:bool)  [unwired: 1 in]
            n517 = Empty String/Path?(string/path=w1287) -> (empty?=w1296:bool)
            n518 = Compound Arithmetic op=AND(w1288, invert w1296) -> (w1289:bool)
            n519 = case shown="True" w1289 {
              tunnel: w1287 -> [_ w1298]
              tunnel: [_ w1297] -> w1284
              frame False {
              }
              frame True {
                n520 = Bundle By Name(cluster=T25 {"AlliGator Q Event"=enum."Intensity Time Trace:Load Intensity Corrections File", "Data"=variant} ("Time-Gated Phasor Q Element"), "Data"=w1298) -> (w1299:T25)
                n521 = Build Array(w1299) -> (w1297:T25[])
              }
            }
            n522 = call "AlliGator Update Settings & Control.vi"("Error In"=w1286, "Value"=w1293, "Sender"=w1292, "CtlRef"=w1294) -> ("Error Out"=w1285:errorcluster)  [unwired: 7 in]
            n523 = call "AlliGator Get Control Notebook String.vi"("error in (no error)"=w1285, "Value"=w1293, "Control Label"=w1295) -> ("error out"=w1291:errorcluster, "Notebook String"=w1283:string)  [unwired: 7 in]
          }
        }
      }
      event "Use ROI as Search Area": Value Change {
        n524 = event-data() -> ("CtlRef"=w1307:refnum<vi>, "NewVal"=w1309:bool, "OldVal"=w1306:bool)  [unwired: 1 in]
        n525 = case shown="True" w1308 {
          tunnel: w1310 -> [_ _]
          tunnel: w1309 -> [_ w1314]
          tunnel: w1307 -> [w1312 _]
          tunnel: w1306 -> [w1311 _]
          tunnel: [_ T25[] [{"AlliGator Q Event"=enum."Image:Use ROI as Search Area", "Data"=variant}] ("element")] -> w1301
          frame False {
            n526 = property class="Bool (strict)"(reference=w1312, "Value"=w1311) -> ()  [unwired: 1 in, 2 out]
          }
          frame True {
            n527 = call "Alligator Variables Storage.vi"("Get(F)/Set"=TRUE, "AlliGator Variable"=AlliGator_Variables_List."GUI:Search ROI Used" ("Alligator Variable"), "Data in"=w1314) -> ()  [unwired: 6 in, 3 out]
          }
        }
      }
      event Mouse Enter {
        # "Decay Fit Parameter Map Display: Mouse Enter"
        n528 = event-data() -> ("CtlRef"=w1322:refnum<vi>)  [unwired: 1 in]
        n529 = case shown="True" w1323 {
          tunnel: [w1326 w1331] -> w1325
          tunnel: w1324 -> [w1326 w1330]
          tunnel: w1322 -> [_ w1328]
          tunnel: [_ w1327] -> w1317
          frame False {
          }
          frame True {
            n530 = Unbundle By Name(w1330) -> ("Decay Fit Parameter Map Display Event"=w1332:refnum<event-registration>)
            n531 = register-events(reference=w1332, T34 refnum ("event source"), w1328, w1328) -> (reference out=w1333:refnum<event-registration>, error out=w1327:errorcluster)  [unwired: 1 in]
            n532 = Bundle By Name(cluster=w1330, "Decay Fit Parameter Map Display Event"=w1333) -> (w1331:T26)
          }
        }
      }
      event Mouse Leave {
        # "Decay Fit Parameter Map Display: Mouse Leave"
        n533 = event-data() -> ("CtlRef"=w1339:refnum<vi>)  [unwired: 1 in]
        n534 = case shown="True" w1340 {
          tunnel: [w1343 w1348] -> w1342
          tunnel: w1341 -> [w1343 w1347]
          tunnel: w1339 -> [_ w1346]
          tunnel: [_ w1344] -> w1334
          frame False {
          }
          frame True {
            w1345 = refnum<vi> refnum ("event source")
            n535 = Unbundle By Name(w1347) -> ("Decay Fit Parameter Map Display Event"=w1349:refnum<event-registration>)
            n536 = register-events(reference=w1349, w1346, w1345, w1345) -> (reference out=w1350:refnum<event-registration>, error out=w1344:errorcluster)  [unwired: 1 in]
            n537 = Bundle By Name(cluster=w1347, "Decay Fit Parameter Map Display Event"=w1350) -> (w1348:T26)
          }
        }
      }
      event Mouse Up {
        # "Decay Fit Parameter Map Display: Mouse Up"
        n538 = event-data() -> ("CtlRef"=w1357:refnum<vi>)  [unwired: 1 in]
        n539 = case shown="True" w1356 {
          tunnel: w1357 -> [_ w1359]
          tunnel: [_ w1358] -> w1353
          frame False {
          }
          frame True {
            n540 = Bundle By Name(cluster=T25 {"AlliGator Q Event"=enum."Decay Fit Parameter Map:Mouse Up", "Data"=variant} ("Array"), "Data"=w1359) -> (w1360:T25)
            n541 = Build Array(w1360) -> (w1358:T25[])
          }
        }
      }
      event Mouse Down {
        w1366 = refnum<vi> refnum  # Decay Fit Parameter Map Display Range
        # "Decay Fit Parameter Map Display Range: Mouse Down"
        n542 = event-data() -> ("CtlRef"=w1365:refnum<vi>)  [unwired: 1 in]
        n543 = Unbundle By Name(w1371) -> ("Decay Fit Parameter Map Display Range Event"=w1369:refnum<event-registration>)
        n544 = register-events(reference=w1369, w1366, w1365, w1365, w1365) -> (reference out=w1370:refnum<event-registration>, error out=w1362:errorcluster)  [unwired: 1 in]
        n545 = Bundle By Name(cluster=w1371, "Decay Fit Parameter Map Display Range Event"=w1370) -> (w1372:T26)
      }
      event Mouse Leave {
        w1376 = refnum<vi> refnum  # Decay Fit Parameter Map Display Range
        # "Decay Fit Parameter Map Display Range: Mouse Up, Mouse Leave"
        n546 = event-data() -> ("CtlRef"=w1377:refnum<vi>)  [unwired: 1 in]
        n547 = Unbundle By Name(w1382) -> ("Decay Fit Parameter Map Display Range Event"=w1380:refnum<event-registration>)
        n548 = register-events(reference=w1380, w1377, w1376, w1376, w1376) -> (reference out=w1381:refnum<event-registration>, error out=w1373:errorcluster)  [unwired: 1 in]
        n549 = Bundle By Name(cluster=w1382, "Decay Fit Parameter Map Display Range Event"=w1381) -> (w1383:T26)
      }
      event Mouse Move {
        # "Decay Fit Parameter Map Display Range: Mouse Move"
        n550 = event-data() -> ("Time"=w1385:u32)  [unwired: 1 in]
        n551 = case shown="True" w1392 {
          tunnel: [_ w1400] -> w1386
          tunnel: w1385 -> [_ w1396]
          tunnel: w1384 -> [_ w1393]
          frame False {
          }
          frame True {
            w1395 = T25 {"AlliGator Q Event"=enum."Decay Fit Parameter Map:Display Range Mouse Move", "Data"=variant} ("Time-Gated Phasor Q Element")
            n552 = Unbundle By Name(w1395) -> ("AlliGator Q Event"=w1399:T24)
            n553 = Bundle By Name(cluster=T39 {"AlliGator Q Event"=enum."---- Files ----", "Time"=0, "Timeout"=0} ("output cluster"), "AlliGator Q Event"=w1399, "Time"=w1396, "Timeout"=w1393) -> (w1397:T39)
            n554 = call "AlliGator Filter Event.vi"("Filtered Event Data"=w1397) -> ("Filter Event?"=w1394:bool)  [unwired: 9 in, 1 out]
            n555 = case shown="False" w1394 {
              tunnel: [w1403 _] -> w1400
              tunnel: w1395 -> [w1401 _]
              frame False {
                n556 = local read "Decay Fit Parameter"() -> (w1402:T11)
                n557 = Bundle By Name(cluster=w1401, "Data"=w1402) -> (w1404:T25)
                n558 = Build Array(w1404) -> (w1403:T25[])
              }
              frame True {
              }
            }
          }
        }
      }
      event Mouse Enter {
        # "Decay Graph Tipstrip: Mouse Enter"
        n559 = event-data() -> ("CtlRef"=w1413:refnum<vi>)  [unwired: 1 in]
        n560 = Unbundle By Name(w1412) -> ("Decay Graph Tipstrip Event"=w1414:refnum<event-registration>)
        n561 = call "Tipstrip Mouse Enter (XY Graph).vi"("Event Registration Refnum in"=w1414, "XYGraph Refnum"=w1413) -> ("Error Out"=w1407:errorcluster, "Event Registration Refnum out"=w1411:refnum<event-registration>)  [unwired: 8 in]
        n562 = Bundle By Name(cluster=w1412, "Decay Graph Tipstrip Event"=w1411) -> (w1410:T26)
      }
      event Mouse Leave {
        # "Decay Graph Tipstrip: Mouse Leave"
        n563 = event-data() -> ("CtlRef"=w1421:refnum<vi>)  [unwired: 1 in]
        n564 = Unbundle By Name(w1425) -> ("Decay Graph Tipstrip Event"=w1423:refnum<event-registration>)
        n565 = control-ref of="Decay Graph TipStrip"() -> (w1420:refnum<vi>)
        n566 = call "Tipstrip Mouse Leave (XY Graph).vi"("TipStrip Refnum"=w1420, "Event Registration Refnum in"=w1423, "XYGraph Refnum"=w1421) -> ("Error Out"=w1417:errorcluster, "Event Registration Refnum out"=w1422:refnum<event-registration>)  [unwired: 7 in]
        n567 = Bundle By Name(cluster=w1425, "Decay Graph Tipstrip Event"=w1422) -> (w1424:T26)
      }
      event Mouse Move {
        # "Decay Graph Tipstrip: Mouse Move"
        n568 = event-data() -> ("Time"=w1428:u32, "CtlRef"=w1439:refnum<vi>, "Coords"=w1438:T35)  [unwired: 1 in]
        n569 = Unbundle By Name(T25 {"AlliGator Q Event"=enum."Decay:Graph Tip Strip Update", "Data"=variant} ("Time-Gated Phasor Q Element")) -> ("AlliGator Q Event"=w1432:T24)
        n570 = Bundle By Name(cluster=T39 {"AlliGator Q Event"=enum."---- Files ----", "Time"=0, "Timeout"=0} ("output cluster"), "AlliGator Q Event"=w1432, "Time"=w1428, "Timeout"=w1427) -> (w1430:T39)
        n571 = call "AlliGator Filter Event.vi"("Filtered Event Data"=w1430) -> ("Filter Event?"=w1429:bool)  [unwired: 9 in, 1 out]
        n572 = case shown="False" w1429 {
          tunnel: w1439 -> [w1443 _]
          tunnel: w1438 -> [w1442 _]
          tunnel: [w1440 _] -> w1435
          frame False {
            n573 = control-ref of="Decay Graph TipStrip"() -> (w1441:refnum<vi>)
            n574 = call "Set Plot TipStrip (XY Graph).vi"("TipStrip Refnum"=w1441, "Coords"=w1442, "XY Graph Refnum"=w1443) -> ("Error Out"=w1440:errorcluster)  [unwired: 6 in, 2 out]
          }
          frame True {
          }
        }
      }
      event Mouse Enter {
        # "Decay Statistics Graph Tipstrip: Mouse Enter"
        n575 = event-data() -> ("CtlRef"=w1452:refnum<vi>)  [unwired: 1 in]
        n576 = Unbundle By Name(w1451) -> ("Decay Statistics Graph Tipstrip Event"=w1453:refnum<event-registration>)
        n577 = call "Tipstrip Mouse Enter (XY Graph).vi"("Event Registration Refnum in"=w1453, "XYGraph Refnum"=w1452) -> ("Error Out"=w1444:errorcluster, "Event Registration Refnum out"=w1450:refnum<event-registration>)  [unwired: 8 in]
        n578 = Bundle By Name(cluster=w1451, "Decay Statistics Graph Tipstrip Event"=w1450) -> (w1449:T26)
      }
      event Mouse Leave {
        # "Decay Statistics Graph Tipstrip: Mouse Leave"
        n579 = event-data() -> ("CtlRef"=w1460:refnum<vi>)  [unwired: 1 in]
        n580 = Unbundle By Name(w1464) -> ("Decay Statistics Graph Tipstrip Event"=w1462:refnum<event-registration>)
        n581 = control-ref of="Decay Statistics Graph TipStrip"() -> (w1459:refnum<vi>)
        n582 = call "Tipstrip Mouse Leave (XY Graph).vi"("TipStrip Refnum"=w1459, "Event Registration Refnum in"=w1462, "XYGraph Refnum"=w1460) -> ("Error Out"=w1456:errorcluster, "Event Registration Refnum out"=w1461:refnum<event-registration>)  [unwired: 7 in]
        n583 = Bundle By Name(cluster=w1464, "Decay Statistics Graph Tipstrip Event"=w1461) -> (w1463:T26)
      }
      event Mouse Move {
        # "Decay Statistics Graph Tipstrip: Mouse Move"
        n584 = event-data() -> ("Time"=w1467:u32, "CtlRef"=w1478:refnum<vi>, "Coords"=w1477:T35)  [unwired: 1 in]
        n585 = Unbundle By Name(T25 {"AlliGator Q Event"=enum."Decay Statistics:Tip Strip Update", "Data"=variant} ("Time-Gated Phasor Q Element")) -> ("AlliGator Q Event"=w1471:T24)
        n586 = Bundle By Name(cluster=T39 {"AlliGator Q Event"=enum."---- Files ----", "Time"=0, "Timeout"=0} ("output cluster"), "AlliGator Q Event"=w1471, "Time"=w1467, "Timeout"=w1465) -> (w1469:T39)
        n587 = call "AlliGator Filter Event.vi"("Filtered Event Data"=w1469) -> ("Filter Event?"=w1466:bool)  [unwired: 9 in, 1 out]
        n588 = case shown="False" w1466 {
          tunnel: w1478 -> [w1482 _]
          tunnel: w1477 -> [w1481 _]
          tunnel: [w1479 _] -> w1474
          frame False {
            n589 = control-ref of="Decay Statistics Graph TipStrip"() -> (w1480:refnum<vi>)
            n590 = call "Set Plot TipStrip (XY Graph).vi"("TipStrip Refnum"=w1480, "Coords"=w1481, "XY Graph Refnum"=w1482) -> ("Error Out"=w1479:errorcluster)  [unwired: 6 in, 2 out]
          }
          frame True {
          }
        }
      }
      event Mouse Enter {
        # "Intensity Time Trace Tipstrip: Mouse Enter"
        n591 = event-data() -> ("CtlRef"=w1491:refnum<vi>)  [unwired: 1 in]
        n592 = Unbundle By Name(w1490) -> ("Intensity Time Trace Tipstrip Event"=w1492:refnum<event-registration>)
        n593 = call "Tipstrip Mouse Enter (XY Graph).vi"("Event Registration Refnum in"=w1492, "XYGraph Refnum"=w1491) -> ("Error Out"=w1485:errorcluster, "Event Registration Refnum out"=w1489:refnum<event-registration>)  [unwired: 8 in]
        n594 = Bundle By Name(cluster=w1490, "Intensity Time Trace Tipstrip Event"=w1489) -> (w1488:T26)
      }
      event Mouse Leave {
        # "Intensity Time Trace Tipstrip: Mouse Leave"
        n595 = event-data() -> ("CtlRef"=w1499:refnum<vi>)  [unwired: 1 in]
        n596 = Unbundle By Name(w1503) -> ("Intensity Time Trace Tipstrip Event"=w1501:refnum<event-registration>)
        n597 = control-ref of="Intensity Time Trace TipStrip"() -> (w1498:refnum<vi>)
        n598 = call "Tipstrip Mouse Leave (XY Graph).vi"("TipStrip Refnum"=w1498, "Event Registration Refnum in"=w1501, "XYGraph Refnum"=w1499) -> ("Error Out"=w1495:errorcluster, "Event Registration Refnum out"=w1500:refnum<event-registration>)  [unwired: 7 in]
        n599 = Bundle By Name(cluster=w1503, "Intensity Time Trace Tipstrip Event"=w1500) -> (w1502:T26)
      }
      event Mouse Move {
        # "Intensity Time Trace Tipstrip: Mouse Move"
        n600 = event-data() -> ("Time"=w1507:u32, "CtlRef"=w1517:refnum<vi>, "Coords"=w1516:T35)  [unwired: 1 in]
        n601 = Unbundle By Name(T25 {"AlliGator Q Event"=enum."Intensity Time Trace:Tip Strip Update", "Data"=variant} ("Named Q Element")) -> ("AlliGator Q Event"=w1510:T24)
        n602 = Bundle By Name(cluster=T39 {"AlliGator Q Event"=enum."---- Files ----", "Time"=0, "Timeout"=0} ("output cluster"), "AlliGator Q Event"=w1510, "Time"=w1507, "Timeout"=w1504) -> (w1508:T39)
        n603 = call "AlliGator Filter Event.vi"("Filtered Event Data"=w1508) -> ("Filter Event?"=w1505:bool)  [unwired: 9 in, 1 out]
        n604 = case shown="False" w1505 {
          tunnel: w1517 -> [w1521 _]
          tunnel: w1516 -> [w1520 _]
          tunnel: [w1518 _] -> w1513
          frame False {
            n605 = control-ref of="Intensity Time Trace TipStrip"() -> (w1519:refnum<vi>)
            n606 = call "Set Plot TipStrip (XY Graph).vi"("TipStrip Refnum"=w1519, "Coords"=w1520, "XY Graph Refnum"=w1521) -> ("Error Out"=w1518:errorcluster)  [unwired: 6 in, 2 out]
          }
          frame True {
          }
        }
      }
      event Mouse Enter {
        # "Lifetime Graph Tipstrip: Mouse Enter"
        n607 = event-data() -> ("CtlRef"=w1530:refnum<vi>)  [unwired: 1 in]
        n608 = Unbundle By Name(w1529) -> ("Lifetime Graph Tipstrip Event"=w1531:refnum<event-registration>)
        n609 = call "Tipstrip Mouse Enter (XY Graph).vi"("Event Registration Refnum in"=w1531, "XYGraph Refnum"=w1530) -> ("Error Out"=w1524:errorcluster, "Event Registration Refnum out"=w1528:refnum<event-registration>)  [unwired: 8 in]
        n610 = Bundle By Name(cluster=w1529, "Lifetime Graph Tipstrip Event"=w1528) -> (w1527:T26)
      }
      event Mouse Leave {
        # "Lifetime Graph Tipstrip: Mouse Leave"
        n611 = event-data() -> ("CtlRef"=w1538:refnum<vi>)  [unwired: 1 in]
        n612 = Unbundle By Name(w1542) -> ("Lifetime Graph Tipstrip Event"=w1540:refnum<event-registration>)
        n613 = control-ref of="Lifetime & Other Parameters Graph TipStrip"() -> (w1537:refnum<vi>)
        n614 = call "Tipstrip Mouse Leave (XY Graph).vi"("TipStrip Refnum"=w1537, "Event Registration Refnum in"=w1540, "XYGraph Refnum"=w1538) -> ("Error Out"=w1534:errorcluster, "Event Registration Refnum out"=w1539:refnum<event-registration>)  [unwired: 7 in]
        n615 = Bundle By Name(cluster=w1542, "Lifetime Graph Tipstrip Event"=w1539) -> (w1541:T26)
      }
      event Mouse Move {
        # "Lifetime Graph Tipstrip: Mouse Move"
        n616 = event-data() -> ("Time"=w1546:u32, "CtlRef"=w1556:refnum<vi>, "Coords"=w1555:T35)  [unwired: 1 in]
        n617 = Unbundle By Name(T25 {"AlliGator Q Event"=enum."Lifetime:Tip Strip Update", "Data"=variant} ("Named Q Element")) -> ("AlliGator Q Event"=w1549:T24)
        n618 = Bundle By Name(cluster=T39 {"AlliGator Q Event"=enum."---- Files ----", "Time"=0, "Timeout"=0} ("output cluster"), "AlliGator Q Event"=w1549, "Time"=w1546, "Timeout"=w1543) -> (w1547:T39)
        n619 = call "AlliGator Filter Event.vi"("Filtered Event Data"=w1547) -> ("Filter Event?"=w1544:bool)  [unwired: 9 in, 1 out]
        n620 = case shown="False" w1544 {
          tunnel: w1556 -> [w1560 _]
          tunnel: w1555 -> [w1559 _]
          tunnel: [w1557 _] -> w1552
          frame False {
            n621 = control-ref of="Lifetime & Other Parameters Graph TipStrip"() -> (w1558:refnum<vi>)
            n622 = call "Set Plot TipStrip (XY Graph).vi"("TipStrip Refnum"=w1558, "Coords"=w1559, "XY Graph Refnum"=w1560) -> ("Error Out"=w1557:errorcluster)  [unwired: 6 in, 2 out]
          }
          frame True {
          }
        }
      }
      event User Event {
        # "AlliGator Settings: User Event"
        n623 = event-data() -> ("AlliGator Settings Message"=w1570:T54, "Sender"=w1568:string, "Control Label"=w1571:string, "Data"=w1569:variant)  [unwired: 1 in]
        n624 = Not Equal?(x=w1567, y=w1568) -> (x != y?=w1572:bool)
        n625 = case shown="True" w1572 {
          tunnel: w1571 -> [_ w1576]
          tunnel: w1570 -> [_ w1577]
          tunnel: w1561 -> [_ w1575]
          tunnel: w1569 -> [_ w1574]
          tunnel: [_ w1573] -> w1564
          frame False {
          }
          frame True {
            n626 = case shown="\"Refresh Parameter\"" w1577 {
              tunnel: w1576 -> [_ _ _ w1583 _]
              tunnel: w1575 -> [_ _ _ w1578 _]
              tunnel: w1574 -> [_ _ _ w1582 _]
              tunnel: [_ _ _ w1580 _] -> w1573
              frame "Idle", Default {
              }
              frame "Subscribe" {
              }
              frame "Unsubscribe" {
              }
              frame "Refresh Parameter" {
                n627 = call "AlliGator Refresh Single Setting.vi"("Data"=w1582, "Control Label"=w1583, "VI Ref in"=w1578) -> ("Error Out"=w1581:errorcluster, "VI Ref (dup)"=w1579:refnum<vi>)  [unwired: 7 in]
                n628 = case shown="\"\", Default" w1583 {
                  tunnel: w1579 -> [_ w1590 w1595 w1602]
                  tunnel: w1582 -> [_ w1588 w1593 w1601]
                  tunnel: w1581 -> [w1585 w1587 w1592 w1600]
                  tunnel: [w1584 w1586 w1591 w1597] -> w1580
                  frame "", Default {
                    n629 = call "Clear Error.vi"("Error In"=w1585) -> ("no Error Out"=w1584:errorcluster)  [unwired: 8 in]
                  }
                  frame "Phasor Graph Frequency" {
                    n630 = call "AlliGator Refresh Single Setting.vi"("Error In"=w1587, "Data"=w1588, "Control Label"="Phasor Plot Frequency", "VI Ref in"=w1590) -> ("Error Out"=w1586:errorcluster)  [unwired: 6 in, 1 out]
                  }
                  frame "Phasor Plot Frequency" {
                    n631 = call "AlliGator Refresh Single Setting.vi"("Error In"=w1592, "Data"=w1593, "Control Label"="Phasor Graph Frequency", "VI Ref in"=w1595) -> ("Error Out"=w1591:errorcluster)  [unwired: 6 in, 1 out]
                  }
                  frame "Phasor Frequency" {
                    n632 = call "Clear Error.vi"("Error In"=w1600) -> ("no Error Out"=w1596:errorcluster)  [unwired: 8 in]
                    n633 = call "AlliGator Refresh Single Setting.vi"("Error In"=w1596, "Data"=w1601, "Control Label"="Phasor Graph Frequency", "VI Ref in"=w1602) -> ("Error Out"=w1599:errorcluster)  [unwired: 6 in, 1 out]
                    n634 = call "AlliGator Refresh Single Setting.vi"("Error In"=w1596, "Data"=w1601, "Control Label"="Phasor Plot Frequency", "VI Ref in"=w1602) -> ("Error Out"=w1598:errorcluster)  [unwired: 6 in, 1 out]
                    n635 = Merge Errors(w1599, w1598) -> (w1597:errorcluster)
                  }
                }
              }
              frame "Refresh All Parameters" {
              }
            }
          }
        }
      }
      event User Event {
        # "Phasor Plot Color Map Picker: User Event"
        n636 = event-data() -> ("Phasor Color Map Picker Event"=w1611:T55)  [unwired: 1 in]
        n637 = case shown="True" w1610 {
          tunnel: w1611 -> [_ w1613]
          tunnel: [_ w1612] -> w1605
          frame False {
          }
          frame True {
            n638 = case shown="\"Vertex Update\"" w1613 {
              tunnel: [_ T25[] [{"AlliGator Q Event"=enum."Phasor Plot:Update Phasor Color Map Vertices", "Data"=variant}] ("element") _] -> w1612
              frame "Init", Default {
              }
              frame "Vertex Update" {
              }
              frame "Color Change" {
              }
            }
          }
        }
      }
      event Mouse Down {
        w1620 = refnum<vi> refnum  # Phasor Plot Display Range
        # "Phasor Plot Display Range: Mouse Down"
        n639 = event-data() -> ("CtlRef"=w1621:refnum<vi>)  [unwired: 1 in]
        n640 = Unbundle By Name(w1624) -> ("Phasor Display Range Event"=w1622:refnum<event-registration>)
        n641 = register-events(reference=w1622, w1620, w1621, w1621, w1621) -> (reference out=w1623:refnum<event-registration>, error out=w1615:errorcluster)  [unwired: 1 in]
        n642 = Bundle By Name(cluster=w1624, "Phasor Display Range Event"=w1623) -> (w1625:T26)
      }
      event Mouse Move {
        # "Phasor Plot Display Range: Mouse Move"
        n643 = event-data() -> ("Time"=w1628:u32)  [unwired: 1 in]
        n644 = case shown="True" w1634 {
          tunnel: w1628 -> [_ w1639]
          tunnel: [_ w1636] -> w1627
          tunnel: w1626 -> [_ w1635]
          frame False {
          }
          frame True {
            w1637 = T25 {"AlliGator Q Event"=enum."Phasor Plot:Display Range Mouse Move", "Data"=variant} ("Time-Gated Phasor Q Element")
            n645 = Unbundle By Name(w1637) -> ("AlliGator Q Event"=w1642:T24)
            n646 = Bundle By Name(cluster=T39 {"AlliGator Q Event"=enum."---- Files ----", "Time"=0, "Timeout"=0} ("output cluster"), "AlliGator Q Event"=w1642, "Time"=w1639, "Timeout"=w1635) -> (w1640:T39)
            n647 = call "AlliGator Filter Event.vi"("Filtered Event Data"=w1640) -> ("Filter Event?"=w1638:bool)  [unwired: 9 in, 1 out]
            n648 = case shown="False" w1638 {
              tunnel: w1637 -> [w1644 _]
              tunnel: [w1643 _] -> w1636
              frame False {
                n649 = Build Array(w1644) -> (w1643:T25[])
              }
              frame True {
              }
            }
          }
        }
      }
      event Mouse Up; Mouse Leave {
        w1649 = refnum<vi> refnum  # Phasor Plot Display Range
        # "Phasor Plot Display Range: Mouse Up, Mouse Leave"
        n650 = event-data() -> ("CtlRef"=w1648:refnum<vi>)  [unwired: 1 in]
        n651 = Unbundle By Name(w1654) -> ("Phasor Display Range Event"=w1652:refnum<event-registration>)
        n652 = register-events(reference=w1652, w1648, w1649, w1649, w1649) -> (reference out=w1653:refnum<event-registration>, error out=w1645:errorcluster)  [unwired: 1 in]
        n653 = Bundle By Name(cluster=w1654, "Phasor Display Range Event"=w1653) -> (w1655:T26)
      }
      event Mouse Enter {
        # "Phasor Graph Tipstrip: Mouse Enter"
        n654 = event-data() -> ("CtlRef"=w1664:refnum<vi>)  [unwired: 1 in]
        n655 = Unbundle By Name(w1663) -> ("Phasor Graph Tipstrip Event"=w1665:refnum<event-registration>)
        n656 = call "Tipstrip Mouse Enter (XY Graph).vi"("Event Registration Refnum in"=w1665, "XYGraph Refnum"=w1664) -> ("Error Out"=w1658:errorcluster, "Event Registration Refnum out"=w1662:refnum<event-registration>)  [unwired: 8 in]
        n657 = Bundle By Name(cluster=w1663, "Phasor Graph Tipstrip Event"=w1662) -> (w1661:T26)
      }
      event Mouse Leave {
        # "Phasor Graph Tipstrip: Mouse Leave"
        n658 = event-data() -> ("CtlRef"=w1672:refnum<vi>)  [unwired: 1 in]
        n659 = Unbundle By Name(w1676) -> ("Phasor Graph Tipstrip Event"=w1674:refnum<event-registration>)
        n660 = control-ref of="Phasor Graph TipStrip"() -> (w1671:refnum<vi>)
        n661 = call "Tipstrip Mouse Leave (XY Graph).vi"("TipStrip Refnum"=w1671, "Event Registration Refnum in"=w1674, "XYGraph Refnum"=w1672) -> ("Error Out"=w1668:errorcluster, "Event Registration Refnum out"=w1673:refnum<event-registration>)  [unwired: 7 in]
        n662 = Bundle By Name(cluster=w1676, "Phasor Graph Tipstrip Event"=w1673) -> (w1675:T26)
      }
      event Mouse Move {
        # "Phasor Graph Tipstrip: Mouse Move"
        n663 = event-data() -> ("Time"=w1679:u32, "CtlRef"=w1690:refnum<vi>, "Coords"=w1689:T35)  [unwired: 1 in]
        n664 = Unbundle By Name(T25 {"AlliGator Q Event"=enum."Phasor Graph:Tip Strip Update", "Data"=variant} ("Named Q Element")) -> ("AlliGator Q Event"=w1683:T24)
        n665 = Bundle By Name(cluster=T39 {"AlliGator Q Event"=enum."---- Files ----", "Time"=0, "Timeout"=0} ("output cluster"), "AlliGator Q Event"=w1683, "Time"=w1679, "Timeout"=w1677) -> (w1681:T39)
        n666 = call "AlliGator Filter Event.vi"("Filtered Event Data"=w1681) -> ("Filter Event?"=w1678:bool)  [unwired: 9 in, 1 out]
        n667 = case shown="False" w1678 {
          tunnel: w1690 -> [w1694 _]
          tunnel: w1689 -> [w1693 _]
          tunnel: [w1691 _] -> w1686
          frame False {
            n668 = control-ref of="Phasor Graph TipStrip"() -> (w1692:refnum<vi>)
            n669 = call "Set Plot TipStrip (XY Graph).vi"("TipStrip Refnum"=w1692, "Coords"=w1693, "XY Graph Refnum"=w1694) -> ("Error Out"=w1691:errorcluster)  [unwired: 6 in, 2 out]
          }
          frame True {
          }
        }
      }
      event Mouse Down {
        # "Phasor Plot Display: Mouse Down"
        n670 = event-data() -> ("CtlRef"=w1707:refnum<vi>, "Coords"=w1706:T35, "Button"=w1705:u16, "PlatMods.Shift"=w1702:bool, "PlatMods.Alt"=w1701:bool)  [unwired: 1 in]
        n671 = case shown="True" w1695 {
          tunnel: w1707 -> [_ w1716]
          tunnel: w1706 -> [_ w1715]
          tunnel: w1705 -> [_ w1714]
          tunnel: w1704 -> [w1708 w1713]
          tunnel: [w1708 w1712] -> w1703
          tunnel: w1702 -> [_ w1711]
          tunnel: w1701 -> [_ w1710]
          tunnel: [_ w1709] -> w1698
          frame False {
          }
          frame True {
            n672 = case shown="1" w1714 {
              tunnel: w1716 -> [_ w1722]
              tunnel: w1715 -> [_ _]
              tunnel: w1713 -> [w1717 w1723]
              tunnel: [w1717 w1724] -> w1712
              tunnel: w1711 -> [_ _]
              tunnel: w1710 -> [_ _]
              tunnel: [_ w1721] -> w1709
              frame 0, Default {
                # "right or middle button"
              }
              frame 1 {
                # "Left Button: look for mouse up"
                n673 = Unbundle By Name(w1723) -> ("Phasor Plot Display Event"=w1720:refnum<event-registration>)
                n674 = call "AlliGator Phasor Plot Display Mouse Down-Up Event Monitoring.vi"("Phasor Plot Display Event Registration"=w1720, "Phasor Plot Display Refnum"=w1722, "Look for Mouse Down(T)/Up(F)"=FALSE) -> ("Phasor Plot Display Event Registration"=w1719:refnum<event-registration>, "Error Out"=w1721:errorcluster)  [unwired: 11 in]
                n675 = Bundle By Name(cluster=w1723, "Phasor Plot Display Event"=w1719) -> (w1724:T26)
              }
            }
          }
        }
      }
      event Mouse Enter {
        # "Phasor Plot Display: Mouse Enter"
        n676 = event-data() -> ("CtlRef"=w1731:refnum<vi>)  [unwired: 1 in]
        n677 = case shown="True" w1725 {
          tunnel: [w1734 w1739] -> w1733
          tunnel: w1732 -> [w1734 w1738]
          tunnel: w1731 -> [_ w1735]
          tunnel: [_ w1736] -> w1726
          frame False {
          }
          frame True {
            n678 = Unbundle By Name(w1738) -> ("Phasor Plot Display Event"=w1740:refnum<event-registration>)
            n679 = register-events(reference=w1740, T34 refnum ("event source"), w1735, w1735, w1735, w1735) -> (reference out=w1741:refnum<event-registration>, error out=w1736:errorcluster)  [unwired: 1 in]
            n680 = Bundle By Name(cluster=w1738, "Phasor Plot Display Event"=w1741) -> (w1739:T26)
          }
        }
      }
      event Mouse Leave {
        # "Phasor Plot Display: Mouse Leave"
        n681 = event-data() -> ("CtlRef"=w1747:refnum<vi>)  [unwired: 1 in]
        n682 = case shown="True" w1748 {
          tunnel: [w1751 w1757] -> w1750
          tunnel: w1749 -> [w1751 w1756]
          tunnel: w1747 -> [_ w1755]
          tunnel: [_ w1753] -> w1742
          frame False {
          }
          frame True {
            w1754 = FALSE ("Visible")
            w1752 = refnum<vi> refnum ("event source")
            n683 = Unbundle By Name(w1756) -> ("Phasor Plot Display Event"=w1758:refnum<event-registration>)
            n684 = register-events(reference=w1758, w1755, w1752, w1752, w1752, w1752) -> (reference out=w1759:refnum<event-registration>, error out=w1753:errorcluster)  [unwired: 1 in]
            n685 = Bundle By Name(cluster=w1756, "Phasor Plot Display Event"=w1759) -> (w1757:T26)
            n686 = property on="Phasor Plot Phasor Ratio" class="DigNum (strict)"("Visible"=w1754) -> ()  [unwired: 2 in, 2 out]
            n687 = property on="Phasor at cursor (g, s)" class="Clust (strict)"("Visible"=w1754) -> ()  [unwired: 2 in, 2 out]
            n688 = property on="Phasor at cursor (m, phi)" class="Clust (strict)"("Visible"=w1754) -> ()  [unwired: 2 in, 2 out]
            n689 = property on="Phasor Plot Phase Lifetime" class="DigNum (strict)"("Visible"=w1754) -> ()  [unwired: 2 in, 2 out]
            n690 = property on="Phasor Plot Average Lifetime" class="DigNum (strict)"("Visible"=w1754) -> ()  [unwired: 2 in, 2 out]
            n691 = property on="Phasor Plot Modulus Lifetime" class="DigNum (strict)"("Visible"=w1754) -> ()  [unwired: 2 in, 2 out]
          }
        }
      }
      event Mouse Move {
        # "Phasor Plot Display: Mouse Move"
        n692 = event-data() -> ("Time"=w1761:u32, "CtlRef"=w1773:refnum<vi>, "Coords"=w1772:T35)  [unwired: 1 in]
        n693 = case shown="True" w1763 {
          tunnel: w1773 -> [_ w1789]
          tunnel: w1772 -> [_ _]
          tunnel: w1771 -> [w1776 w1796]
          tunnel: w1770 -> [w1777 w1797]
          tunnel: [w1777 w1795] -> w1769
          tunnel: [w1776 w1791] -> w1768
          tunnel: w1764 -> [w1775 w1794]
          tunnel: w1766 -> [w1774 w1793]
          tunnel: [w1774 w1790] -> w1767
          tunnel: [w1775 w1792] -> w1765
          tunnel: [_ w1788] -> w1762
          tunnel: w1761 -> [_ w1783]
          tunnel: w1760 -> [_ w1782]
          frame False {
          }
          frame True {
            w1784 = T25 {"AlliGator Q Event"=enum."Phasor Plot:Mouse Move", "Data"=variant} ("AlliGator Actions")
            n694 = Unbundle By Name(w1784) -> ("AlliGator Q Event"=w1787:T24)
            n695 = Bundle By Name(cluster=T39 {"AlliGator Q Event"=enum."---- Files ----", "Time"=0, "Timeout"=0} ("output cluster"), "AlliGator Q Event"=w1787, "Time"=w1783, "Timeout"=w1782) -> (w1785:T39)
            n696 = call "AlliGator Phasor Plot Mouse Move Flag.vi"("Read/Write"=Read-Write."Read") -> ("Flag (out)"=w1779:bool)  [unwired: 8 in]
            n697 = call "AlliGator Filter Event.vi"("Filtered Event Data"=w1785) -> ("Filter Event?"=w1778:bool)  [unwired: 9 in, 1 out]
            n698 = Compound Arithmetic op=OR(w1778, w1779) -> (w1780:bool)
            n699 = case shown="False" w1780 {
              tunnel: w1797 -> [w1817 w1821]
              tunnel: w1796 -> [w1816 w1820]
              tunnel: [w1815 w1821] -> w1795
              tunnel: w1794 -> [w1814 w1819]
              tunnel: w1793 -> [w1813 w1818]
              tunnel: [w1812 w1819] -> w1792
              tunnel: [w1811 w1820] -> w1791
              tunnel: [w1810 w1818] -> w1790
              tunnel: w1789 -> [w1806 _]
              tunnel: [w1803 _] -> w1788
              tunnel: w1784 -> [w1800 _]
              frame False {
                n700 = property class="ImageControl"(reference=w1806) -> (reference out=w1802:refnum<vi>, "Last Mouse Position"=w1801:cluster{"X":i32, "Y":i32})  [unwired: 1 in, 1 out]
                n701 = call "AlliGator Phasor Plot Mouse Move Flag.vi"("Flag (in)"=TRUE, "Read/Write"=Read-Write."Write") -> ()  [unwired: 7 in, 1 out]
                n702 = call-poly <vilib>:"Acquire Input Data.vi"("device ID"=w1817, "error in (no error)"=w1816) -> ("device ID"=w1815:refnum<k1>, "button info"=w1808:T56, "error out"=w1811:errorcluster)  [unwired: 14 in, 1 out]
                n703 = call-poly <vilib>:"Acquire Input Data.vi"("device ID"=w1814, "error in (no error)"=w1813) -> ("device ID"=w1812:refnum<k1>, "keys pressed"=w1807:T49, "error out"=w1810:errorcluster)  [unwired: 15 in]
                n704 = Bundle(cluster=T43 {"Image Control Refnum"=refnum, "Coords"={"Horizontal"=0, "Vertical"=0}, "button info"={"button 1"=FALSE, "button 2"=FALSE, "button 3"=FALSE, "button 4"=FALSE}, "keys pressed"=[]} ("Image User Event Data"), "Image Control Refnum"=w1802, "Coords"=w1801, "button info"=w1808, "keys pressed"=w1807) -> (w1804:T43)
                n705 = Bundle By Name(cluster=w1800, "Data"=w1804) -> (w1809:T25)
                n706 = Build Array(w1809) -> (w1803:T25[])
              }
              frame True {
              }
            }
          }
        }
      }
      event Mouse Up {
        n707 = event-data() -> ("CtlRef"=w1834:refnum<vi>, "Button"=w1829:u16, "PlatMods.Shift"=w1832:bool, "PlatMods.Alt"=w1826:bool)  [unwired: 1 in]
        n708 = case shown="True" w1833 {
          tunnel: w1834 -> [_ w1843]
          tunnel: w1832 -> [_ w1841]
          tunnel: w1829 -> [_ w1842]
          tunnel: w1831 -> [w1835 w1840]
          tunnel: [w1835 w1839] -> w1830
          tunnel: w1826 -> [_ w1838]
          tunnel: [_ w1837] -> w1825
          tunnel: [_ w1836] -> w1822
          frame False {
          }
          frame True {
            n709 = case shown="1" w1842 {
              tunnel: w1843 -> [_ w1857]
              tunnel: w1841 -> [_ w1846]
              tunnel: w1840 -> [w1844 w1855]
              tunnel: [w1844 w1860] -> w1839
              tunnel: w1838 -> [_ w1845]
              tunnel: [_ w1852] -> w1837
              tunnel: [_ w1848] -> w1836
              frame 0, Default {
              }
              frame 1 {
                # "Left Button"
                n710 = property class="ImageControl"(reference=w1857) -> (error out=w1852:errorcluster, "Current ROI Tool"=w1854:u32, "ROI"=w1847:T57)  [unwired: 1 in, 1 out]
                n711 = Unbundle By Name(w1855) -> ("Phasor Plot Display Event"=w1859:refnum<event-registration>)
                n712 = Bundle(cluster=T44 {"Current ROI Tool"=8, "ROI Descriptor"={"Global Rectangle"=[], "Contours"=[]}, "Shift"=FALSE, "Alt"=FALSE} ("output cluster"), "Current ROI Tool"=w1854, "ROI Descriptor"=w1847, "Shift"=w1846, "Alt"=w1845) -> (w1849:T44)
                n713 = call "AlliGator Phasor Plot Display Mouse Down-Up Event Monitoring.vi"("Phasor Plot Display Event Registration"=w1859, "Phasor Plot Display Refnum"=w1857, "Look for Mouse Down(T)/Up(F)"=TRUE) -> ("Phasor Plot Display Event Registration"=w1858:refnum<event-registration>)  [unwired: 11 in, 1 out]
                n714 = Bundle By Name(cluster=w1855, "Phasor Plot Display Event"=w1858) -> (w1860:T26)
                n715 = Bundle By Name(cluster=T25 {"AlliGator Q Event"=enum."Phasor Plot:Mouse Up", "Data"=variant} ("AlliGator Actions out"), "Data"=w1849) -> (w1850:T25)
                n716 = Build Array(w1850) -> (w1848:T25[])
              }
            }
          }
        }
      }
      event Mouse Enter {
        # "Phasor Ratio Graph Tipstrip: Mouse Enter"
        n717 = event-data() -> ("CtlRef"=w1869:refnum<vi>)  [unwired: 1 in]
        n718 = Unbundle By Name(w1868) -> ("Phasor Ratio Graph Tipstrip Event"=w1870:refnum<event-registration>)
        n719 = call "Tipstrip Mouse Enter (XY Graph).vi"("Event Registration Refnum in"=w1870, "XYGraph Refnum"=w1869) -> ("Error Out"=w1863:errorcluster, "Event Registration Refnum out"=w1867:refnum<event-registration>)  [unwired: 8 in]
        n720 = Bundle By Name(cluster=w1868, "Phasor Ratio Graph Tipstrip Event"=w1867) -> (w1866:T26)
      }
      event Mouse Leave {
        # "Phasor Ratio Graph Tipstrip: Mouse Leave"
        n721 = event-data() -> ("CtlRef"=w1877:refnum<vi>)  [unwired: 1 in]
        n722 = Unbundle By Name(w1881) -> ("Phasor Ratio Graph Tipstrip Event"=w1879:refnum<event-registration>)
        n723 = control-ref of="Phasor Ratio Graph TipStrip"() -> (w1876:refnum<vi>)
        n724 = call "Tipstrip Mouse Leave (XY Graph).vi"("TipStrip Refnum"=w1876, "Event Registration Refnum in"=w1879, "XYGraph Refnum"=w1877) -> ("Error Out"=w1873:errorcluster, "Event Registration Refnum out"=w1878:refnum<event-registration>)  [unwired: 7 in]
        n725 = Bundle By Name(cluster=w1881, "Phasor Ratio Graph Tipstrip Event"=w1878) -> (w1880:T26)
      }
      event Mouse Move {
        # "Phasor Ratio Graph Tipstrip: Mouse Move"
        n726 = event-data() -> ("Time"=w1885:u32, "CtlRef"=w1895:refnum<vi>, "Coords"=w1894:T35)  [unwired: 1 in]
        n727 = Unbundle By Name(T25 {"AlliGator Q Event"=enum."Phasor Ratio:Tip Strip Update", "Data"=variant} ("Named Q Element")) -> ("AlliGator Q Event"=w1888:T24)
        n728 = Bundle By Name(cluster=T39 {"AlliGator Q Event"=enum."---- Files ----", "Time"=0, "Timeout"=0} ("output cluster"), "AlliGator Q Event"=w1888, "Time"=w1885, "Timeout"=w1882) -> (w1886:T39)
        n729 = call "AlliGator Filter Event.vi"("Filtered Event Data"=w1886) -> ("Filter Event?"=w1883:bool)  [unwired: 9 in, 1 out]
        n730 = case shown="False" w1883 {
          tunnel: w1895 -> [w1899 _]
          tunnel: w1894 -> [w1898 _]
          tunnel: [w1896 _] -> w1891
          frame False {
            n731 = control-ref of="Phasor Ratio Graph TipStrip"() -> (w1897:refnum<vi>)
            n732 = call "Set Plot TipStrip (XY Graph).vi"("TipStrip Refnum"=w1897, "Coords"=w1898, "XY Graph Refnum"=w1899) -> ("Error Out"=w1896:errorcluster)  [unwired: 6 in, 2 out]
          }
          frame True {
          }
        }
      }
      event Mouse Down {
        # "Source Image Display: Mouse Down"
        n733 = event-data() -> ("CtlRef"=w1911:refnum<vi>, "PlatMods.Shift"=w1910:bool, "PlatMods.Alt"=w1909:bool, "Button"=w1906:u16)  [unwired: 1 in]
        n734 = case shown="True" w1901 {
          tunnel: w1911 -> [_ w1919]
          tunnel: w1910 -> [_ w1918]
          tunnel: w1909 -> [_ w1917]
          tunnel: [w1912 w1916] -> w1908
          tunnel: w1907 -> [w1912 w1915]
          tunnel: w1906 -> [_ w1914]
          tunnel: [_ w1913] -> w1900
          frame False {
          }
          frame True {
            n735 = case shown="1" w1914 {
              tunnel: w1919 -> [_ w1921]
              tunnel: w1918 -> [_ _]
              tunnel: w1917 -> [_ _]
              tunnel: [w1920 w1925] -> w1916
              tunnel: w1915 -> [w1920 w1924]
              tunnel: [_ w1923] -> w1913
              frame 2, Default {
                # "Right Button"
              }
              frame 1 {
                # "Left Button"
                n736 = Unbundle By Name(w1924) -> ("Source Image Display Event"=w1927:refnum<event-registration>)
                n737 = call "AlliGator Source Image Display Mouse Down-Up Event Monitoring.vi"("Source Image Display Event Registration"=w1927, "Source Image Display Refnum"=w1921, "Look for Mouse Down(T)/Up(F)"=FALSE) -> ("Source Image Display Event Registration"=w1926:refnum<event-registration>, "Error Out"=w1923:errorcluster)  [unwired: 11 in]
                n738 = Bundle By Name(cluster=w1924, "Source Image Display Event"=w1926) -> (w1925:T26)
              }
            }
          }
        }
      }
      event Mouse Enter {
        # "Soure Image Display: Mouse Enter"
        n739 = event-data() -> ("CtlRef"=w1934:refnum<vi>)  [unwired: 1 in]
        n740 = case shown="True" w1928 {
          tunnel: [w1937 w1942] -> w1936
          tunnel: w1935 -> [w1937 w1941]
          tunnel: w1934 -> [_ w1939]
          tunnel: [_ w1938] -> w1929
          frame False {
          }
          frame True {
            n741 = Unbundle By Name(w1941) -> ("Source Image Display Event"=w1943:refnum<event-registration>)
            n742 = register-events(reference=w1943, T34 refnum ("event source"), w1939, w1939, w1939) -> (reference out=w1944:refnum<event-registration>, error out=w1938:errorcluster)  [unwired: 2 in]
            n743 = Bundle By Name(cluster=w1941, "Source Image Display Event"=w1944) -> (w1942:T26)
          }
        }
      }
      event Mouse Leave {
        # "Source Image Display: Mouse Leave"
        n744 = event-data() -> ("CtlRef"=w1950:refnum<vi>)  [unwired: 1 in]
        n745 = case shown="True" w1951 {
          tunnel: [w1954 w1960] -> w1953
          tunnel: w1952 -> [w1954 w1959]
          tunnel: w1950 -> [_ w1958]
          tunnel: [_ w1956] -> w1945
          frame False {
          }
          frame True {
            w1957 = FALSE ("Visible")
            w1955 = refnum<vi> refnum ("event source")
            n746 = Unbundle By Name(w1959) -> ("Source Image Display Event"=w1961:refnum<event-registration>)
            n747 = register-events(reference=w1961, w1958, w1955, w1955, w1955, w1955) -> (reference out=w1962:refnum<event-registration>, error out=w1956:errorcluster)  [unwired: 1 in]
            n748 = Bundle By Name(cluster=w1959, "Source Image Display Event"=w1962) -> (w1960:T26)
            n749 = property on="Phasor Plot Phase Lifetime" class="DigNum (strict)"("Visible"=w1957) -> ()  [unwired: 2 in, 2 out]
            n750 = property on="Phasor Plot Phasor Ratio" class="DigNum (strict)"("Visible"=w1957) -> ()  [unwired: 2 in, 2 out]
            n751 = property on="Phasor at cursor (g, s)" class="Clust (strict)"("Visible"=w1957) -> ()  [unwired: 2 in, 2 out]
            n752 = property on="Phasor at cursor (m, phi)" class="Clust (strict)"("Visible"=w1957) -> ()  [unwired: 2 in, 2 out]
            n753 = property on="Phasor Plot Modulus Lifetime" class="DigNum (strict)"("Visible"=w1957) -> ()  [unwired: 2 in, 2 out]
            n754 = property on="Phasor Plot Average Lifetime" class="DigNum (strict)"("Visible"=w1957) -> ()  [unwired: 2 in, 2 out]
          }
        }
      }
      event Mouse Move {
        # "Source Image Display: Mouse Move"
        n755 = event-data() -> ("Time"=w1964:u32, "CtlRef"=w1975:refnum<vi>, "Coords"=w1974:T35)  [unwired: 1 in]
        n756 = call-poly <vilib>:"Acquire Input Data.vi"("device ID"=w1966, "error in (no error)"=w1969) -> ("device ID"=w1967:refnum<k1>, "keys pressed"=w1965:T49, "error out"=w1968:errorcluster)  [unwired: 15 in]
        n757 = case shown="True" w1970 {
          tunnel: w1975 -> [_ w1989]
          tunnel: w1974 -> [_ _]
          tunnel: [_ w1987] -> w1971
          tunnel: w1965 -> [_ w1988]
          tunnel: w1964 -> [_ w1977]
          tunnel: w1963 -> [_ w1976]
          frame False {
          }
          frame True {
            w1982 = T25 {"AlliGator Q Event"=enum."Image:Mouse Move", "Data"=variant} ("AlliGator Events")
            n758 = Unbundle By Name(w1982) -> ("AlliGator Q Event"=w1985:T24)
            n759 = property on="Source Image" class="ImageControl"() -> (error out=w1986:errorcluster, "ROI"=w1991:T57)  [unwired: 2 in, 1 out]
            n760 = call "is ROI Empty.vi"("Current ROI Descriptor"=w1991) -> ("Empty ROI?"=w1990:bool)  [unwired: 8 in]
            n761 = Bundle By Name(cluster=T39 {"AlliGator Q Event"=enum."---- Files ----", "Time"=0, "Timeout"=0} ("output cluster"), "AlliGator Q Event"=w1985, "Timeout"=w1976, "Time"=w1977) -> (w1983:T39)
            n762 = case shown="False" w1990 {
              tunnel: w1991 -> [w2009 _]
              tunnel: w1986 -> [w2008 _]
              frame False {
                n763 = property on="Decay Fit Parameter Map Image" class="ImageControl"(error in=w2008, "ROI"=w2009) -> ()  [unwired: 1 in, 2 out]
              }
              frame True {
              }
            }
            n764 = call "AlliGator Filter Event.vi"("Filtered Event Data"=w1983) -> ("Filter Event?"=w1979:bool)  [unwired: 9 in, 1 out]
            n765 = call "AlliGator Source Image Display Mouse Move Flag.vi"("Read/Write"=Read-Write."Read") -> ("Flag (out)"=w1980:bool)  [unwired: 8 in]
            n766 = Or(x=w1980, y=w1979) -> (x .or. y?=w1978:bool)
            n767 = case shown="False" w1978 {
              tunnel: w1989 -> [w1996 _]
              tunnel: w1988 -> [w1995 _]
              tunnel: [w1992 _] -> w1987
              tunnel: w1982 -> [w1993 _]
              frame False {
                n768 = local read "Tab Control"() -> (w1994:T3)
                n769 = case shown="\"Phasor Plot\"" w1994 {
                  tunnel: w1996 -> [_ w2007]
                  tunnel: w1995 -> [_ w2003]
                  tunnel: w1993 -> [_ w2001]
                  tunnel: [_ w1997] -> w1992
                  frame "Image Histogram", Default {
                  }
                  frame "Phasor Plot" {
                    # "If the Phasor Plot Tab is visible,"
                    n770 = property class="ImageControl"(reference=w2007) -> (reference out=w2006:refnum<vi>, "Last Mouse Position"=w2004:cluster{"X":i32, "Y":i32})  [unwired: 1 in, 1 out]
                    n771 = call "AlliGator Source Image Display Mouse Move Flag.vi"("Flag (in)"=TRUE, "Read/Write"=Read-Write."Write") -> ()  [unwired: 7 in, 1 out]
                    n772 = Bundle By Name(cluster=T43 {"Image Control Refnum"=refnum, "Coords"={"Horizontal"=0, "Vertical"=0}, "button info"={"button 1"=FALSE, "button 2"=FALSE, "button 3"=FALSE, "button 4"=FALSE}, "keys pressed"=[]} ("Image User Event Data"), "Image Control Refnum"=w2006, "Coords"=w2004, "keys pressed"=w2003) -> (w2002:T43)
                    n773 = Bundle By Name(cluster=w2001, "Data"=w2002) -> (w1998:T25)
                    n774 = Build Array(w1998) -> (w1997:T25[])
                  }
                }
              }
              frame True {
              }
            }
          }
        }
      }
      event Mouse Up {
        # "Source Image Display: Mouse Up"
        n775 = event-data() -> ("CtlRef"=w2021:refnum<vi>, "PlatMods.Shift"=w2012:bool, "PlatMods.Alt"=w2011:bool)  [unwired: 1 in]
        n776 = case shown="True" w2013 {
          tunnel: w2021 -> [_ w2025]
          tunnel: w2020 -> [w2022 w2026]
          tunnel: [w2022 w2027] -> w2019
          tunnel: [_ w2037] -> w2014
          tunnel: w2012 -> [_ w2033]
          tunnel: w2011 -> [_ w2032]
          tunnel: [_ w2023] -> w2010
          frame False {
          }
          frame True {
            n777 = property class="ImageControl"(reference=w2025) -> (error out=w2024:errorcluster, "Current ROI Tool"=w2035:u32, "ROI"=w2034:T57)  [unwired: 1 in, 1 out]
            n778 = Unbundle By Name(w2026) -> ("Source Image Display Event"=w2030:refnum<event-registration>)
            n779 = Bundle(cluster=T44 {"Current ROI Tool"=8, "ROI Descriptor"={"Global Rectangle"=[], "Contours"=[]}, "Shift"=FALSE, "Alt"=FALSE} ("output cluster"), "Current ROI Tool"=w2035, "ROI Descriptor"=w2034, "Shift"=w2033, "Alt"=w2032) -> (w2031:T44)
            n780 = call "AlliGator Source Image Display Mouse Down-Up Event Monitoring.vi"("Source Image Display Event Registration"=w2030, "Source Image Display Refnum"=w2025, "Error In"=w2024, "Look for Mouse Down(T)/Up(F)"=TRUE) -> ("Source Image Display Event Registration"=w2029:refnum<event-registration>, "Error Out"=w2023:errorcluster)  [unwired: 10 in]
            n781 = Bundle By Name(cluster=T25 {"AlliGator Q Event"=enum."Image:Mouse Up", "Data"=variant} ("AlliGator Actions out"), "Data"=w2031) -> (w2038:T25)
            n782 = Bundle By Name(cluster=w2026, "Source Image Display Event"=w2029) -> (w2027:T26)
            n783 = Build Array(w2038) -> (w2037:T25[])
          }
        }
      }
      event Mouse Down {
        # "Time Point Slider: Mouse Down"
        n784 = event-data() -> ("CtlRef"=w2045:refnum<vi>)  [unwired: 1 in]
        n785 = case shown="True" w2046 {
          tunnel: [w2049 w2054] -> w2048
          tunnel: w2047 -> [w2049 w2053]
          tunnel: w2045 -> [_ w2052]
          tunnel: [_ w2051] -> w2040
          frame False {
          }
          frame True {
            w2050 = refnum<vi> refnum ("event source")
            n786 = Unbundle By Name(w2053) -> ("Time Point Slider Event"=w2055:refnum<event-registration>)
            n787 = register-events(reference=w2055, w2050, w2052, w2052, w2050) -> (reference out=w2056:refnum<event-registration>, error out=w2051:errorcluster)  [unwired: 1 in]
            n788 = Bundle By Name(cluster=w2053, "Time Point Slider Event"=w2056) -> (w2054:T26)
          }
        }
      }
      event Mouse Move {
        # "Time Point Slider: Mouse Move"
        n789 = event-data() -> ("CtlRef"=w2062:refnum<vi>, "Time"=w2058:u32)  [unwired: 1 in]
        n790 = case shown="True" w2065 {
          tunnel: w2062 -> [_ w2074]
          tunnel: [_ w2073] -> w2059
          tunnel: w2058 -> [_ w2070]
          tunnel: w2057 -> [_ w2066]
          frame False {
          }
          frame True {
            w2072 = T25 {"AlliGator Q Event"=enum."GUI:Time Series Slider Moved", "Data"=variant} ("Time-Gated Phasor Q Element")
            n791 = Unbundle By Name(w2072) -> ("AlliGator Q Event"=w2071:T24)
            n792 = Bundle By Name(cluster=T39 {"AlliGator Q Event"=enum."---- Files ----", "Time"=0, "Timeout"=0} ("output cluster"), "AlliGator Q Event"=w2071, "Time"=w2070, "Timeout"=w2066) -> (w2068:T39)
            n793 = call "AlliGator Filter Event.vi"("Filtered Event Data"=w2068) -> ("Filter Event?"=w2067:bool)  [unwired: 9 in, 1 out]
            n794 = case shown="False" w2067 {
              tunnel: w2074 -> [w2078 _]
              tunnel: [w2076 _] -> w2073
              tunnel: w2072 -> [w2075 _]
              frame False {
                n795 = property class="Slide (strict)"(reference=w2078) -> ("Value"=w2077:u16)  [unwired: 1 in, 2 out]
                n796 = Bundle By Name(cluster=w2075, "Data"=w2077) -> (w2079:T25)
                n797 = Build Array(w2079) -> (w2076:T25[])
              }
              frame True {
              }
            }
          }
        }
      }
      event Mouse Up; Mouse Leave {
        # "Time Point Slider: Mouse Up, Mouse Leave"
        n798 = event-data() -> ("CtlRef"=w2086:refnum<vi>)  [unwired: 1 in]
        n799 = case shown="True" w2087 {
          tunnel: [w2090 w2101] -> w2089
          tunnel: w2088 -> [w2090 w2100]
          tunnel: w2086 -> [_ w2094]
          tunnel: [_ w2092] -> w2081
          tunnel: [_ w2091] -> w2080
          frame False {
          }
          frame True {
            w2097 = refnum<vi> refnum ("event source")
            n800 = property class="Slide (strict)"(reference=w2094) -> ("Value"=w2093:u16)  [unwired: 1 in, 2 out]
            n801 = Unbundle By Name(w2100) -> ("Time Point Slider Event"=w2099:refnum<event-registration>)
            n802 = register-events(reference=w2099, w2094, w2097, w2097, w2097) -> (reference out=w2098:refnum<event-registration>, error out=w2092:errorcluster)  [unwired: 1 in]
            n803 = Bundle By Name(cluster=T25 {"AlliGator Q Event"=enum."GUI:Time Series Slider Changed", "Data"=variant} ("Time-Gated Phasor Q Element"), "Data"=w2093) -> (w2095:T25)
            n804 = Build Array(w2095) -> (w2091:T25[])
            n805 = Bundle By Name(cluster=w2100, "Time Point Slider Event"=w2098) -> (w2101:T26)
          }
        }
      }
      event Menu Activation? {
        n806 = event-data() -> ("MenuRef"=w2110:refnum<k9>)  [unwired: 1 in]
        n807 = case shown="True" w2109 {
          tunnel: w2110 -> [_ w2118]
          tunnel: [_ w2117] -> w2104
          tunnel: w2103 -> [_ w2116]
          tunnel: w2102 -> [_ w2114]
          frame False {
          }
          frame True {
            n808 = Strip Path(path=w2114) -> (stripped path=w2113:path)  [unwired: 1 out]
            n809 = Build Path(base path=w2113, name or relative path=path "AlliGator.rtm") -> (appended path=w2111:path)
            n810 = property class="VI"(reference=w2116, "RT Menu Path"=w2111) -> (error out=w2115:errorcluster)  [unwired: 1 in, 1 out]
            n811 = call "AlliGator Update Menu.vi"("Error In"=w2115, "Menu in"=w2118) -> ("Error Out"=w2117:errorcluster)  [unwired: 9 in]
          }
        }
        n812 = event-data() -> ()  [unwired: 2 in, 1 out]
      }
      event Menu Selection (User) {
        n813 = event-data() -> ("MenuRef"=w2130:refnum<k9>, "ItemPath"=w2129:string, "ItemTag"=w2124:string)  [unwired: 1 in]
        n814 = call-poly <vilib>:"Acquire Input Data.vi"("device ID"=w2143, "error in (no error)"=w2142) -> ("device ID"=w2140:refnum<k1>, "keys pressed"=w2139:T49, "error out"=w2141:errorcluster)  [unwired: 15 in]
        n815 = Index Array(array=w2139) -> (element=w2123:T32)  [unwired: 1 in]
        n816 = property on="Time Point Slide" class="Slide (strict)"() -> ("Visible"=w2128:bool)  [unwired: 2 in, 2 out]
        n817 = Select(t=w2124, s=w2134, f=w2147) -> (s? t:f=w2122:string)
        n818 = Equal?(x=w2123, y=T32."H" ("element")) -> (x = y?=w2121:bool)
        n819 = call "AlliGator Menu Items.vi"("Menu Item Tag"=w2124, "This VI"=w2127) -> ("Error Out"=w2132:errorcluster, "Message"=w2136:string, "Window opened?"=w2125:bool, "AlliGator Actions"=w2120:T25[])  [unwired: 6 in]
        n820 = call "AlliGator Conditional Menu Items.vi"("Dataset Series?"=w2128, "Help?"=w2121, "Menu Item Path"=w2129, "Menu Item Tag"=w2122, "menu reference"=w2130) -> ("Error Out"=w2133:errorcluster, "Quit?"=w2137:bool, "Message"=w2119:string, "AlliGator Actions"=w2138:T25[])  [unwired: 3 in]
        n821 = Concatenate Strings(w2119, w2136) -> (w2135:string)
        n822 = Build Array (concatenate)(w2138, w2120) -> (w2126:T25[])
        n823 = Select(t=w2133, s=w2134, f=w2132) -> (s? t:f=w2131:errorcluster)
        n824 = global write "AlliGator Globals.vi" "Window Just Opened"(w2125) -> ()
      }
      event "Current ROI Analysis": Value Change {
        n825 = event-data() -> ()  [unwired: 1 in, 1 out]
        n826 = case shown="True" w2148 {
          tunnel: [_ T25[] [{"AlliGator Q Event"=enum."FLI Dataset:ROI Analysis", "Data"=variant}] ("element")] -> w2149
          frame False {
          }
          frame True {
          }
        }
      }
      event "Phasor ROI Decay": Value Change {
        n827 = event-data() -> ()  [unwired: 1 in, 1 out]
        n828 = case shown="True" w2155 {
          tunnel: [_ T25[] [{"AlliGator Q Event"=enum."Phasor Plot:Compute Decay of Selected Phasors", "Data"=variant}] ("element")] -> w2156
          frame False {
          }
          frame True {
          }
        }
      }
      event Mouse Enter {
        # "Note: when dragging and dropping a file in the window, the \"Mouse Enter\" is not triggered, therefore this event is triggered for all other user actions, EXCEPT for drag & dropping"
        # "Makes File/Folder Path invisible to allow normal user interaction"
        n829 = event-data() -> ()  [unwired: 1 in, 1 out]
        n830 = call "AlliGator Hide Path Drop Boxes.vi"("Hide (F)/Show"=FALSE, "AlliGator Ctrl Refnums"=w2163) -> ()  [unwired: 9 in, 1 out]
      }
      event Mouse Leave {
        (unwired) FALSE
        # "If the user moves away from the window, we can show the (transparent) path control to allow the user to drag & drop a file in it."
        # "Makes File/Folder Path visible (but transparent) to allow the user to drop a file in the window"
        n831 = event-data() -> ()  [unwired: 1 in, 1 out]
        n832 = global read "AlliGator Globals.vi" "Window Just Opened"() -> (w2172:bool)
        n833 = Not(x=w2172) -> (.not. x?=w2169:bool)
        n834 = call "AlliGator Hide Path Drop Boxes.vi"("Hide (F)/Show"=w2169, "AlliGator Ctrl Refnums"=w2168) -> ()  [unwired: 9 in, 1 out]
        n835 = And(x=w2169, y=FALSE ("Mouse Leave")) -> (x .and. y?=w2170:bool)
        n836 = global write "AlliGator Globals.vi" "Window Just Opened"(w2170) -> ()
      }
      event Panel Close? {
        n837 = event-data() -> ()  [unwired: 1 in, 1 out]
        n838 = case shown="True" w2184 {
          tunnel: [_ w2189] -> w2178
          tunnel: w2183 -> [_ w2188]
          tunnel: [_ w2187] -> w2177
          frame False {
            n839 = One Button Dialog(message="First abort the current operation...") -> ()  [unwired: 1 in, 1 out]
            n840 = call "Play Error Sound.vi"() -> ()  [unwired: 27 in, 1 out]
          }
          frame True {
            n841 = call "AlliGator Quit Dialog.vi"("App name"=w2188) -> ("Quit?"=w2187:bool, "AlliGator Actions"=w2189:T25[])  [unwired: 9 in]
          }
        }
        n842 = event-data("Discard?"=TRUE) -> ()  [unwired: 1 in, 1 out]
      }
    }
    n843 = call "AlliGator Settings Storage.vi"("AlliGator Settings List"=AlliGator_Settings_List."Miscellaneous:Verbose Error Mode") -> ("Variant Data out"=w182:variant)  [unwired: 9 in, 1 out]
    n844 = call-poly "Variant to Data.vi"("Variant"=w182) -> ("Value"=w180:bool)  [unwired: 8 in]
    n845 = call "Message Style.vi"() -> ("Message Formatting"=w176:T58)
    n846 = call "Send Message to Notebook.vi"("Text Formatting"=w176, "Error In"=w175, "Message"=w172, "Notebook Queue"=w168) -> ("Error Out"=w174:errorcluster, "Notebook Queue"=w173:refnum<queue>)  [unwired: 4 in]
    n847 = call "AlliGator Queue Non Empty Events.vi"("Actions"=w177, "AlliGator Q"=w169) -> ()  [unwired: 9 in, 1 out]
    n848 = call "Send Error to Notebook.vi"("error in (no error)"=w174, "Verbose Error Messages (T)"=w180, "State Machine Case Error Source"="Event Loop", "Notebook Q"=w173) -> ()  [unwired: 7 in, 1 out]
  }
  n849 = call <vilib>:"Simple Error Handler.vi"("error in (no error)"=w37) -> ()  [unwired: 4 in, 5 out]
  n850 = for {
    N: 10 -> [_]
    tunnel: [w2191] -> w53 mode=indexing
    tunnel: T14."Parameter Map" ("Tab Control") -> [w2190]
    i -> [w2192]
    n851 = Coerce To Type(0:w2192, 1:w2190) -> (2:w2191:T14)
  }
  n852 = call "Destroy Embedded Progress Bar.vi"("Error In"=w34, "Progress Bar Queue in"=w33) -> ()  [unwired: 9 in, 1 out]
  n853 = for {
    tunnel: w53 -> [w2193] mode=indexing
    n854 = case shown="\"Parameter Map\"" w2193 {
      frame "Image Histogram" {
      }
      frame "Fluorescence Decay", Default {
      }
      frame "Fluorescence Decay Statistics" {
      }
      frame "Intensity Time Trace" {
      }
      frame "Phasor Plot" {
        n855 = property on="Phasor Plot ROI Color" class="ColBox"("Val(Sgnl)"="Phasor Plot ROI Color") -> ()  [unwired: 2 in, 2 out]
      }
      frame "Phasor Graph" {
      }
      frame "Phasor Ratio" {
      }
      frame "Lifetime & Other Parameters" {
      }
      frame "Decay Fit Parameters Map" {
        n856 = property on="Decay Fit Parameter Map Color Scale" class="ColRmp (strict)"("Scale.FormatString"="%.3g" ("Scale.Format String")) -> ()  [unwired: 2 in, 2 out]
        n857 = property on="Decay Fit Parameter Map ROI Color" class="ColBox"("Val(Sgnl)"="Decay Fit Parameter Map ROI Color") -> ()  [unwired: 2 in, 2 out]
      }
      frame "Parameter Map" {
        n858 = property on="Parameter Map Color Scale" class="ColRmp (strict)"("Scale.FormatString"="%.3g" ("Scale.Format String")) -> ()  [unwired: 2 in, 2 out]
        n859 = property on="Parameter Map ROI Color" class="ColBox"("Val(Sgnl)"="Parameter Map ROI Color") -> ()  [unwired: 2 in, 2 out]
      }
    }
  }
  n860 = flat-sequence {
    frame #0 {
      n861 = property on="Source Image ROI Color" class="ColBox"("Val(Sgnl)"="Source Image ROI Color") -> ()  [unwired: 2 in, 2 out]
      n862 = property on="Image Color Scale" class="ColRmp (strict)"("Scale.Format"=u8 8 ("Scale.Display Format:Format"), "Scale.Precision"=u8 1 ("Scale.Display Format:Precision")) -> ()  [unwired: 2 in, 2 out]
    }
  }
  n863 = call-poly <vilib>:"Close Input Device.vi"("error in (no error)"=w135, "device ID"=w136) -> ("error out"=w49:errorcluster)  [unwired: 8 in]
  n864 = call-poly <vilib>:"Close Input Device.vi"("error in (no error)"=w115, "device ID"=w114) -> ("error out"=w48:errorcluster)  [unwired: 8 in]
  n865 = Unregister For Events(event registration refnum=w154) -> (error out=w57:errorcluster)  [unwired: 1 in]
  n866 = Merge Errors(w57, w49, w48) -> (w42:errorcluster)
  n867 = call "Clear Error.vi"("Error In"=w42) -> ("no Error Out"=w41:errorcluster)  [unwired: 8 in]
  n868 = invoke class="VI" method="FP.Close"(reference=w30, error in=w41) -> ()  [unwired: 1 in, 3 out]
